vi "Q14070-Z060B.vi"() -> ()   [LabVIEW 2013]
uses:
  <vilib>/Utility/file.llb/Read From Spreadsheet File (string).vi
  <vilib>/express/express arith-compare/Formula/XNode/ExpressFormulaBlockNode.xnode
  PCI8622_32.dll
  <vilib>/printing/EasyPrintingControls.llb/contents.ctl
  <vilib>/Utility/NIReport.llb/NI_ReportGenerationCore.lvlib
  <vilib>/printing/EasyPrintingControls.llb/report_type.ctl
  <vilib>/Utility/NIReport.llb/NI_report.lvclass
  <vilib>/printing/EasyPrinting.llb/Easy Print VI Panel or Documentation (path).vi
panel:
  out "齿条跑和右极限":dbl format="%#.3f"
  out "齿条跑和左极限":dbl format="%#.3f"
  out "左轴向力数组大小":i32
  in  "电动缸快速":dbl=15.0
  in  "电动缸慢速":dbl=1.0
  out "最大轴向力标准(N)":dbl=200.0 caption="L+Lmax(mm)" format="%#.3f"
  out "循环退出":bool
  in  "?":bool
  in  "密码":string
  in  "?":bool
  in  "?":bool
  in  "截取百分比":dbl=0.05
  in  "半行程":dbl=70.0
  in  "是否取消放行按钮":bool
  out "PLC":bool
  out "齿条传动比":dbl=200.0 caption="L+Lmax(mm)" format="%#.3f"
  out "右平均轴向力(N)":dbl caption="L+Lmax(mm)" format="%#.3f"
  out "左平均轴向力(N)":dbl caption="最大位移偏离Lmax(mm)" format="%#.3f"
  in  "确定按钮":bool
  out "员工ID":string
  in  "出支线工步号":dbl
  out "报警提示":string
  in  "报警工步号":dbl
  out "急停":bool
  out "DeviceHandle":u32
  in  "轴向力设定次数":dbl=5.0
  in  "最小间隙(mm)":dbl=0.0005 format="%#.3f"
  out "本备料状态H":bool
  out "本测试状态H":bool
  out "本自动状态H":bool
  out "夹头松开":bool
  out "测头右位":bool
  out "测头左位":bool
  in  "测头气缸右移":bool
  in  "测头气缸左移":bool
  in  "轴向力已做次数":dbl
  out "轴向力及全行程间隙合格":bool
  out "轴向力启动":bool
  out "间隙启动":bool
  out "夹头夹紧位":bool
  in  "夹头松开":bool
  in  "夹头夹紧":bool
  out "找帽扭矩":dbl=5.0 caption="压力传感器" format="%#.2f"
  out "error out":errorcluster
  out "型号数量":i32
  out "error out 4":errorcluster
  in  "间隙设定调整次数":dbl=5.0
  out "读取产品ID":string
  in  "本备料状态":bool
  in  "本测试状态":bool
  in  "本自动状态":bool
  out "FGCS":string
  out "KSJJ":string
  out "Z060BRFID":string
  out "轴向力Y":dbl[](array[numeric])
  out "轴向力X":dbl[](array[numeric])
  out "间隙X数组":dbl[](array[numeric])
  out "间隙Y数组":dbl[](array[numeric])
  out "error out 3":errorcluster caption="错误输出"
  out "rfid工步号":u32
  out "芯片ID":string="201209190001"
  out "rfid完成":bool
  out "rfid触发":bool
  out "本序已做":bool
  in  "回零完成":bool
  in  "电动缸回零":bool
  in  "单点间隙已调试次数":dbl
  in  "需调整角度(度)":dbl
  in  "转向器中心":dbl
  out "扭矩到达":bool
  out "黄灯":bool
  out "红灯":bool
  out "基准位移":dbl caption="压力传感器" format="%#.4f"
  out "上序不合格":bool
  out "单点间隙合格":bool
  out "上序合格":bool
  out "测头机构电机":u32
  out "复位":bool
  in  "型号选择":u16(ring)=2 items=["J709", "J728", "J706"]
  in  "联线按钮":bool
  in  "工步号":u32
  in  "产品ID":string="201209190001"
  out "间隙位移(mm)":dbl=-4.6787895475327215 caption="压力传感器" format="%#.3f"
  out "齿条推拉力(N)":dbl format="%#.2f"
  out "齿条扭矩(Nm)":dbl format="%#.2f"
  out "通讯状态":bool
  out "员工姓名":string
  out "工步提示":string
  out "ADODB._Connection Out 2":refnum<k7>
  out "旋转齿条电机":u32
  out "电动缸电机":u32
  in  "停止":bool
  in  "参数加载":bool
  in  "选项卡控件":T1(tab)
  out "180°外全行程间隙标准(mm)":dbl=0.1 format="%#.3f"
  out "扭动曲线":cluster{"Y":dbl[], "Y":dbl[]}[](graph) caption="压球涨堵头1"
  out "中间位置间隙":dbl caption="间隙值L(mm)" format="%#.3f"
  out "中间位置最大间隙标准(mm)":dbl=0.07 format="%#.3f"
  out "右180°外全行程间隙":dbl caption="正向最大间隙L1(mm)" format="%#.3f"
  out "左180°外全行程间隙":dbl caption="正向最大间隙L1(mm)" format="%#.3f"
  out "右180°内全行程间隙":dbl caption="正向最大间隙L1(mm)" format="%#.3f"
  out "左180°内全行程间隙":dbl caption="正向最大间隙L1(mm)" format="%#.3f"
  out "180°内全行程间隙标准(mm)":dbl=0.07 format="%#.3f"
  in  "找帽OK":bool
  out "左全行程间隙":dbl caption="正向最大间隙L1(mm)" format="%#.3f"
  out "右全行程间隙":dbl caption="正向最大间隙L1(mm)" format="%#.3f"
  out "总圈数最大值":dbl
  out "总圈数标准":dbl
  out "总行程最大值":dbl
  out "总行程标准(mm)":dbl
  out "力波动标准(N)":dbl=60.0 caption="L+Lmax(mm)" format="%#.3f"
  out "轴向力标准(N)":dbl=100.0 caption="L+Lmax(mm)" format="%#.3f"
  out "右轴向力波动(N)":dbl caption="L+Lmax(mm)" format="%_4g"
  out "右最大轴向力(N)":dbl caption="L+Lmax(mm)" format="%_4g"
  out "左轴向力波动(N)":dbl caption="最大位移偏离Lmax(mm)" format="%_4g"
  out "左最大轴向力(N)":dbl caption="最大位移偏离Lmax(mm)" format="%_4g"
  out "行程跳动曲线":cluster{"Y":dbl[], "Y":dbl[]}[](graph) caption="压球涨堵头1"
  out "平均轴向力标准(N) max":dbl=200.0 caption="L+Lmax(mm)" format="%#.3f"
  out "总行程":dbl format="%_4g"
  out "总圈数":dbl format="%_4g"
  in  "不合格品":bool
  in  "扭矩停止值":dbl=16.0
  in  "齿条右极限":dbl=-70.0 caption="压力传感器" format="%#.2f"
  in  "齿条左极限":dbl=-262.0 caption="压力传感器" format="%#.2f"
  in  "齿条移动速度":dbl=5.0 caption="压力传感器" format="%#.2f"
  in  "旋转齿条轴找帽转速":dbl=5.0 caption="压力传感器" format="%#.2f"
  in  "测量点扭矩":dbl=4.0 caption="压力传感器" format="%#.2f"
  in  "旋转齿条轴测量转速":dbl caption="压力传感器" format="%#.2f"
  in  "测头机构轴后退位":dbl=30.0 caption="压力传感器" format="%#.2f"
  in  "测头机构轴待检位":dbl caption="压力传感器" format="%#.2f"
  in  "测头机构轴检测位":dbl caption="压力传感器" format="%#.2f"
  in  "测头机构轴移动速度":dbl caption="压力传感器" format="%#.2f"
  in  "机械间隙值":dbl=3.5
  in  "阻挡":bool
  in  "放行":bool
  in  "夹头松开":bool
  in  "夹头夹紧":bool
  in  "测头气缸右移":bool
  in  "测头气缸左移":bool
  in  "支线下降":bool
  in  "支线顶升":bool
  in  "出支线":bool
  in  "进支线":bool
  in  "主线下降":bool
  in  "主线顶升":bool
  in  "下阻挡器放行":bool
  in  "上阻挡器放行":bool
  in  "测头机构轴使能":bool
  in  "测头机构轴后退":bool
  in  "测头机构轴前进":bool
  in  "电动缸速度(mm/s)":dbl=10.0 format="%#.3f"
  out "电动缸位置(mm)":dbl format="%#.3f"
  in  "旋转齿条轴速度(°/s)":dbl=10.0 format="%#.3f"
  out "旋转齿条轴位置(°)":dbl format="%#.3f"
  in  "测头机构轴速度(mm/s)":dbl=10.0 format="%#.3f"
  out "测头机构轴位置(mm)":dbl format="%#.3f"
  in  "旋转齿条轴右转":bool
  in  "旋转齿条轴左转":bool
  in  "旋转齿条轴使能":bool
  in  "电动缸后退":bool
  in  "电动缸使能":bool
  in  "电动缸前进":bool
  in  "齿条扭矩比例偏移":dbl=1.0 format="%#.2f"
  in  "齿条扭矩零点偏移":dbl format="%#.2f"
  in  "齿条推拉力比例偏移":dbl=1.0 format="%#.2f"
  in  "齿条推拉力零点偏移":dbl format="%#.2f"
  in  "间隙位移比例偏移":dbl=1.0 format="%#.2f"
  in  "间隙位移零点偏移":dbl format="%#.2f"
  in  "传感器参数保存":bool
  in  "参数修改":bool
  in  "参数查询":bool
  in  "参数浏览表":string[][](table)
  # "芜湖机械转向器装配线"
  # "间隙及轴向力检测"
  # "湖北唯思凌科装备制造有限公司 设计开发 (C)2015"
  # "Q14070机械转向器装配线"
  # "≤"
  # "间隙测量结果"
  # "间隙测量判定值"
  # "≤"
  # "≤"
  # "≤"
  # "轴向力测量结果"
  # "轴向力测量标准"
  # "≥"
  # "≤"
  # "≥"
  # "≤"
  # "≤"
  # "≥"
  # "不得大于20NM"
  # "传感器校验区"
  # "关于传感器校验：\n1、传感器校验需要由具备资质的单位或部门进行校验。\n2、具备权限的用户才能够修改传感器校验参数和试验参数。\n3、修改校验参数方法：先将比例偏移置为1，修改零点偏移，使零点值与校验的传感器一致；然后根据增幅调整比例偏移。"
  # "注意：\n具备权限的用户才能够修改传感器校验参数和试验参数！"
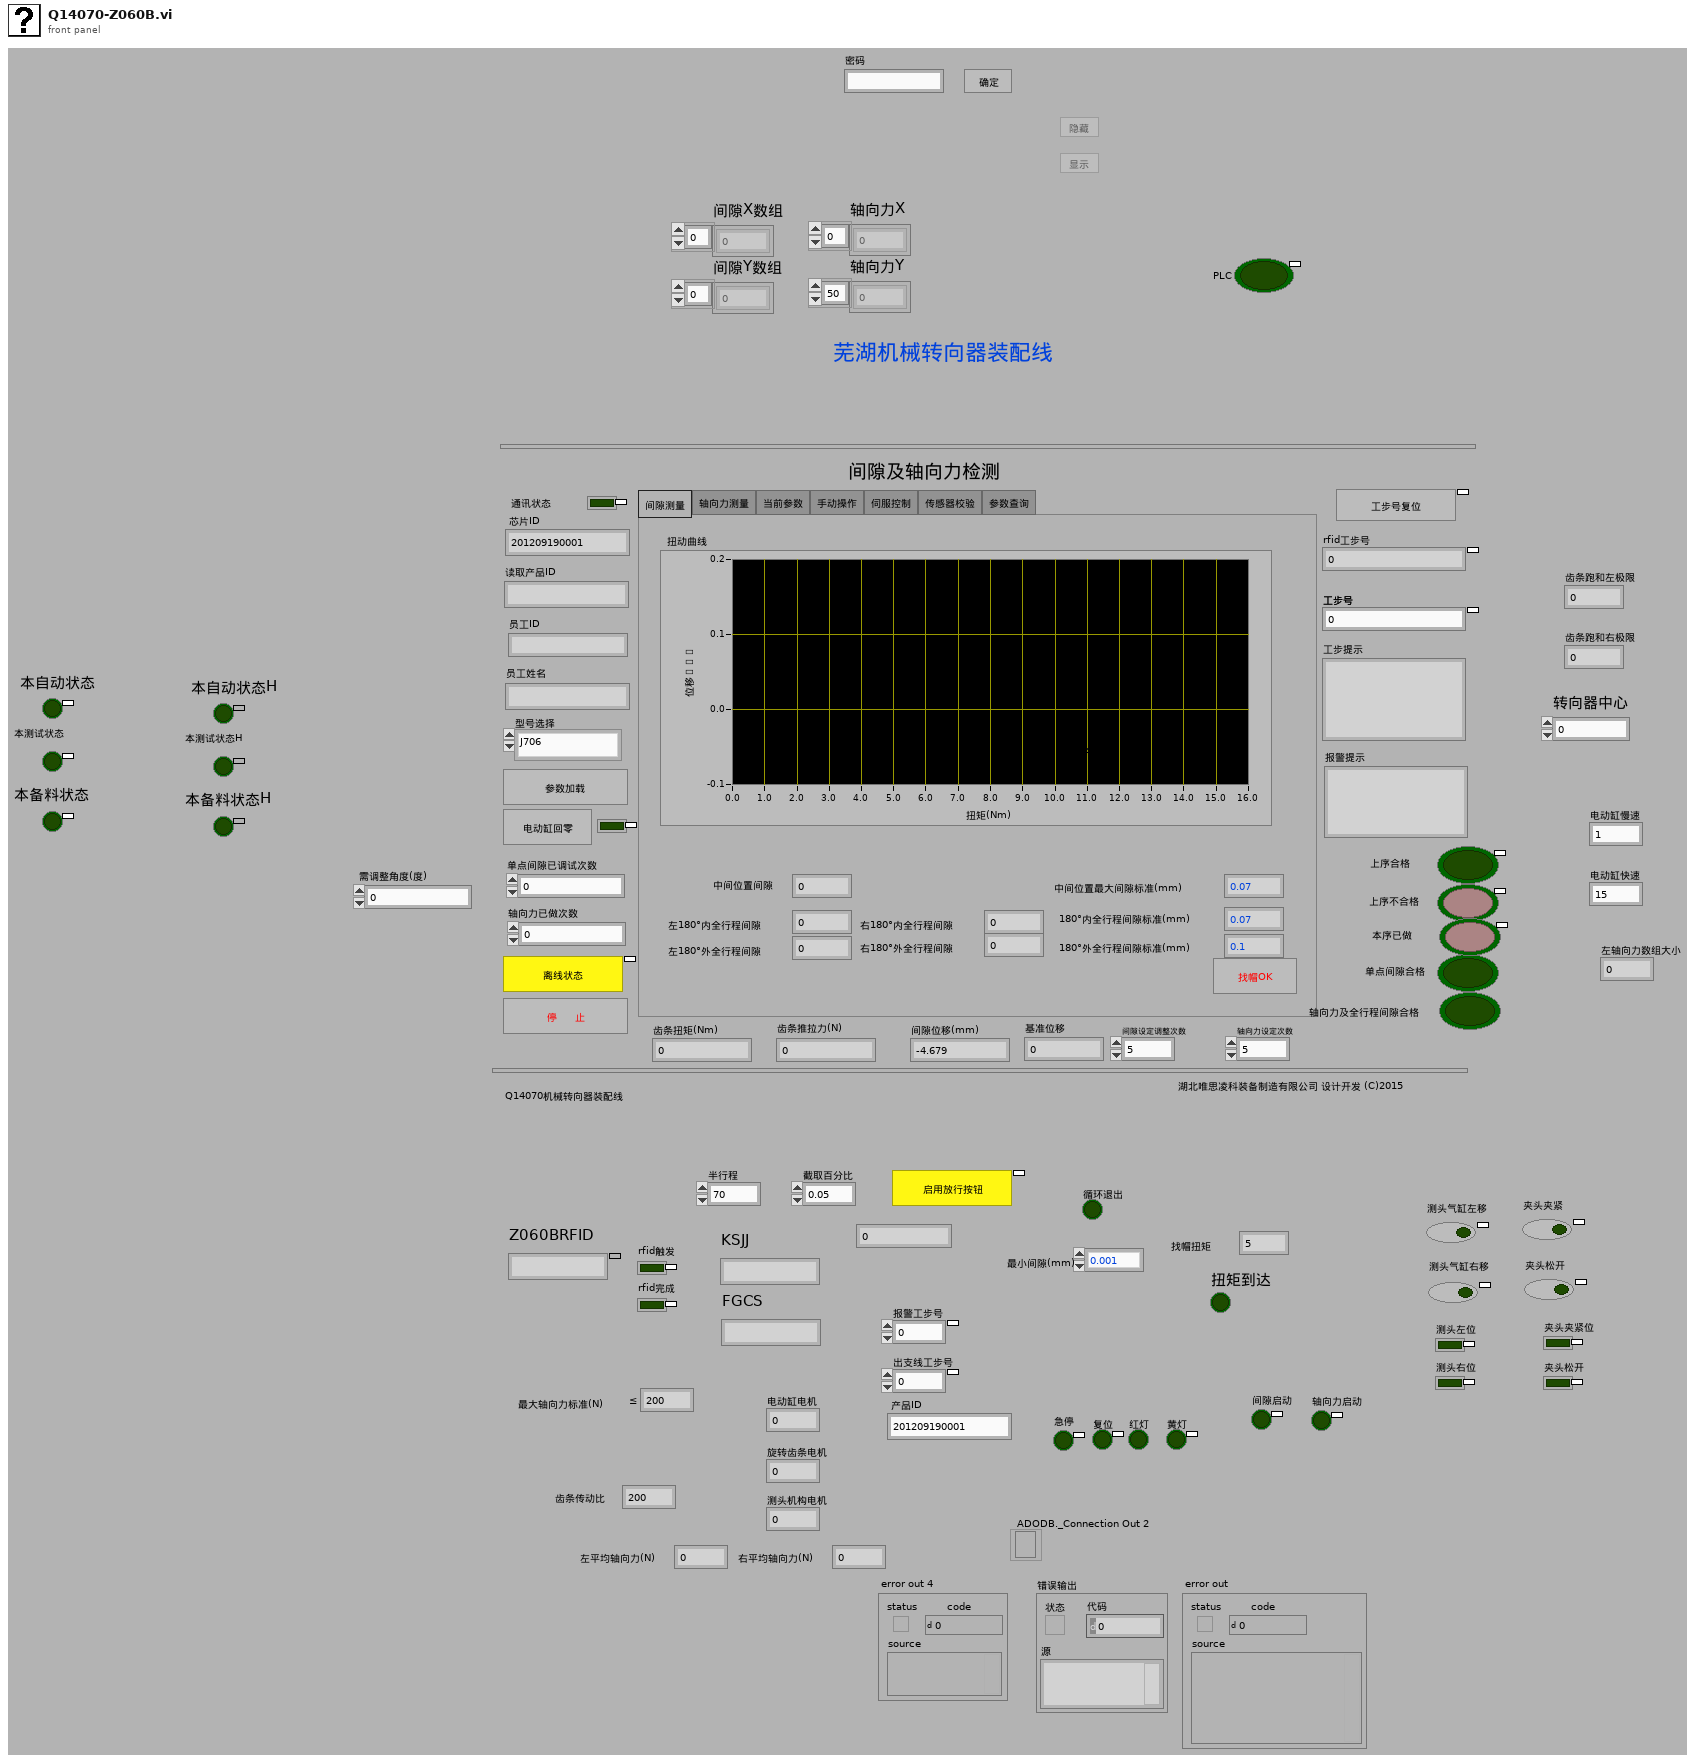
[diagram p1: front panel]
types:
  T1 = enum32{"间隙测量", "轴向力测量", "当前参数", "手动操作", "伺服控制", "传感器校验", "参数查询"}
  T2 = typedef "NI_ReportGenerationCore.lvlib/report_type.ctl" = u16
  T3 = typedef "NI_ReportGenerationCore.lvlib/contents.ctl" = u16
  T4 = typedef "imagedata.ctl" = cluster{"image type":i32, "image depth":i32, "image":u8[], "mask":u8[], "colors":u32[], "Rectangle":cluster{"left":i16, "top":i16, "right":i16, "bottom":i16}}
  T5 = enum8{"Enabled", "Disabled", "Disabled and Grayed Out"}
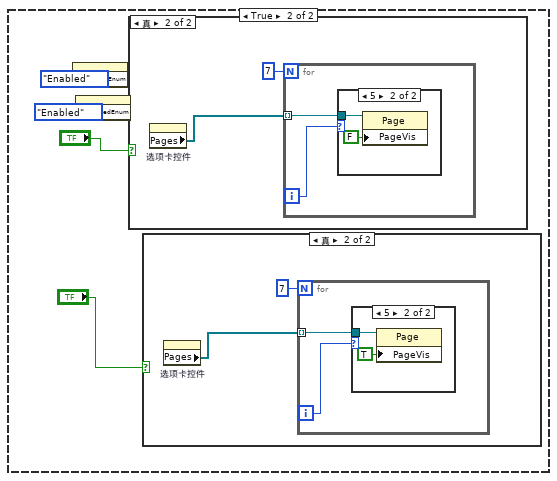
[diagram p2: hidden frame]
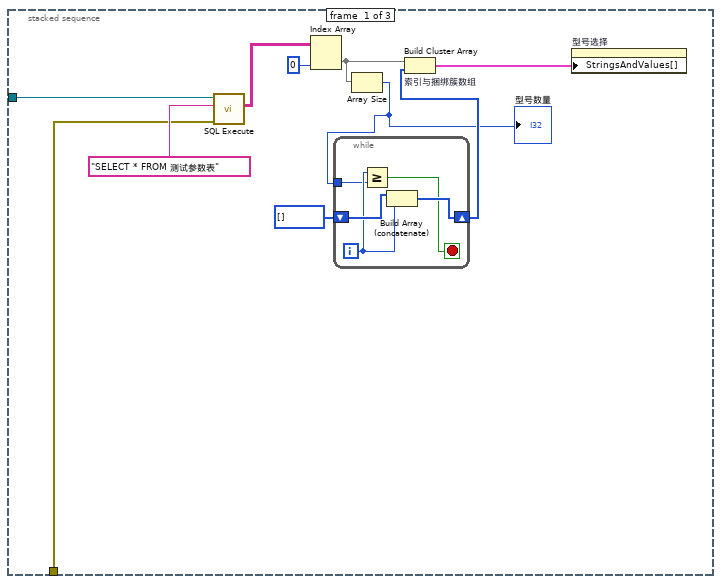
[diagram p9: hidden frame]
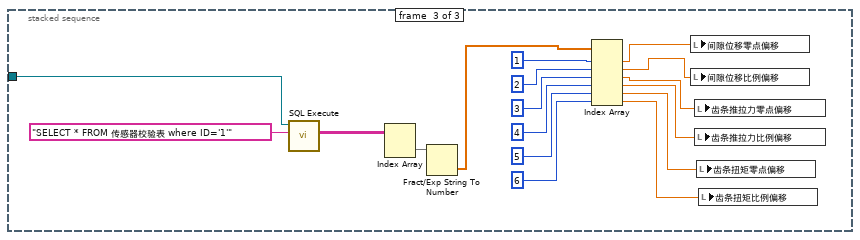
[diagram p10: hidden frame]
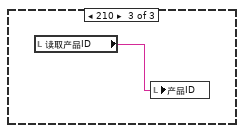
[diagram p12: hidden frame]
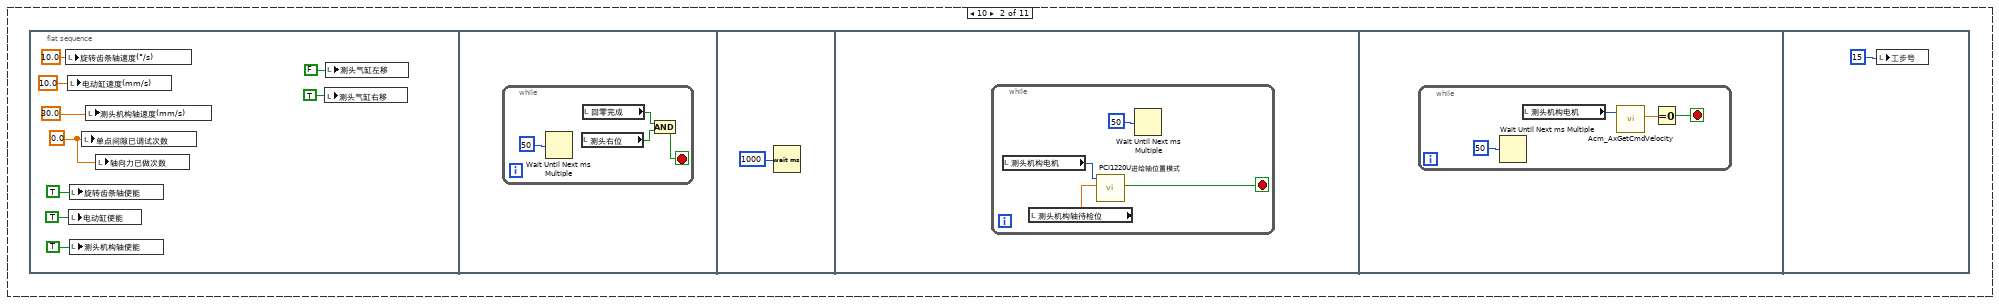
[diagram p14: hidden frame]
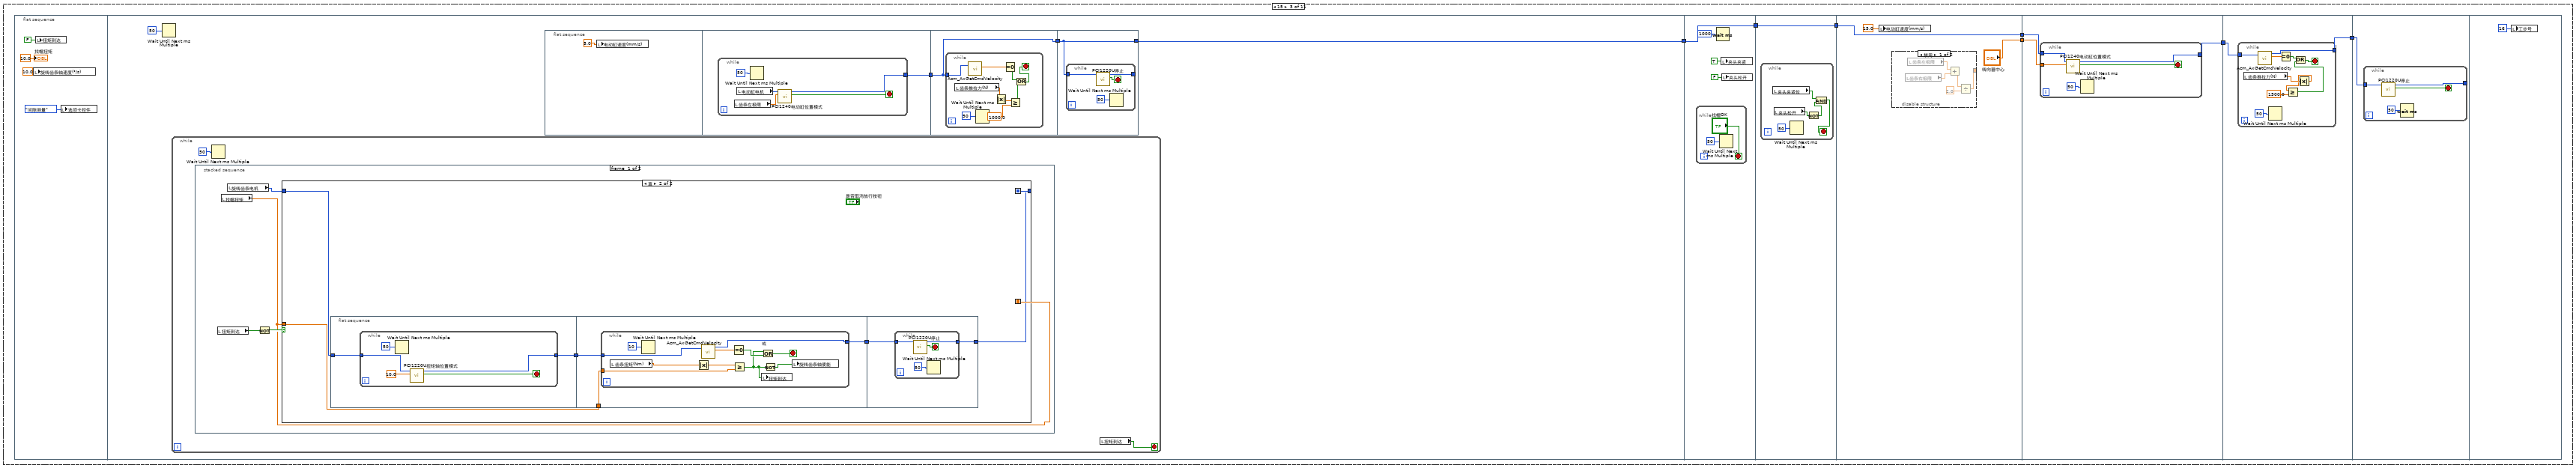
[diagram p15: hidden frame]
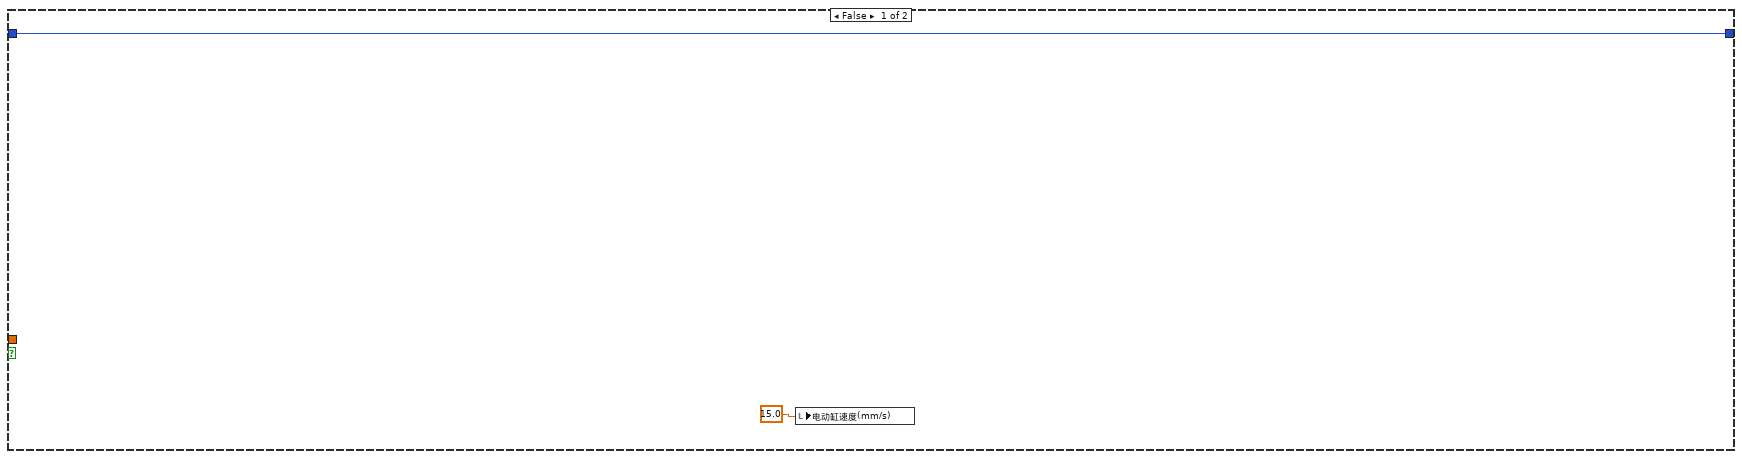
[diagram p16: hidden frame]
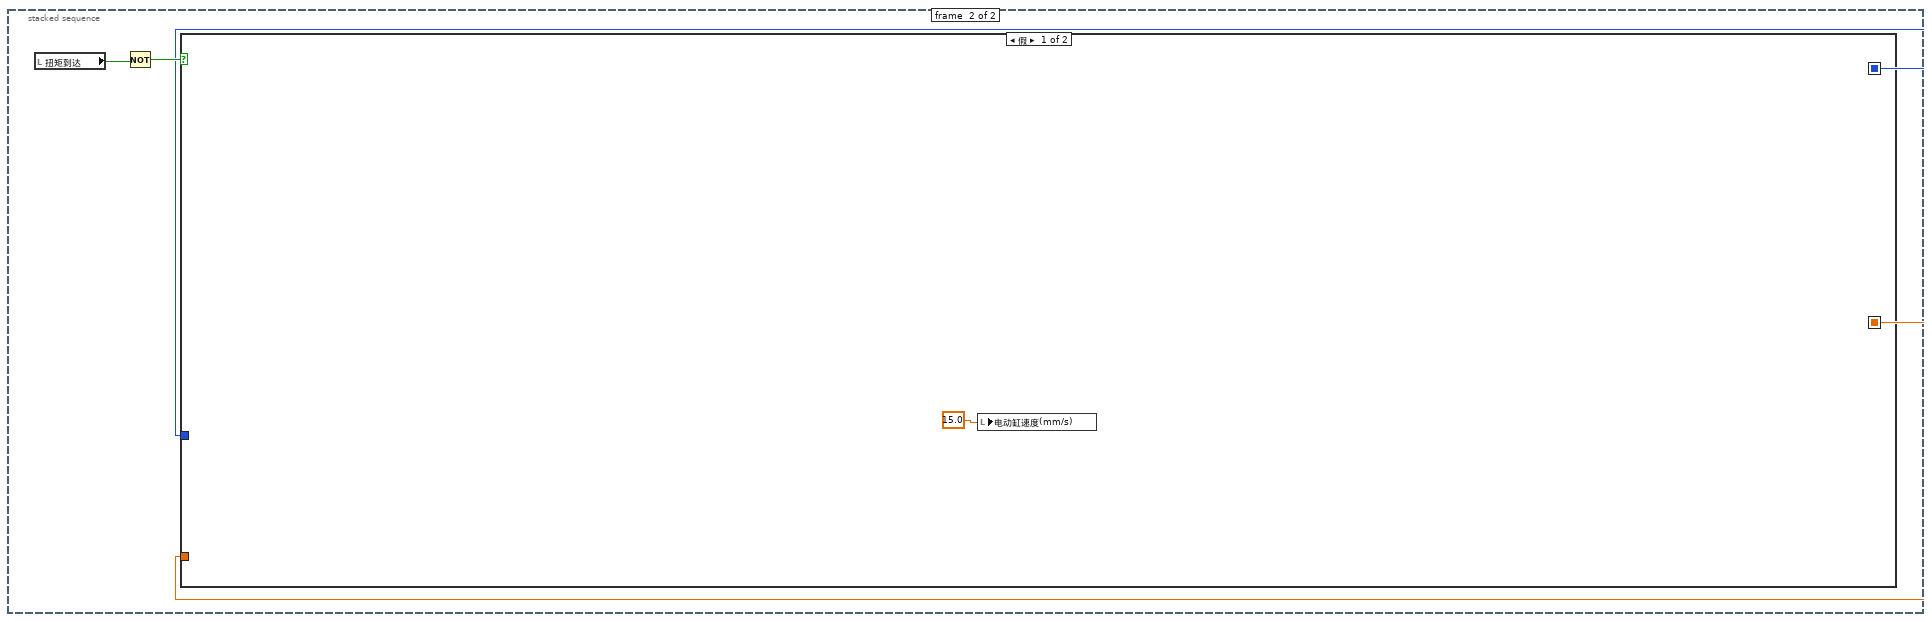
[diagram p17: hidden frame]
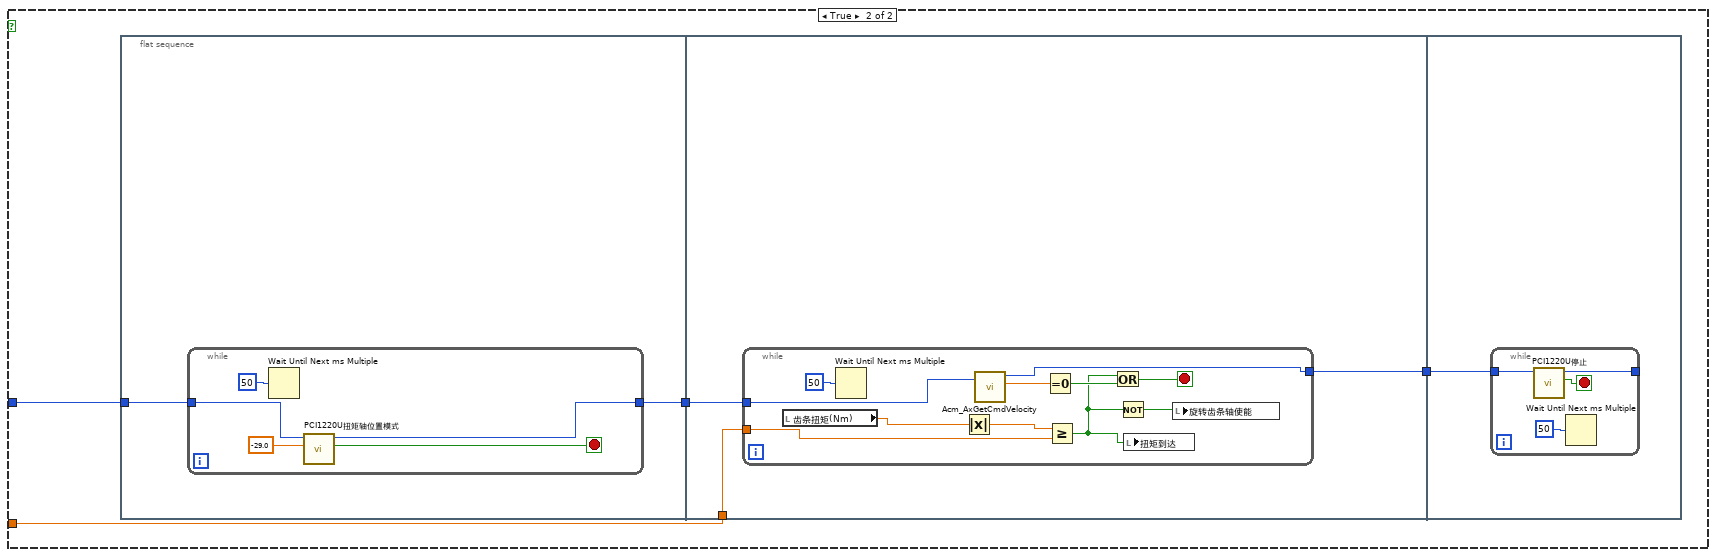
[diagram p18: hidden frame]
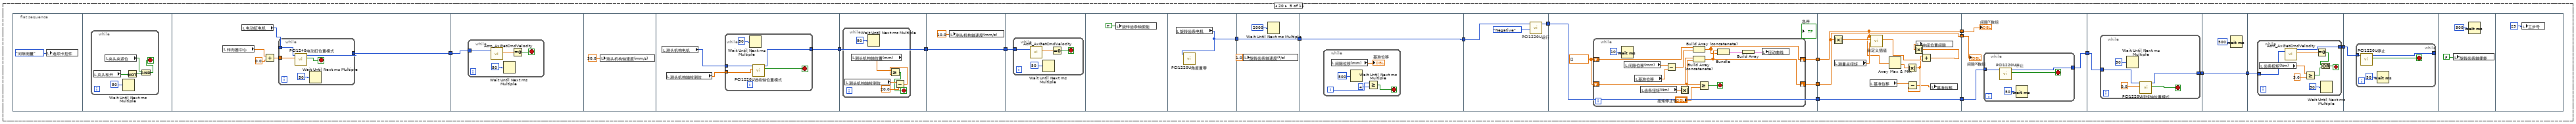
[diagram p20: hidden frame]
diagram:
  n1 = while {
    stop <- w7 stop-if-true
    n2 = local read "工步号"() -> (w5:u32)
    n3 = case shown="16" w5 {
      frame 0, Default {
      }
      frame 10 {
        n4 = flat-sequence {
          frame #0 {
            w8 = 0.0 ("已调试次数")
            n5 = local write "旋转齿条轴速度(°/s)"(10.0 ("旋转齿条轴速度(°/s)")) -> ()
            n6 = local write "电动缸速度(mm/s)"(10.0 ("电动缸速度(mm/s)")) -> ()
            n7 = local write "电动缸使能"(TRUE ("电动缸使能")) -> ()
            n8 = local write "旋转齿条轴使能"(TRUE ("旋转齿条轴使能")) -> ()
            n9 = local write "测头机构轴使能"(TRUE ("调整机构轴使能")) -> ()
            n10 = local write "单点间隙已调试次数"(w8) -> ()
            n11 = local write "测头机构轴速度(mm/s)"(30.0 ("调整机构轴速度(mm/s)")) -> ()
            n12 = local write "轴向力已做次数"(w8) -> ()
            n13 = local write "测头气缸右移"(TRUE ("测头气缸右移")) -> ()
            n14 = local write "测头气缸左移"(FALSE ("测头气缸左移")) -> ()
          }
          frame #1 {
            n15 = while {
              stop <- w17 stop-if-true
              n16 = Wait Until Next ms Multiple(millisecond multiple=u32 50 ("毫秒倍数")) -> ()  [unwired: 1 out]
              n17 = local read "测头右位"() -> (w18:bool)
              n18 = local read "回零完成"() -> (w19:bool)
              n19 = And(x=w19, y=w18) -> (x .and. y?=w17:bool)
            }
          }
          frame #2 {
            n20 = Wait (ms)(milliseconds to wait=u32 1000 ("等待时间（毫秒）")) -> ()  [unwired: 1 out]
          }
          frame #3 {
            n21 = while {
              stop <- w25 stop-if-true
              n22 = local read "测头机构电机"() -> (w23:u32)
              n23 = local read "测头机构轴待检位"() -> (w22:dbl)
              n24 = call "PCI1220U进给轴位置模式.vi"("Distance"=w22, "AxisHandle IN"=w23) -> ("AbsSuccess"=w25:bool)  [unwired: 8 in, 1 out]
              n25 = Wait Until Next ms Multiple(millisecond multiple=u32 50 ("毫秒倍数")) -> ()  [unwired: 1 out]
            }
          }
          frame #4 {
            n26 = while {
              stop <- w28 stop-if-true
              n27 = Wait Until Next ms Multiple(millisecond multiple=u32 50 ("毫秒倍数")) -> ()  [unwired: 1 out]
              n28 = local read "测头机构电机"() -> (w26:u32)
              n29 = call <userlib>:"Acm_AxGetCmdVelocity.vi"("AxisHandle"=w26) -> ("Velocity"=w29:dbl)  [unwired: 1 in, 3 out]
              n30 = Equal To 0?(x=w29) -> (x = 0?=w28:bool)
            }
          }
          frame #5 {
            n31 = local write "工步号"(u32 15 ("工步号")) -> ()
          }
        }
      }
      frame 15 {
        n32 = flat-sequence {
          tunnel: [w43] -> w34
          tunnel: w34 -> [w146]
          tunnel: [w146] -> w32
          tunnel: w32 -> [w150]
          tunnel: [w150] -> w31
          tunnel: [w157] -> w37
          tunnel: ["转向器中心"] -> w36
          tunnel: w31 -> [w157]
          tunnel: w37 -> [w166]
          tunnel: w36 -> [w165]
          tunnel: [w164] -> w35
          tunnel: w35 -> [w173]
          tunnel: [w172] -> w33
          tunnel: w33 -> [w184]
          frame #0 {
            n33 = local write "旋转齿条轴速度(°/s)"(10.0 ("旋转齿条轴速度(°/s)")) -> ()
            n34 = local write "扭矩到达"(FALSE ("扭矩到达")) -> ()
            n35 = local write "选项卡控件"(T1."间隙测量" ("选项卡控件")) -> ()
            "找帽扭矩" <- 10.0 ("找帽扭矩")
          }
          frame #1 {
            n36 = Wait Until Next ms Multiple(millisecond multiple=u32 50 ("毫秒倍数")) -> ()  [unwired: 1 out]
            n37 = while {
              stop <- w46 stop-if-true
              n38 = stacked-sequence {
                seq-local: [w48 _] -> [_ w89]
                seq-local: [w52 _] -> [_ w88]
                frame #0 {
                  n39 = local read "扭矩到达"() -> (w50:bool)
                  n40 = local read "找帽扭矩"() -> (w48:dbl)
                  n41 = local read "旋转齿条电机"() -> (w49:u32)
                  n42 = Not(x=w50) -> (.not. x?=w51:bool)
                  n43 = case shown="真" w51 {
                    tunnel: [w54 w55] -> w52
                    tunnel: w49 -> [w54 w59]
                    tunnel: w48 -> [_ w57]
                    frame False {
                      n44 = local write "电动缸速度(mm/s)"(15.0 ("电动缸速度(mm/s)")) -> ()
                    }
                    frame True {
                      n45 = flat-sequence {
                        tunnel: w59 -> [w61]
                        tunnel: [w60] -> w58
                        tunnel: w58 -> [w69]
                        tunnel: w57 -> [w68]
                        tunnel: [w67] -> w56
                        tunnel: w56 -> [w82]
                        tunnel: [w81] -> w55
                        frame #0 {
                          n46 = while {
                            tunnel: [w65] -> w60
                            tunnel: w61 -> [w62]
                            stop <- w64 stop-if-true
                            n47 = Wait Until Next ms Multiple(millisecond multiple=u32 50 ("毫秒倍数")) -> ()  [unwired: 1 out]
                            n48 = call "PCI1220U扭矩轴位置模式.vi"("Distance"=10.0, "AxisHandle IN"=w62) -> ("AbsSuccess"=w64:bool, "AxisHandle OUT"=w65:u32)  [unwired: 8 in]
                          }
                        }
                        frame #1 {
                          n49 = while {
                            tunnel: w69 -> [w79]
                            tunnel: w68 -> [w74]
                            tunnel: [w73] -> w67
                            stop <- w75 stop-if-true
                            n50 = local read "齿条扭矩(Nm)"() -> (w72:dbl)
                            n51 = Wait Until Next ms Multiple(millisecond multiple=u32 10 ("毫秒倍数")) -> ()  [unwired: 1 out]
                            n52 = Absolute Value(x=w72) -> (abs(x)=w77:dbl)
                            n53 = call <userlib>:"Acm_AxGetCmdVelocity.vi"("AxisHandle"=w79) -> ("Velocity"=w78:dbl, "AxisHandle"=w73:u32)  [unwired: 1 in, 2 out]
                            n54 = Equal To 0?(x=w78) -> (x = 0?=w76:bool)
                            n55 = Greater Or Equal?(x=w77, y=w74) -> (x >= y?=w71:bool)
                            n56 = Or "或"(x=w71, y=w76) -> (x .or. y?=w75:bool)
                            n57 = local write "扭矩到达"(w71) -> ()
                            n58 = Not(x=w71) -> (.not. x?=w70:bool)
                            n59 = local write "旋转齿条轴使能"(w70) -> ()
                          }
                        }
                        frame #2 {
                          n60 = while {
                            tunnel: w82 -> [w86]
                            tunnel: [w83] -> w81
                            stop <- w85 stop-if-true
                            n61 = call "PCI1220U停止.vi"("AxisHandle IN"=w86) -> ("完成"=w85:bool, "AxisHandle OUT"=w83:u32)  [unwired: 9 in]
                            n62 = Wait Until Next ms Multiple(millisecond multiple=u32 50 ("毫秒倍数")) -> ()  [unwired: 1 out]
                          }
                        }
                      }
                    }
                  }
                }
                frame #1 {
                  n63 = local read "扭矩到达"() -> (w87:bool)
                  n64 = Not(x=w87) -> (.not. x?=w90:bool)
                  n65 = case shown="假" w90 {
                    tunnel: w88 -> [_ w95]
                    tunnel: w89 -> [_ w93]
                    frame False {
                      n66 = local write "电动缸速度(mm/s)"(15.0 ("电动缸速度(mm/s)")) -> ()
                    }
                    frame True {
                      n67 = flat-sequence {
                        tunnel: w95 -> [w96]
                        tunnel: [w97] -> w94
                        tunnel: w94 -> [w105]
                        tunnel: w93 -> [w104]
                        tunnel: [w103] -> w92
                        tunnel: w92 -> [w117]
                        frame #0 {
                          n68 = while {
                            tunnel: [w101] -> w97
                            tunnel: w96 -> [w98]
                            stop <- w100 stop-if-true
                            n69 = Wait Until Next ms Multiple(millisecond multiple=u32 50 ("毫秒倍数")) -> ()  [unwired: 1 out]
                            n70 = call "PCI1220U扭矩轴位置模式.vi"("Distance"=-29.0, "AxisHandle IN"=w98) -> ("AbsSuccess"=w100:bool, "AxisHandle OUT"=w101:u32)  [unwired: 8 in]
                          }
                        }
                        frame #1 {
                          n71 = while {
                            tunnel: w105 -> [w115]
                            tunnel: [w110] -> w103
                            tunnel: w104 -> [w109]
                            stop <- w111 stop-if-true
                            n72 = local read "齿条扭矩(Nm)"() -> (w108:dbl)
                            n73 = Wait Until Next ms Multiple(millisecond multiple=u32 50 ("毫秒倍数")) -> ()  [unwired: 1 out]
                            n74 = Absolute Value(x=w108) -> (abs(x)=w113:dbl)
                            n75 = call <userlib>:"Acm_AxGetCmdVelocity.vi"("AxisHandle"=w115) -> ("Velocity"=w114:dbl, "AxisHandle"=w110:u32)  [unwired: 1 in, 2 out]
                            n76 = Equal To 0?(x=w114) -> (x = 0?=w112:bool)
                            n77 = Greater Or Equal?(x=w113, y=w109) -> (x >= y?=w106:bool)
                            n78 = Or(x=w106, y=w112) -> (x .or. y?=w111:bool)
                            n79 = Not(x=w106) -> (.not. x?=w107:bool)
                            n80 = local write "扭矩到达"(w106) -> ()
                            n81 = local write "旋转齿条轴使能"(w107) -> ()
                          }
                        }
                        frame #2 {
                          n82 = while {
                            tunnel: w117 -> [w121]
                            tunnel: [w118] -> _
                            stop <- w120 stop-if-true
                            n83 = call "PCI1220U停止.vi"("AxisHandle IN"=w121) -> ("完成"=w120:bool, "AxisHandle OUT"=w118:u32)  [unwired: 9 in]
                            n84 = Wait Until Next ms Multiple(millisecond multiple=u32 50 ("毫秒倍数")) -> ()  [unwired: 1 out]
                          }
                        }
                      }
                    }
                  }
                }
              }
              n85 = Wait Until Next ms Multiple(millisecond multiple=u32 50 ("毫秒倍数")) -> ()  [unwired: 1 out]
              n86 = local read "扭矩到达"() -> (w46:bool)
            }
            n87 = flat-sequence {
              tunnel: [w123] -> w45
              tunnel: w45 -> [w129]
              tunnel: [w129] -> w42
              tunnel: [w139] -> w43
              tunnel: w42 -> [w139]
              frame #0 {
                n88 = local write "电动缸速度(mm/s)"(5.0 ("电动缸速度(mm/s)")) -> ()
              }
              frame #1 {
                n89 = while {
                  tunnel: [w127] -> w123
                  stop <- w126 stop-if-true
                  n90 = local read "齿条左极限"() -> (w124:dbl)
                  n91 = local read "电动缸电机"() -> (w128:u32)
                  n92 = Wait Until Next ms Multiple(millisecond multiple=u32 50 ("毫秒倍数")) -> ()  [unwired: 1 out]
                  n93 = call "PCI1240电动缸位置模式 .vi"("Distance"=w124, "AxisHandle IN"=w128) -> ("AbsSuccess"=w126:bool, "AxisHandle OUT"=w127:u32)  [unwired: 8 in]
                }
              }
              frame #2 {
                n94 = while {
                  tunnel: w129 -> [w137]
                  stop <- w134 stop-if-true
                  n95 = local read "齿条推拉力(N)"() -> (w133:dbl)
                  n96 = call <userlib>:"Acm_AxGetCmdVelocity.vi"("AxisHandle"=w137) -> ("Velocity"=w138:dbl)  [unwired: 1 in, 3 out]
                  n97 = Wait Until Next ms Multiple(millisecond multiple=u32 50 ("毫秒倍数")) -> ()  [unwired: 1 out]
                  n98 = Absolute Value(x=w133) -> (abs(x)=w130:dbl)
                  n99 = Equal To 0?(x=w138) -> (x = 0?=w135:bool)
                  n100 = Greater Or Equal?(x=w130, y=1000.0) -> (x >= y?=w131:bool)
                  n101 = Or(x=w135, y=w131) -> (x .or. y?=w134:bool)
                }
              }
              frame #3 {
                n102 = while {
                  tunnel: w139 -> [w143]
                  tunnel: [w140] -> _
                  stop <- w142 stop-if-true
                  n103 = call "PCI1220U停止.vi"("AxisHandle IN"=w143) -> ("完成"=w142:bool, "AxisHandle OUT"=w140:u32)  [unwired: 9 in]
                  n104 = Wait Until Next ms Multiple(millisecond multiple=u32 50 ("毫秒倍数")) -> ()  [unwired: 1 out]
                }
              }
            }
          }
          frame #2 {
            n105 = while {
              stop <- "找帽OK" stop-if-true
              n106 = Wait Until Next ms Multiple(millisecond multiple=u32 50 ("毫秒倍数")) -> ()  [unwired: 1 out]
            }
            n107 = Wait (ms)(milliseconds to wait=u32 1000 ("毫秒倍数")) -> ()  [unwired: 1 out]
            n108 = local write "夹头夹紧"(TRUE ("夹头夹紧")) -> ()
            n109 = local write "夹头松开"(FALSE ("夹头松开")) -> ()
          }
          frame #3 {
            n110 = while {
              stop <- w152 stop-if-true
              n111 = local read "夹头夹紧位"() -> (w153:bool)
              n112 = local read "夹头松开"() -> (w155:bool)
              n113 = Wait Until Next ms Multiple(millisecond multiple=u32 50 ("毫秒倍数")) -> ()  [unwired: 1 out]
              n114 = Not(x=w155) -> (.not. x?=w154:bool)
              n115 = And(x=w153, y=w154) -> (x .and. y?=w152:bool)
            }
          }
          frame #4 {
            n116 = local write "电动缸速度(mm/s)"(15.0 ("电动缸轴移动速度")) -> ()
            n117 = disable-structure shown="禁用" {
              disable-tunnel: [w159 _] -> _
              frame Disabled {
                n118 = local read "齿条右极限"() -> (w162:dbl)
                n119 = local read "齿条左极限"() -> (w163:dbl)
                n120 = Add(x=w163, y=w162) -> (x+y=w161:dbl)
                n121 = Divide(x=w161, y=2.0) -> (x/y=w159:dbl)
              }
              frame Enabled {
              }
            }
          }
          frame #5 {
            n122 = while {
              tunnel: w166 -> [w171]
              tunnel: w165 -> [w170]
              tunnel: [w167] -> w164
              stop <- w169 stop-if-true
              n123 = call "PCI1240电动缸位置模式 .vi"("Distance"=w170, "AxisHandle IN"=w171) -> ("AbsSuccess"=w169:bool, "AxisHandle OUT"=w167:u32)  [unwired: 8 in]
              n124 = Wait Until Next ms Multiple(millisecond multiple=u32 50 ("毫秒倍数")) -> ()  [unwired: 1 out]
            }
          }
          frame #6 {
            n125 = while {
              tunnel: w173 -> [w183]
              tunnel: [w174] -> w172
              stop <- w175 stop-if-true
              n126 = local read "齿条推拉力(N)"() -> (w180:dbl)
              n127 = call <userlib>:"Acm_AxGetCmdVelocity.vi"("AxisHandle"=w183) -> ("Velocity"=w182:dbl, "AxisHandle"=w174:u32)  [unwired: 1 in, 2 out]
              n128 = Wait Until Next ms Multiple(millisecond multiple=u32 50 ("毫秒倍数")) -> ()  [unwired: 1 out]
              n129 = Equal To 0?(x=w182) -> (x = 0?=w177:bool)
              n130 = Absolute Value(x=w180) -> (abs(x)=w179:dbl)
              n131 = Greater Or Equal?(x=w179, y=1500.0) -> (x >= y?=w176:bool)
              n132 = Or(x=w177, y=w176) -> (x .or. y?=w175:bool)
            }
          }
          frame #7 {
            n133 = while {
              tunnel: w184 -> [w188]
              tunnel: [w187] -> _
              stop <- w186 stop-if-true
              n134 = call "PCI1220U停止.vi"("AxisHandle IN"=w188) -> ("完成"=w186:bool, "AxisHandle OUT"=w187:u32)  [unwired: 9 in]
              n135 = Wait (ms)(milliseconds to wait=u32 50 ("毫秒倍数")) -> ()  [unwired: 1 out]
            }
          }
          frame #8 {
            n136 = local write "工步号"(u32 16 ("工步号")) -> ()
          }
        }
      }
      frame 16 {
        n137 = flat-sequence {
          tunnel: [w203] -> w200
          tunnel: w200 -> [w210]
          tunnel: [w209] -> w199
          tunnel: w199 -> [w221]
          tunnel: [w223] -> w198
          tunnel: w198 -> [w232]
          tunnel: [w231] -> w197
          tunnel: w197 -> [w244]
          tunnel: [w246] -> w196
          tunnel: w196 -> [w253]
          tunnel: [w252] -> w195
          tunnel: w195 -> [w263]
          tunnel: [w266] -> w194
          tunnel: w194 -> [w275]
          tunnel: [w274] -> w193
          tunnel: w193 -> [w287]
          tunnel: [w286] -> w192
          tunnel: w192 -> [w292]
          tunnel: [w296] -> w191
          tunnel: w191 -> [w298]
          tunnel: [w297] -> w190
          tunnel: w190 -> [w309]
          frame #0 {
            n138 = local write "电动缸速度(mm/s)"(30.0 ("齿条移动速度")) -> ()
          }
          frame #1 {
            n139 = Wait (ms)(milliseconds to wait=u32 100 ("等待时间（毫秒）")) -> ()  [unwired: 1 out]
          }
          frame #2 {
            n140 = while {
              tunnel: [w206] -> w203
              stop <- w208 stop-if-true
              n141 = local read "电动缸电机"() -> (w205:u32)
              n142 = local read "齿条左极限"() -> (w204:dbl)
              n143 = Wait Until Next ms Multiple(millisecond multiple=u32 50 ("毫秒倍数")) -> ()  [unwired: 1 out]
              n144 = call "PCI1240电动缸位置模式 .vi"("Distance"=w204, "AxisHandle IN"=w205) -> ("AbsSuccess"=w208:bool, "AxisHandle OUT"=w206:u32)  [unwired: 8 in]
            }
          }
          frame #3 {
            n145 = while {
              tunnel: w210 -> [w219]
              tunnel: [w212] -> w209
              stop <- w213 stop-if-true
              n146 = local read "齿条推拉力(N)"() -> (w211:dbl)
              n147 = Wait Until Next ms Multiple(millisecond multiple=u32 50 ("毫秒倍数")) -> ()  [unwired: 1 out]
              n148 = call <userlib>:"Acm_AxGetCmdVelocity.vi"("AxisHandle"=w219) -> ("Velocity"=w218:dbl, "AxisHandle"=w212:u32)  [unwired: 1 in, 2 out]
              n149 = Less Or Equal?(x=w211, y=-500.0) -> (x <= y?=w214:bool)
              n150 = Equal To 0?(x=w218) -> (x = 0?=w215:bool)
              n151 = Or(x=w215, y=w214) -> (x .or. y?=w213:bool)
            }
          }
          frame #4 {
            n152 = call "PCI1220U停止.vi"("AxisHandle IN"=w221) -> ()  [unwired: 9 in, 2 out]
            n153 = local write "电动缸速度(mm/s)"(1.0 ("齿条移动速度")) -> ()
          }
          frame #5 {
            n154 = Wait (ms)(milliseconds to wait=u32 100 ("等待时间（毫秒）")) -> ()  [unwired: 1 out]
          }
          frame #6 {
            n155 = while {
              tunnel: [w228] -> w223
              stop <- w230 stop-if-true
              n156 = local read "齿条左极限"() -> (w226:dbl)
              n157 = Wait Until Next ms Multiple(millisecond multiple=u32 50 ("毫秒倍数")) -> ()  [unwired: 1 out]
              n158 = local read "电动缸电机"() -> (w227:u32)
              n159 = Add(x=w226, y=30.0) -> (x+y=w224:dbl)
              n160 = call "PCI1240电动缸位置模式 .vi"("Distance"=w224, "AxisHandle IN"=w227) -> ("AbsSuccess"=w230:bool, "AxisHandle OUT"=w228:u32)  [unwired: 8 in]
            }
          }
          frame #7 {
            n161 = while {
              tunnel: w232 -> [w241]
              tunnel: [w234] -> w231
              stop <- w235 stop-if-true
              n162 = local read "齿条推拉力(N)"() -> (w233:dbl)
              n163 = Wait Until Next ms Multiple(millisecond multiple=u32 50 ("毫秒倍数")) -> ()  [unwired: 1 out]
              n164 = call <userlib>:"Acm_AxGetCmdVelocity.vi"("AxisHandle"=w241) -> ("Velocity"=w240:dbl, "AxisHandle"=w234:u32)  [unwired: 1 in, 2 out]
              n165 = Less Or Equal?(x=w233, y=-500.0) -> (x <= y?=w236:bool)
              n166 = Equal To 0?(x=w240) -> (x = 0?=w237:bool)
              n167 = Or(x=w237, y=w236) -> (x .or. y?=w235:bool)
            }
          }
          frame #8 {
            n168 = local read "电动缸位置(mm)"() -> (→"齿条跑和左极限":dbl)
            n169 = call "PCI1220U停止.vi"("AxisHandle IN"=w244) -> ()  [unwired: 9 in, 2 out]
            n170 = local write "电动缸速度(mm/s)"(30.0 ("齿条移动速度")) -> ()
          }
          frame #9 {
            n171 = Wait (ms)(milliseconds to wait=u32 100 ("等待时间（毫秒）")) -> ()  [unwired: 1 out]
          }
          frame #10 {
            n172 = while {
              tunnel: [w249] -> w246
              stop <- w251 stop-if-true
              n173 = local read "电动缸电机"() -> (w248:u32)
              n174 = local read "齿条右极限"() -> (w247:dbl)
              n175 = Wait Until Next ms Multiple(millisecond multiple=u32 50 ("毫秒倍数")) -> ()  [unwired: 1 out]
              n176 = call "PCI1240电动缸位置模式 .vi"("Distance"=w247, "AxisHandle IN"=w248) -> ("AbsSuccess"=w251:bool, "AxisHandle OUT"=w249:u32)  [unwired: 8 in]
            }
          }
          frame #11 {
            n177 = while {
              tunnel: w253 -> [w262]
              tunnel: [w255] -> w252
              stop <- w256 stop-if-true
              n178 = local read "齿条推拉力(N)"() -> (w254:dbl)
              n179 = Wait Until Next ms Multiple(millisecond multiple=u32 50 ("毫秒倍数")) -> ()  [unwired: 1 out]
              n180 = call <userlib>:"Acm_AxGetCmdVelocity.vi"("AxisHandle"=w262) -> ("Velocity"=w261:dbl, "AxisHandle"=w255:u32)  [unwired: 1 in, 2 out]
              n181 = Equal To 0?(x=w261) -> (x = 0?=w258:bool)
              n182 = Greater Or Equal?(x=w254, y=500.0) -> (x >= y?=w257:bool)
              n183 = Or(x=w258, y=w257) -> (x .or. y?=w256:bool)
            }
          }
          frame #12 {
            n184 = call "PCI1220U停止.vi"("AxisHandle IN"=w263) -> ()  [unwired: 9 in, 2 out]
            n185 = local write "电动缸速度(mm/s)"(1.0 ("齿条移动速度")) -> ()
          }
          frame #13 {
            n186 = Wait (ms)(milliseconds to wait=u32 100 ("等待时间（毫秒）")) -> ()  [unwired: 1 out]
          }
          frame #14 {
            n187 = while {
              tunnel: [w271] -> w266
              stop <- w273 stop-if-true
              n188 = local read "齿条右极限"() -> (w269:dbl)
              n189 = Wait Until Next ms Multiple(millisecond multiple=u32 50 ("毫秒倍数")) -> ()  [unwired: 1 out]
              n190 = local read "电动缸电机"() -> (w270:u32)
              n191 = Subtract(x=w269, y=30.0) -> (x-y=w267:dbl)
              n192 = call "PCI1240电动缸位置模式 .vi"("Distance"=w267, "AxisHandle IN"=w270) -> ("AbsSuccess"=w273:bool, "AxisHandle OUT"=w271:u32)  [unwired: 8 in]
            }
          }
          frame #15 {
            n193 = while {
              tunnel: w275 -> [w284]
              tunnel: [w277] -> w274
              stop <- w278 stop-if-true
              n194 = local read "齿条推拉力(N)"() -> (w276:dbl)
              n195 = Wait Until Next ms Multiple(millisecond multiple=u32 50 ("毫秒倍数")) -> ()  [unwired: 1 out]
              n196 = call <userlib>:"Acm_AxGetCmdVelocity.vi"("AxisHandle"=w284) -> ("Velocity"=w283:dbl, "AxisHandle"=w277:u32)  [unwired: 1 in, 2 out]
              n197 = Equal To 0?(x=w283) -> (x = 0?=w280:bool)
              n198 = Greater Or Equal?(x=w276, y=500.0) -> (x >= y?=w279:bool)
              n199 = Or(x=w280, y=w279) -> (x .or. y?=w278:bool)
            }
          }
          frame #16 {
            n200 = call "PCI1220U停止.vi"("AxisHandle IN"=w287) -> ()  [unwired: 9 in, 2 out]
            n201 = local read "电动缸位置(mm)"() -> (w286:dbl)
            "齿条跑和右极限" <- w286
            n202 = local write "电动缸速度(mm/s)"(30.0 ("齿条移动速度")) -> ()
          }
          frame #17 {
            n203 = local read "齿条跑和左极限"() -> (w288:dbl)
            n204 = Add(x=w288, y=w292) -> (x+y=w291:dbl)
            n205 = Divide(x=w291, y=2.0) -> (x/y=w289:dbl)
            n206 = local write "转向器中心"(w289) -> ()
          }
          frame #18 {
            n207 = Wait (ms)(milliseconds to wait=u32 150 ("等待时间（毫秒）")) -> ()  [unwired: 1 out]
          }
          frame #19 {
            n208 = local read "转向器中心"() -> (w294:dbl)
            n209 = Wait Until Next ms Multiple(millisecond multiple=u32 50 ("毫秒倍数")) -> ()  [unwired: 1 out]
            n210 = call "PCI1240电动缸位置模式 .vi"("Distance"=w294) -> ("AxisHandle OUT"=w296:u32)  [unwired: 9 in, 1 out]
          }
          frame #20 {
            n211 = while {
              tunnel: w298 -> [w308]
              tunnel: [w299] -> w297
              stop <- w300 stop-if-true
              n212 = local read "齿条推拉力(N)"() -> (w305:dbl)
              n213 = Wait Until Next ms Multiple(millisecond multiple=u32 50 ("毫秒倍数")) -> ()  [unwired: 1 out]
              n214 = Absolute Value(x=w305) -> (abs(x)=w304:dbl)
              n215 = call <userlib>:"Acm_AxGetCmdVelocity.vi"("AxisHandle"=w308) -> ("Velocity"=w307:dbl, "AxisHandle"=w299:u32)  [unwired: 1 in, 2 out]
              n216 = Greater Or Equal?(x=w304, y=500.0) -> (x >= y?=w301:bool)
              n217 = Equal To 0?(x=w307) -> (x = 0?=w302:bool)
              n218 = Or(x=w302, y=w301) -> (x .or. y?=w300:bool)
            }
          }
          frame #21 {
            n219 = call "PCI1220U停止.vi"("AxisHandle IN"=w309) -> ()  [unwired: 9 in, 2 out]
          }
          frame #22 {
            n220 = local write "工步号"(u32 20 ("工步号")) -> ()
          }
        }
      }
      frame 20 {
        n221 = flat-sequence {
          tunnel: [w339] -> w320
          tunnel: w320 -> [w345]
          tunnel: [w352] -> w316
          tunnel: w316 -> [w359]
          tunnel: [w359] -> w315
          tunnel: w315 -> [w367]
          tunnel: [w367] -> w314
          tunnel: w314 -> [w368]
          tunnel: [w374] -> w318
          tunnel: [w376] -> w319
          tunnel: w318 -> [w376]
          tunnel: [w378] -> w325
          tunnel: w319 -> [w378]
          tunnel: w325 -> [w385]
          tunnel: [w384] -> w324
          tunnel: [w389] -> w323
          tunnel: [w388] -> w322
          tunnel: w324 -> [w387]
          tunnel: [w387] -> w321
          tunnel: [w416] -> w328
          tunnel: [w413] -> w327
          tunnel: w323 -> [w413]
          tunnel: [w412] -> w326
          tunnel: w322 -> [w412]
          tunnel: w321 -> [w416]
          tunnel: w328 -> [w420]
          tunnel: [w419] -> w317
          tunnel: w327 -> [w417]
          tunnel: w326 -> [w418]
          tunnel: w317 -> [w426]
          tunnel: [w425] -> w312
          tunnel: w312 -> [w433]
          tunnel: [w433] -> w311
          tunnel: w311 -> [w435]
          tunnel: [w434] -> w313
          tunnel: w313 -> [w445]
          frame #0 {
            n222 = local write "选项卡控件"(T1."间隙测量" ("选项卡控件")) -> ()
          }
          frame #1 {
            n223 = while {
              stop <- w330 stop-if-true
              n224 = local read "夹头松开"() -> (w332:bool)
              n225 = local read "夹头夹紧位"() -> (w331:bool)
              n226 = Wait Until Next ms Multiple(millisecond multiple=u32 50 ("毫秒倍数")) -> ()  [unwired: 1 out]
              n227 = Not(x=w332) -> (.not. x?=w333:bool)
              n228 = And(x=w331, y=w333) -> (x .and. y?=w330:bool)
            }
          }
          frame #2 {
            n229 = local read "转向器中心"() -> (w335:dbl)
            n230 = local read "电动缸电机"() -> (w338:u32)
            n231 = Add(x=w335, y=0.0) -> (x+y=w337:dbl)
            n232 = while {
              tunnel: w338 -> [w344]
              tunnel: w337 -> [w343]
              tunnel: [w340] -> w339
              stop <- w342 stop-if-true
              n233 = call "PCI1240电动缸位置模式 .vi"("Distance"=w343, "AxisHandle IN"=w344) -> ("AbsSuccess"=w342:bool, "AxisHandle OUT"=w340:u32)  [unwired: 8 in]
              n234 = Wait Until Next ms Multiple(millisecond multiple=u32 50 ("毫秒倍数")) -> ()  [unwired: 1 out]
            }
          }
          frame #3 {
            n235 = while {
              tunnel: w345 -> [w349]
              stop <- w347 stop-if-true
              n236 = call <userlib>:"Acm_AxGetCmdVelocity.vi"("AxisHandle"=w349) -> ("Velocity"=w348:dbl)  [unwired: 1 in, 3 out]
              n237 = Wait Until Next ms Multiple(millisecond multiple=u32 50 ("毫秒倍数")) -> ()  [unwired: 1 out]
              n238 = Equal To 0?(x=w348) -> (x = 0?=w347:bool)
            }
          }
          frame #4 {
            n239 = local write "测头机构轴速度(mm/s)"(30.0 ("测头机构轴速度(mm/s)")) -> ()
          }
          frame #5 {
            n240 = local read "测头机构电机"() -> (w353:u32)
            n241 = local read "测头机构轴检测位"() -> (w351:dbl)
            n242 = while {
              tunnel: w353 -> [w356]
              tunnel: w351 -> [w355]
              tunnel: [w354] -> w352
              stop <- w358 stop-if-true
              n243 = Wait Until Next ms Multiple(millisecond multiple=u32 50 ("毫秒倍数")) -> ()  [unwired: 1 out]
              n244 = call "PCI1220U进给轴位置模式.vi"("Distance"=w355, "AxisHandle IN"=w356) -> ("AbsSuccess"=w358:bool, "AxisHandle OUT"=w354:u32)  [unwired: 8 in]
            }
          }
          frame #6 {
            n245 = while {
              stop <- w362 stop-if-true
              n246 = local read "测头机构轴检测位"() -> (w364:dbl)
              n247 = local read "测头机构轴位置(mm)"() -> (w361:dbl)
              n248 = Wait Until Next ms Multiple(millisecond multiple=u32 50 ("毫秒倍数")) -> ()  [unwired: 1 out]
              n249 = Subtract(x=w364, y=20.0) -> (x-y=w360:dbl)
              n250 = Greater Or Equal?(x=w361, y=w360) -> (x >= y?=w362:bool)
            }
          }
          frame #7 {
            n251 = local write "测头机构轴速度(mm/s)"(10.0 ("测头机构轴速度(mm/s)")) -> ()
          }
          frame #8 {
            n252 = while {
              tunnel: w368 -> [w372]
              stop <- w370 stop-if-true
              n253 = call <userlib>:"Acm_AxGetCmdVelocity.vi"("AxisHandle"=w372) -> ("Velocity"=w371:dbl)  [unwired: 1 in, 3 out]
              n254 = Wait Until Next ms Multiple(millisecond multiple=u32 50 ("毫秒倍数")) -> ()  [unwired: 1 out]
              n255 = Equal To 0?(x=w371) -> (x = 0?=w370:bool)
            }
          }
          frame #9 {
            n256 = local write "旋转齿条轴使能"(TRUE ("旋转齿条轴使能")) -> ()
          }
          frame #10 {
            n257 = local read "旋转齿条电机"() -> (w374:u32)
            n258 = call "PCI1220U角度置零.vi"("AxisHandle IN"=w374) -> ()  [unwired: 10 in, 1 out]
          }
          frame #11 {
            n259 = local write "旋转齿条轴速度(°/s)"(1.0 ("旋转齿条轴速度(°/s)")) -> ()
            n260 = Wait Until Next ms Multiple(millisecond multiple=u32 2000 ("毫秒倍数")) -> ()  [unwired: 1 out]
          }
          frame #12 {
            n261 = while {
              i -> [w381]
              stop <- w379 stop-if-true
              n262 = local read "间隙位移(mm)"() -> (→"基准位移":dbl)
              n263 = Wait Until Next ms Multiple(millisecond multiple=u32 500 ("毫秒倍数")) -> ()  [unwired: 1 out]
              n264 = Greater Or Equal?(x=w381, y=4) -> (x >= y?=w379:bool)
            }
          }
          frame #13 {
            n265 = call "PCI1220U运行.vi"("方向"=enum32{"Negative", "Positive"}."Negative" ("Direction"), "AxisHandle IN"=w385) -> ("AxisHandle OUT"=w384:u32)  [unwired: 9 in]
          }
          frame #14 {
            w390 = dbl[] []
            n266 = while {
              shift-right: [w401] -> w389
              shift-left: w390 -> [w403]
              shift-right: [w400] -> w388
              shift-left: w390 -> [w402]
              stop <- w393 stop-if-true
              n267 = Wait (ms)(milliseconds to wait=u32 10 ("毫秒倍数")) -> ()  [unwired: 1 out]
              n268 = local read "间隙位移(mm)"() -> (w396:dbl)
              n269 = local read "基准位移"() -> (w394:dbl)
              n270 = local read "齿条扭矩(Nm)"() -> (w397:dbl)
              n271 = Subtract(x=w396, y=w394) -> (x-y=w395:dbl)
              n272 = Absolute Value(x=w397) -> (abs(x)=w392:dbl)
              n273 = Build Array (concatenate) ("创建数组")(w402, w395) -> (w400:dbl[])
              n274 = Build Array (concatenate) ("创建数组")(w403, w392) -> (w401:dbl[])
              n275 = Greater Or Equal?(x=w392, y="扭矩停止值") -> (x >= y?=w393:bool)
              n276 = Bundle ("捆绑")(w401, w400) -> (w398:cluster{dbl[], dbl[]})  [unwired: 1 in]
              n277 = Build Array ("创建数组")(w398) -> (w399:cluster{dbl[], dbl[]}[])
              n278 = local write "扭动曲线"(w399) -> ()
            }
          }
          frame #15 {
            n279 = Absolute Value(x=w413) -> (abs(x)=w414:dbl[])
            n280 = local read "测量点扭矩"() -> (w415:dbl)
            n281 = local read "基准位移"() -> (w409:dbl)
            n282 = call "自定义插值.vi"("压力"=w415, "扭矩数组"=w414, "位移数组"=w412) -> ("扭矩值"=w410:dbl)  [unwired: 8 in]
            n283 = Array Max & Min(array=w412) -> (min value=w411:dbl)  [unwired: 3 out]
            n284 = Absolute Value(x=w411) -> (abs(x)=w408:dbl)
            n285 = Subtract(x=w409, y=w408) -> (x-y=w407:dbl)
            n286 = Add(x=w408, y=w410) -> (x+y=w405:dbl)
            n287 = Absolute Value(x=w405) -> (abs(x)=w406:dbl)
            n288 = local write "中间位置间隙"(w406) -> ()
            n289 = local write "基准位移"(w407) -> ()
          }
          frame #16 {
            n290 = while {
              tunnel: w420 -> [w424]
              tunnel: [w423] -> w419
              stop <- w422 stop-if-true
              n291 = call "PCI1220U停止.vi"("AxisHandle IN"=w424) -> ("完成"=w422:bool, "AxisHandle OUT"=w423:u32)  [unwired: 9 in]
              n292 = Wait (ms)(milliseconds to wait=u32 50 ("毫秒倍数")) -> ()  [unwired: 1 out]
            }
            "间隙Y数组" <- w418
            "间隙X数组" <- w417
          }
          frame #17 {
            n293 = while {
              tunnel: [w431] -> w425
              tunnel: w426 -> [w429]
              stop <- w430 stop-if-true
              n294 = Wait Until Next ms Multiple(millisecond multiple=u32 50 ("毫秒倍数")) -> ()  [unwired: 1 out]
              n295 = call "PCI1220U扭矩轴位置模式.vi"("Distance"=0.0, "AxisHandle IN"=w429) -> ("AbsSuccess"=w430:bool, "AxisHandle OUT"=w431:u32)  [unwired: 8 in]
            }
          }
          frame #18 {
            n296 = Wait (ms)(milliseconds to wait=u32 500 ("等待时间（毫秒）")) -> ()  [unwired: 1 out]
          }
          frame #19 {
            n297 = while {
              tunnel: w435 -> [w443]
              tunnel: [w439] -> w434
              stop <- w440 stop-if-true
              n298 = local read "齿条扭矩(Nm)"() -> (w438:dbl)
              n299 = call <userlib>:"Acm_AxGetCmdVelocity.vi"("AxisHandle"=w443) -> ("Velocity"=w444:dbl, "AxisHandle"=w439:u32)  [unwired: 1 in, 2 out]
              n300 = Greater Or Equal?(x=w438, y=3.0) -> (x >= y?=w436:bool)
              n301 = Equal To 0?(x=w444) -> (x = 0?=w441:bool)
              n302 = Or(x=w441, y=w436) -> (x .or. y?=w440:bool)
              n303 = Wait Until Next ms Multiple(millisecond multiple=u32 50 ("毫秒倍数")) -> ()  [unwired: 1 out]
            }
          }
          frame #20 {
            n304 = while {
              tunnel: w445 -> [w449]
              tunnel: [w448] -> _
              stop <- w447 stop-if-true
              n305 = call "PCI1220U停止.vi"("AxisHandle IN"=w449) -> ("完成"=w447:bool, "AxisHandle OUT"=w448:u32)  [unwired: 9 in]
              n306 = Wait (ms)(milliseconds to wait=u32 50 ("毫秒倍数")) -> ()  [unwired: 1 out]
            }
          }
          frame #21 {
            n307 = local write "旋转齿条轴使能"(FALSE ("旋转齿条轴使能")) -> ()
            n308 = Wait (ms)(milliseconds to wait=u32 500 ("毫秒倍数")) -> ()  [unwired: 1 out]
          }
          frame #22 {
            n309 = local write "工步号"(u32 25 ("工步号")) -> ()
          }
        }
      }
      frame 25 {
        n310 = flat-sequence {
          frame #0 {
            n311 = local read "中间位置最大间隙标准(mm)"() -> (w454:dbl)
            n312 = local read "中间位置间隙"() -> (w455:dbl)
            n313 = local read "最小间隙(mm)"() -> (w453:dbl)
            n314 = In Range and Coerce(upper limit=w454, x=w455, lower limit=w453) -> (In Range?=w458:bool)  [unwired: 1 out]
            n315 = case shown="假" w458 {
              tunnel: [FALSE ("本序合格") TRUE ("本序合格")] -> w457
              tunnel: [w463 0.0 ("需调整角度(度)")] -> w456
              tunnel: w455 -> [w461 _]
              tunnel: w454 -> [w460 _]
              tunnel: w453 -> [w459 _]
              frame False {
                n316 = xnode "公式"("X"=w461, "Xmax"=w460, "Xmin"=w459) -> ("结果"=w463:dbl)  [unwired: 1 in, 1 out]
              }
              frame True {
              }
            }
            n317 = local write "单点间隙合格"(w457) -> ()
            n318 = local write "需调整角度(度)"(w456) -> ()
          }
          frame #1 {
            n319 = local read "单点间隙合格"() -> (w478:bool)
            n320 = case shown="假" w478 {
              frame False {
                n321 = local read "单点间隙已调试次数"() -> (w481:dbl)
                n322 = Less?(x=w481, y="间隙设定调整次数") -> (x < y?=w480:bool)
                n323 = case shown="假" w480 {
                  frame False {
                    n324 = local write "工步号"(u32 45 ("变更工步号")) -> ()
                  }
                  frame True {
                    n325 = local write "工步号"(u32 30 ("变更工步号")) -> ()
                  }
                }
              }
              frame True {
                n326 = local write "工步号"(u32 40 ("变更工步号")) -> ()
              }
            }
          }
        }
      }
      frame 30 {
        # "人工调整"
        n327 = flat-sequence {
          tunnel: [w487] -> w485
          tunnel: w485 -> [w494]
          frame #0 {
            n328 = local write "测头机构轴速度(mm/s)"(30.0 ("测头机构轴速度(mm/s)")) -> ()
          }
          frame #1 {
            n329 = local read "测头机构电机"() -> (w488:u32)
            n330 = while {
              tunnel: w488 -> [w491]
              tunnel: [w490] -> w487
              stop <- w493 stop-if-true
              n331 = local read "测头机构轴待检位"() -> (w489:dbl)
              n332 = call "PCI1220U进给轴位置模式.vi"("Distance"=w489, "AxisHandle IN"=w491) -> ("AbsSuccess"=w493:bool, "AxisHandle OUT"=w490:u32)  [unwired: 8 in]
              n333 = Wait Until Next ms Multiple(millisecond multiple=u32 50 ("毫秒倍数")) -> ()  [unwired: 1 out]
            }
          }
          frame #2 {
            n334 = while {
              tunnel: w494 -> [w498]
              stop <- w496 stop-if-true
              n335 = call <userlib>:"Acm_AxGetCmdVelocity.vi"("AxisHandle"=w498) -> ("Velocity"=w497:dbl)  [unwired: 1 in, 3 out]
              n336 = Wait Until Next ms Multiple(millisecond multiple=u32 50 ("毫秒倍数")) -> ()  [unwired: 1 out]
              n337 = Equal To 0?(x=w497) -> (x = 0?=w496:bool)
            }
          }
          frame #3 {
            n338 = while {
              stop <- w500 stop-if-true
              n339 = local read "测头机构轴位置(mm)"() -> (w502:dbl)
              n340 = Wait Until Next ms Multiple(millisecond multiple=u32 50 ("毫秒倍数")) -> ()  [unwired: 1 out]
              n341 = Less Or Equal?(x=w502, y=35.0) -> (x <= y?=w500:bool)
            }
          }
          frame #4 {
            n342 = local write "测头气缸左移"(TRUE ("测头气缸左移")) -> ()
            n343 = local write "测头气缸右移"(FALSE ("测头气缸右移")) -> ()
          }
          frame #5 {
            n344 = while {
              stop <- w505 stop-if-true
              # "等待启动"
              n345 = local read "间隙启动"() -> (w505:bool)
              n346 = Wait Until Next ms Multiple(millisecond multiple=u32 50 ("毫秒倍数")) -> ()  [unwired: 1 out]
            }
          }
          frame #6 {
            n347 = local read "不合格品"() -> (w507:bool)
            n348 = case shown="假" w507 {
              frame False {
                n349 = flat-sequence {
                  frame #0 {
                    n350 = local read "单点间隙已调试次数"() -> (w510:dbl)
                    n351 = local write "测头气缸左移"(FALSE ("测头气缸左移")) -> ()
                    n352 = local write "测头气缸右移"(TRUE ("测头气缸左移")) -> ()
                    n353 = Add(x=w510, y=1.0 ("已调试次数")) -> (x+y=w512:dbl)
                    n354 = local write "单点间隙已调试次数"(w512) -> ()
                  }
                  frame #1 {
                    n355 = while {
                      stop <- w513 stop-if-true
                      n356 = Wait Until Next ms Multiple(millisecond multiple=u32 50 ("毫秒倍数")) -> ()  [unwired: 1 out]
                      n357 = local read "测头右位"() -> (w513:bool)
                    }
                  }
                  frame #2 {
                    n358 = local write "工步号"(u32 20 ("工步号")) -> ()
                  }
                }
              }
              frame True {
                n359 = local write "工步号"(u32 45 ("工步号")) -> ()
              }
            }
          }
        }
      }
      frame 40 {
        n360 = flat-sequence {
          tunnel: [w633] -> w629
          tunnel: w629 -> [w635]
          tunnel: [w634] -> w628
          tunnel: w628 -> [w643]
          tunnel: [w643] -> w627
          tunnel: w627 -> [w655]
          tunnel: [w655] -> w626
          tunnel: w626 -> [w657]
          tunnel: [w656] -> w625
          tunnel: w625 -> [w665]
          tunnel: [w665] -> w624
          tunnel: w624 -> [w675]
          tunnel: [w675] -> w623
          tunnel: w623 -> [w683]
          tunnel: [w683] -> w622
          tunnel: w622 -> [w685]
          tunnel: [w686] -> w621
          tunnel: [w684] -> w620
          tunnel: w621 -> [w699]
          tunnel: w620 -> [w694]
          tunnel: [w697] -> w619
          tunnel: [w696] -> w618
          tunnel: [w695] -> w617
          tunnel: [w694] -> w616
          tunnel: [w730] -> w615
          tunnel: [w733] -> w614
          tunnel: w619 -> [w733]
          tunnel: [w732] -> w613
          tunnel: w618 -> [w732]
          tunnel: [w731] -> w612
          tunnel: w617 -> [w731]
          tunnel: w616 -> [w730]
          tunnel: w615 -> [w739]
          tunnel: [w735] -> w611
          tunnel: [w738] -> w610
          tunnel: w614 -> [w738]
          tunnel: [w737] -> w609
          tunnel: w613 -> [w737]
          tunnel: [w736] -> w608
          tunnel: w612 -> [w736]
          tunnel: [w734] -> w607
          tunnel: [w754] -> w603
          tunnel: [w753] -> w604
          tunnel: [w752] -> w605
          tunnel: w611 -> [w747]
          tunnel: w610 -> [w751]
          tunnel: w609 -> [w750]
          tunnel: w608 -> [w749]
          tunnel: w607 -> [w748]
          tunnel: [w747] -> w606
          tunnel: [w801] -> w602
          tunnel: [w786] -> w601
          tunnel: [w800] -> w600
          tunnel: [w799] -> w599
          tunnel: [w798] -> w598
          tunnel: [w797] -> w597
          tunnel: [w796] -> w596
          tunnel: w606 -> [w800]
          tunnel: w605 -> [w799]
          tunnel: w604 -> [w786]
          tunnel: w603 -> [w801]
          tunnel: [w787] -> w595
          tunnel: w602 -> [w823]
          tunnel: [w823] -> w594
          tunnel: w601 -> [w822]
          tunnel: [w822] -> w593
          tunnel: w600 -> [w821]
          tunnel: [w810] -> w592
          tunnel: [w809] -> w591
          tunnel: [w820] -> w590
          tunnel: w599 -> [w820]
          tunnel: w598 -> [w817]
          tunnel: w597 -> [w819]
          tunnel: w596 -> [w818]
          tunnel: [w812] -> w589
          tunnel: [w811] -> w588
          tunnel: w595 -> [w808]
          tunnel: w594 -> [w836]
          tunnel: w593 -> [w835]
          tunnel: w592 -> [w831]
          tunnel: w591 -> [w838]
          tunnel: [w838] -> w586
          tunnel: w590 -> [w837]
          tunnel: [w833] -> w585
          tunnel: w589 -> [w840]
          tunnel: [w840] -> w584
          tunnel: w588 -> [w839]
          tunnel: [w839] -> w583
          tunnel: [w834] -> w587
          tunnel: [w832] -> w582
          tunnel: [w831] -> w581
          tunnel: w587 -> [w879]
          tunnel: [w879] -> w580
          tunnel: [w873] -> w579
          tunnel: w586 -> [w878]
          tunnel: [w878] -> w578
          tunnel: w585 -> [w877]
          tunnel: [w877] -> w577
          tunnel: w584 -> [w876]
          tunnel: [w876] -> w576
          tunnel: w583 -> [w875]
          tunnel: [w875] -> w575
          tunnel: [w874] -> w574
          tunnel: w582 -> [w874]
          tunnel: w581 -> [w873]
          tunnel: w580 -> [w886]
          tunnel: [w886] -> w573
          tunnel: w579 -> [w880]
          tunnel: w578 -> [w885]
          tunnel: [w885] -> w572
          tunnel: w577 -> [w884]
          tunnel: [w884] -> w571
          tunnel: w576 -> [w883]
          tunnel: [w883] -> w570
          tunnel: w575 -> [w882]
          tunnel: [w882] -> w569
          tunnel: [w880] -> w568
          tunnel: [w881] -> w567
          tunnel: w574 -> [w881]
          tunnel: [w902] -> w566
          tunnel: [w901] -> w565
          tunnel: w573 -> [w894]
          tunnel: [w893] -> w564
          tunnel: w572 -> [w896]
          tunnel: [w896] -> w563
          tunnel: w571 -> [w897]
          tunnel: [w900] -> w562
          tunnel: w570 -> [w898]
          tunnel: w569 -> [w899]
          tunnel: [w899] -> w561
          tunnel: [w898] -> w560
          tunnel: w568 -> [w893]
          tunnel: w567 -> [w895]
          tunnel: w566 -> [w939]
          tunnel: w565 -> [w945]
          tunnel: [w945] -> w559
          tunnel: w564 -> [w942]
          tunnel: [w942] -> w558
          tunnel: w563 -> [w944]
          tunnel: [w944] -> w557
          tunnel: w562 -> [w943]
          tunnel: [w943] -> w556
          tunnel: [w939] -> w555
          tunnel: [w938] -> w554
          tunnel: [w937] -> w553
          tunnel: w561 -> [w935]
          tunnel: w560 -> [w936]
          tunnel: [w936] -> w552
          tunnel: [w935] -> w551
          tunnel: [w934] -> w550
          tunnel: w559 -> [w958]
          tunnel: [w992] -> w549
          tunnel: w558 -> [w992]
          tunnel: [w991] -> w548
          tunnel: w557 -> [w991]
          tunnel: w556 -> [w990]
          tunnel: [w988] -> w547
          tunnel: w555 -> [w987]
          tunnel: w554 -> [w985]
          tunnel: w553 -> [w984]
          tunnel: [w982] -> w546
          tunnel: [w981] -> w545
          tunnel: [w980] -> w544
          tunnel: [w955] -> w543
          tunnel: [w954] -> w542
          tunnel: w552 -> [w977]
          tunnel: w551 -> [w976]
          tunnel: [w977] -> w541
          tunnel: [w976] -> w540
          tunnel: [w975] -> w539
          tunnel: [w974] -> w538
          tunnel: [w971] -> w537
          tunnel: [w966] -> w536
          tunnel: [w961] -> w535
          tunnel: [w953] -> w534
          tunnel: w550 -> [w952]
          tunnel: w549 -> [w1019]
          tunnel: [w1019] -> w533
          tunnel: w548 -> [_]
          tunnel: [w1016] -> w532
          tunnel: w547 -> [w1018]
          tunnel: w546 -> [w1014]
          tunnel: w545 -> [w1013]
          tunnel: w544 -> [w1012]
          tunnel: [w1011] -> w531
          tunnel: [w1010] -> w530
          tunnel: w543 -> [w1009]
          tunnel: w542 -> [w1008]
          tunnel: w541 -> [w1004]
          tunnel: w540 -> [w1003]
          tunnel: [w1004] -> w529
          tunnel: [w1003] -> w528
          tunnel: [w1002] -> w527
          tunnel: [w1001] -> w526
          tunnel: w539 -> [w1001]
          tunnel: [w1000] -> w525
          tunnel: w538 -> [w1000]
          tunnel: [w999] -> w524
          tunnel: [w998] -> w523
          tunnel: w537 -> [w997]
          tunnel: [w996] -> w522
          tunnel: w536 -> [w996]
          tunnel: [w995] -> w521
          tunnel: w535 -> [w995]
          tunnel: w534 -> [w994]
          tunnel: w533 -> [w1035]
          tunnel: [w1035] -> w520
          tunnel: w532 -> [w1034]
          tunnel: [w1034] -> w519
          tunnel: w531 -> [w1029]
          tunnel: w530 -> [w1028]
          tunnel: w529 -> [w1031]
          tunnel: w528 -> [w1030]
          tunnel: w527 -> [w1027]
          tunnel: w526 -> [w1026]
          tunnel: w525 -> [w1025]
          tunnel: w524 -> [w1024]
          tunnel: w523 -> [w1023]
          tunnel: w522 -> [w1021]
          tunnel: w521 -> [w1020]
          tunnel: w520 -> [w1038]
          tunnel: [w1037] -> w518
          tunnel: w519 -> [w1036]
          tunnel: w518 -> [w1045]
          tunnel: [w1044] -> w517
          tunnel: w517 -> [w1051]
          frame #0 {
            n361 = local read "电动缸快速"() -> (w630:dbl)
            n362 = local write "电动缸速度(mm/s)"(w630) -> ()
            n363 = local write "单点间隙已调试次数"(0.0 ("单点间隙已调试次数")) -> ()
            n364 = local read "电动缸电机"() -> (w633:u32)
            n365 = local write "选项卡控件"(T1."轴向力测量" ("选项卡控件")) -> ()
          }
          frame #1 {
            n366 = while {
              tunnel: w635 -> [w642]
              tunnel: [w641] -> w634
              stop <- w636 stop-if-true
              n367 = local read "齿条左极限"() -> (w639:dbl)
              n368 = Wait (ms)(milliseconds to wait=u32 50 ("毫秒倍数")) -> ()  [unwired: 1 out]
              n369 = local read "循环退出"() -> (w638:bool)
              n370 = call "PCI1240电动缸位置模式 .vi"("Distance"=w639, "AxisHandle IN"=w642) -> ("AbsSuccess"=w637:bool, "AxisHandle OUT"=w641:u32)  [unwired: 8 in]
              n371 = Compound Arithmetic op=OR(w637, w638) -> (w636:bool)
            }
          }
          frame #2 {
            n372 = while {
              tunnel: w643 -> [w644]
              stop <- w646 stop-if-true
              n373 = local read "齿条推拉力(N)"() -> (w650:dbl)
              n374 = Wait (ms)(milliseconds to wait=u32 50 ("毫秒倍数")) -> ()  [unwired: 1 out]
              n375 = call <userlib>:"Acm_AxGetCmdVelocity.vi"("AxisHandle"=w644) -> ("Velocity"=w652:dbl)  [unwired: 1 in, 3 out]
              n376 = local read "循环退出"() -> (w645:bool)
              n377 = Less Or Equal?(x=w650, y=-500.0) -> (x <= y?=w647:bool)
              n378 = Equal To 0?(x=w652) -> (x = 0?=w648:bool)
              n379 = Compound Arithmetic op=OR(w648, w647, w645) -> (w646:bool)
            }
          }
          frame #3 {
            n380 = local read "电动缸慢速"() -> (w653:dbl)
            n381 = local write "电动缸速度(mm/s)"(w653) -> ()
            n382 = Wait (ms)(milliseconds to wait=u32 100 ("等待时间（毫秒）")) -> ()  [unwired: 1 out]
          }
          frame #4 {
            n383 = while {
              tunnel: w657 -> [w664]
              tunnel: [w662] -> w656
              stop <- w658 stop-if-true
              n384 = Wait (ms)(milliseconds to wait=u32 50 ("毫秒倍数")) -> ()  [unwired: 1 out]
              n385 = local read "循环退出"() -> (w660:bool)
              n386 = call "PCI1240电动缸位置模式 .vi"("Distance"=10000.0, "AxisHandle IN"=w664) -> ("AbsSuccess"=w659:bool, "AxisHandle OUT"=w662:u32)  [unwired: 8 in]
              n387 = Compound Arithmetic op=OR(w659, w660) -> (w658:bool)
            }
          }
          frame #5 {
            n388 = while {
              tunnel: w665 -> [w666]
              stop <- w668 stop-if-true
              n389 = local read "齿条推拉力(N)"() -> (w672:dbl)
              n390 = Wait (ms)(milliseconds to wait=u32 50 ("毫秒倍数")) -> ()  [unwired: 1 out]
              n391 = call <userlib>:"Acm_AxGetCmdVelocity.vi"("AxisHandle"=w666) -> ("Velocity"=w674:dbl)  [unwired: 1 in, 3 out]
              n392 = local read "循环退出"() -> (w667:bool)
              n393 = Less Or Equal?(x=w672, y=-500.0) -> (x <= y?=w669:bool)
              n394 = Equal To 0?(x=w674) -> (x = 0?=w670:bool)
              n395 = Compound Arithmetic op=OR(w670, w669, w667) -> (w668:bool)
            }
          }
          frame #6 {
            n396 = while {
              tunnel: w675 -> [w680]
              stop <- w676 stop-if-true
              n397 = call "PCI1220U停止.vi"("AxisHandle IN"=w680) -> ("完成"=w677:bool)  [unwired: 9 in, 1 out]
              n398 = local read "循环退出"() -> (w678:bool)
              n399 = Wait (ms)(milliseconds to wait=u32 50 ("毫秒倍数")) -> ()  [unwired: 1 out]
              n400 = Compound Arithmetic op=OR(w677, w678) -> (w676:bool)
            }
          }
          frame #7 {
            n401 = local read "电动缸快速"() -> (w681:dbl)
            n402 = local write "电动缸速度(mm/s)"(w681) -> ()
            n403 = Wait (ms)(milliseconds to wait=u32 100 ("毫秒倍数")) -> ()  [unwired: 1 out]
          }
          frame #8 {
            n404 = while {
              tunnel: w685 -> [w693]
              tunnel: [w691] -> w684
              stop <- w687 stop-if-true
              n405 = local read "齿条右极限"() -> (w690:dbl)
              n406 = Wait (ms)(milliseconds to wait=u32 50 ("毫秒倍数")) -> ()  [unwired: 1 out]
              n407 = local read "循环退出"() -> (w689:bool)
              n408 = call "PCI1240电动缸位置模式 .vi"("Distance"=w690, "AxisHandle IN"=w693) -> ("AbsSuccess"=w688:bool, "AxisHandle OUT"=w691:u32)  [unwired: 8 in]
              n409 = Compound Arithmetic op=OR(w688, w689) -> (w687:bool)
            }
            n410 = local read "转向器中心"() -> (w686:dbl)
          }
          frame #9 {
            w698 = dbl[] []
            n411 = while {
              shift-right: [w717] -> w696
              shift-left: w698 -> [w727]
              shift-right: [w725] -> w697
              shift-left: w698 -> [w726]
              tunnel: w694 -> [w721]
              tunnel: w699 -> [w720]
              shift-right: [w716] -> w695
              shift-left: w698 -> [w718]
              stop <- w710 stop-if-true
              n412 = local read "中间位置间隙"() -> (w707:dbl)
              n413 = local read "基准位移"() -> (w722:dbl)
              n414 = local read "间隙位移(mm)"() -> (w706:dbl)
              n415 = local read "电动缸位置(mm)"() -> (w702:dbl)
              n416 = call <userlib>:"Acm_AxGetCmdVelocity.vi"("AxisHandle"=w721) -> ("Velocity"=w715:dbl)  [unwired: 1 in, 3 out]
              n417 = Wait (ms)(milliseconds to wait=u32 50 ("毫秒倍数")) -> ()  [unwired: 1 out]
              n418 = local read "齿条推拉力(N)"() -> (w713:dbl)
              n419 = Subtract(x=w706, y=w722) -> (x-y=w709:dbl)
              n420 = Subtract(x=w709, y=w707) -> (x-y=w708:dbl)
              n421 = Subtract(x=w702, y=w720) -> (x-y=w705:dbl)
              n422 = Negate(x=w708) -> (-x=w700:dbl)
              n423 = local read "循环退出"() -> (w701:bool)
              n424 = Multiply(x=w705, y=1.0) -> (x*y=w703:dbl)
              n425 = Build Array (concatenate) ("创建数组")(w726, w700) -> (w725:dbl[])
              n426 = Build Array (concatenate) ("创建数组")(w727, w703) -> (w717:dbl[])
              n427 = Build Array (concatenate) ("创建数组")(w718, w713) -> (w716:dbl[])
              n428 = Greater Or Equal?(x=w713, y=500.0) -> (x >= y?=w711:bool)
              n429 = Equal To 0?(x=w715) -> (x = 0?=w712:bool)
              n430 = Bundle ("捆绑")(w717, w725) -> (w723:cluster{dbl[], dbl[]})  [unwired: 1 in]
              n431 = Compound Arithmetic op=OR(w712, w711, w701) -> (w710:bool)
              n432 = Bundle ("捆绑")(w717, w716) -> (w719:cluster{dbl[], dbl[]})  [unwired: 1 in]
              n433 = Build Array ("创建数组")(w723, w719) -> (w724:cluster{dbl[], dbl[]}[])
              n434 = local write "行程跳动曲线"(w724) -> ()
            }
          }
          frame #10 {
            n435 = local read "电动缸慢速"() -> (w729:dbl)
            n436 = local write "电动缸速度(mm/s)"(w729) -> ()
          }
          frame #11 {
            n437 = while {
              tunnel: w739 -> [w746]
              tunnel: [w744] -> w735
              stop <- w740 stop-if-true
              n438 = Wait (ms)(milliseconds to wait=u32 50 ("毫秒倍数")) -> ()  [unwired: 1 out]
              n439 = local read "循环退出"() -> (w742:bool)
              n440 = call "PCI1240电动缸位置模式 .vi"("Distance"=-10.0, "AxisHandle IN"=w746) -> ("AbsSuccess"=w741:bool, "AxisHandle OUT"=w744:u32)  [unwired: 8 in]
              n441 = Compound Arithmetic op=OR(w741, w742) -> (w740:bool)
            }
            n442 = local read "转向器中心"() -> (w734:dbl)
          }
          frame #12 {
            n443 = while {
              shift-right: [w772] -> w753
              shift-left: w750 -> [w782]
              shift-right: [w780] -> w754
              shift-left: w751 -> [w781]
              tunnel: w747 -> [w776]
              tunnel: w748 -> [w775]
              shift-right: [w771] -> w752
              shift-left: w749 -> [w773]
              stop <- w765 stop-if-true
              n444 = local read "中间位置间隙"() -> (w762:dbl)
              n445 = local read "基准位移"() -> (w777:dbl)
              n446 = local read "间隙位移(mm)"() -> (w761:dbl)
              n447 = local read "电动缸位置(mm)"() -> (w757:dbl)
              n448 = call <userlib>:"Acm_AxGetCmdVelocity.vi"("AxisHandle"=w776) -> ("Velocity"=w770:dbl)  [unwired: 1 in, 3 out]
              n449 = Wait (ms)(milliseconds to wait=u32 50 ("毫秒倍数")) -> ()  [unwired: 1 out]
              n450 = local read "齿条推拉力(N)"() -> (w768:dbl)
              n451 = Subtract(x=w761, y=w777) -> (x-y=w764:dbl)
              n452 = Subtract(x=w757, y=w775) -> (x-y=w760:dbl)
              n453 = Subtract(x=w764, y=w762) -> (x-y=w763:dbl)
              n454 = Negate(x=w763) -> (-x=w755:dbl)
              n455 = Multiply(x=w760, y=1.0) -> (x*y=w758:dbl)
              n456 = local read "循环退出"() -> (w756:bool)
              n457 = Build Array (concatenate) ("创建数组")(w781, w755) -> (w780:dbl[])
              n458 = Build Array (concatenate) ("创建数组")(w782, w758) -> (w772:dbl[])
              n459 = Build Array (concatenate) ("创建数组")(w773, w768) -> (w771:dbl[])
              n460 = Greater Or Equal?(x=w768, y=500.0) -> (x >= y?=w766:bool)
              n461 = Equal To 0?(x=w770) -> (x = 0?=w767:bool)
              n462 = Bundle ("捆绑")(w772, w780) -> (w778:cluster{dbl[], dbl[]})  [unwired: 1 in]
              n463 = Bundle ("捆绑")(w772, w771) -> (w774:cluster{dbl[], dbl[]})  [unwired: 1 in]
              n464 = Compound Arithmetic op=OR(w767, w766, w756) -> (w765:bool)
              n465 = Build Array ("创建数组")(w778, w774) -> (w779:cluster{dbl[], dbl[]}[])
              n466 = local write "行程跳动曲线"(w779) -> ()
            }
          }
          frame #13 {
            n467 = while {
              tunnel: w800 -> [w807]
              tunnel: [w806] -> _
              stop <- w802 stop-if-true
              n468 = call "PCI1220U停止.vi"("AxisHandle IN"=w807) -> ("完成"=w803:bool, "AxisHandle OUT"=w806:u32)  [unwired: 9 in]
              n469 = Wait (ms)(milliseconds to wait=u32 50 ("毫秒倍数")) -> ()  [unwired: 1 out]
              n470 = local read "循环退出"() -> (w804:bool)
              n471 = Compound Arithmetic op=OR(w803, w804) -> (w802:bool)
            }
            n472 = call "功能计算_何 截取位移左.vi"("位移数组"=w786, "拉压力数组"=w799, "半行程"="半行程", "截取百分比"="截取百分比") -> ("峰值扭矩"=w798:dbl, "平均扭矩"=w797:dbl, "扭差"=w796:dbl)  [unwired: 12 in, 1 out]
            "左轴向力波动(N)" <- w796
            "左最大轴向力(N)" <- w798
            n473 = call "间隙计算.vi"("扭矩数组"=w801) -> ("峰值间隙1"=w795:dbl, "峰值间隙2"=w794:dbl)  [unwired: 6 in, 3 out]
            n474 = local read "180°内全行程间隙标准(mm)"() -> (w793:dbl)
            n475 = Array Size(array=w786) -> (size(s)=w785:i32)
            n476 = local read "180°外全行程间隙标准(mm)"() -> (w790:dbl)
            n477 = local write "左平均轴向力(N)"(w797) -> ()
            n478 = local write "左180°外全行程间隙"(w794) -> ()
            n479 = local write "左180°内全行程间隙"(w795) -> ()
            n480 = local write "左轴向力数组大小"(w785) -> ()
            n481 = local read "电动缸快速"() -> (w784:dbl)
            n482 = Greater?(x=w795, y=w793) -> (0:w792:bool)
            n483 = Greater?(x=w794, y=w790) -> (0:w791:bool)
            n484 = local write "电动缸速度(mm/s)"(w784) -> ()
            n485 = property on="左180°内全行程间隙" class="DigNum (严格)"("Blinking"=w792) -> ()  [unwired: 2 in, 2 out]
            n486 = property on="左180°外全行程间隙" class="DigNum (严格)"("Blinking"=w791) -> ()  [unwired: 2 in, 2 out]
            n487 = local read "最大轴向力标准(N)"() -> (w787:dbl)
          }
          frame #14 {
            n488 = while {
              tunnel: w821 -> [w830]
              tunnel: [w827] -> w810
              stop <- w824 stop-if-true
              n489 = Wait (ms)(milliseconds to wait=u32 50 ("毫秒倍数")) -> ()  [unwired: 1 out]
              n490 = local read "齿条左极限"() -> (w828:dbl)
              n491 = local read "循环退出"() -> (w826:bool)
              n492 = call "PCI1240电动缸位置模式 .vi"("Distance"=w828, "AxisHandle IN"=w830) -> ("AbsSuccess"=w825:bool, "AxisHandle OUT"=w827:u32)  [unwired: 8 in]
              n493 = Compound Arithmetic op=OR(w825, w826) -> (w824:bool)
            }
            n494 = local read "轴向力标准(N)"() -> (w815:dbl)
            n495 = local read "平均轴向力标准(N) max"() -> (w814:dbl)
            n496 = local read "力波动标准(N)"() -> (w813:dbl)
            n497 = call "判断.vi"("y 3"=w813, "y 2-2"=w814, "y 2-1"=w815, "y"=w808, "x 3"=w818, "x 2"=w819, "x"=w817) -> ("非x? 3"=w811:bool, "非x? 2"=w816:bool, "非x?"=w812:bool)  [unwired: 2 in]
            n498 = property on="左最大轴向力(N)" class="DigNum (严格)"("Blinking"=w812) -> ()  [unwired: 2 in, 2 out]
            n499 = property on="左平均轴向力(N)" class="DigNum (严格)"("Blinking"=w816) -> ()  [unwired: 2 in, 2 out]
            n500 = property on="左轴向力波动(N)" class="DigNum (严格)"("Blinking"=w811) -> ()  [unwired: 2 in, 2 out]
            n501 = local read "转向器中心"() -> (w809:dbl)
          }
          frame #15 {
            n502 = while {
              shift-right: [w861] -> w832
              shift-left: w835 -> [w870]
              shift-right: [w868] -> w834
              shift-left: w836 -> [w869]
              tunnel: w831 -> [w863]
              tunnel: w838 -> [w862]
              shift-right: [w858] -> w833
              shift-left: w837 -> [w859]
              stop <- w853 stop-if-true
              n503 = local read "电动缸位置(mm)"() -> (w843:dbl)
              n504 = call <userlib>:"Acm_AxGetCmdVelocity.vi"("AxisHandle"=w863) -> ("Velocity"=w851:dbl)  [unwired: 1 in, 3 out]
              n505 = local read "间隙位移(mm)"() -> (w849:dbl)
              n506 = local read "基准位移"() -> (w864:dbl)
              n507 = Wait (ms)(milliseconds to wait=u32 50 ("毫秒倍数")) -> ()  [unwired: 1 out]
              n508 = local read "中间位置间隙"() -> (w850:dbl)
              n509 = local read "齿条推拉力(N)"() -> (w857:dbl)
              n510 = Add(x=1.47, y=w843) -> (x+y=w845:dbl)
              n511 = Subtract(x=w849, y=w864) -> (x-y=w865:dbl)
              n512 = Subtract(x=w845, y=w862) -> (x-y=w848:dbl)
              n513 = local read "循环退出"() -> (w842:bool)
              n514 = Subtract(x=w865, y=w850) -> (x-y=w852:dbl)
              n515 = Negate(x=w852) -> (-x=w841:dbl)
              n516 = Multiply(x=w848, y=1.0) -> (x*y=w846:dbl)
              n517 = Build Array (concatenate) ("创建数组")(w870, w846) -> (w861:dbl[])
              n518 = Less Or Equal?(x=w857, y=-500.0) -> (x <= y?=w854:bool)
              n519 = Build Array (concatenate) ("创建数组")(w859, w857) -> (w858:dbl[])
              n520 = Equal To 0?(x=w851) -> (x = 0?=w855:bool)
              n521 = Build Array (concatenate) ("创建数组")(w869, w841) -> (w868:dbl[])
              n522 = Bundle ("捆绑")(w861, w858) -> (w860:cluster{dbl[], dbl[]})  [unwired: 1 in]
              n523 = Compound Arithmetic op=OR(w855, w854, w842) -> (w853:bool)
              n524 = Bundle ("捆绑")(w861, w868) -> (w866:cluster{dbl[], dbl[]})  [unwired: 1 in]
              n525 = Build Array ("创建数组")(w866, w860) -> (w867:cluster{dbl[], dbl[]}[])
              n526 = local write "行程跳动曲线"(w867) -> ()
            }
          }
          frame #16 {
            n527 = local read "电动缸慢速"() -> (w872:dbl)
            n528 = local write "电动缸速度(mm/s)"(w872) -> ()
          }
          frame #17 {
            n529 = while {
              tunnel: w880 -> [w892]
              stop <- w887 stop-if-true
              n530 = Wait (ms)(milliseconds to wait=u32 50 ("毫秒倍数")) -> ()  [unwired: 1 out]
              n531 = local read "循环退出"() -> (w889:bool)
              n532 = call "PCI1240电动缸位置模式 .vi"("Distance"=160.0, "AxisHandle IN"=w892) -> ("AbsSuccess"=w888:bool)  [unwired: 8 in, 1 out]
              n533 = Compound Arithmetic op=OR(w888, w889) -> (w887:bool)
            }
          }
          frame #18 {
            n534 = while {
              shift-right: [w923] -> w901
              shift-left: w895 -> [w932]
              shift-right: [w930] -> w902
              shift-left: w894 -> [w931]
              tunnel: w893 -> [w925]
              tunnel: w896 -> [w924]
              shift-right: [w920] -> w900
              shift-left: w897 -> [w921]
              stop <- w915 stop-if-true
              n535 = local read "电动缸位置(mm)"() -> (w905:dbl)
              n536 = call <userlib>:"Acm_AxGetCmdVelocity.vi"("AxisHandle"=w925) -> ("Velocity"=w913:dbl)  [unwired: 1 in, 3 out]
              n537 = local read "间隙位移(mm)"() -> (w911:dbl)
              n538 = local read "基准位移"() -> (w926:dbl)
              n539 = Wait (ms)(milliseconds to wait=u32 50 ("毫秒倍数")) -> ()  [unwired: 1 out]
              n540 = local read "中间位置间隙"() -> (w912:dbl)
              n541 = local read "齿条推拉力(N)"() -> (w919:dbl)
              n542 = Subtract(x=w911, y=w926) -> (x-y=w927:dbl)
              n543 = Add(x=1.45, y=w905) -> (x+y=w907:dbl)
              n544 = Subtract(x=w907, y=w924) -> (x-y=w910:dbl)
              n545 = Subtract(x=w927, y=w912) -> (x-y=w914:dbl)
              n546 = local read "循环退出"() -> (w904:bool)
              n547 = Negate(x=w914) -> (-x=w903:dbl)
              n548 = Multiply(x=w910, y=1.0) -> (x*y=w908:dbl)
              n549 = Build Array (concatenate) ("创建数组")(w932, w908) -> (w923:dbl[])
              n550 = Less Or Equal?(x=w919, y=-500.0) -> (x <= y?=w916:bool)
              n551 = Build Array (concatenate) ("创建数组")(w921, w919) -> (w920:dbl[])
              n552 = Equal To 0?(x=w913) -> (x = 0?=w917:bool)
              n553 = Build Array (concatenate) ("创建数组")(w931, w903) -> (w930:dbl[])
              n554 = Bundle ("捆绑")(w923, w920) -> (w922:cluster{dbl[], dbl[]})  [unwired: 1 in]
              n555 = Compound Arithmetic op=OR(w917, w916, w904) -> (w915:bool)
              n556 = Bundle ("捆绑")(w923, w930) -> (w928:cluster{dbl[], dbl[]})  [unwired: 1 in]
              n557 = Build Array ("创建数组")(w928, w922) -> (w929:cluster{dbl[], dbl[]}[])
              n558 = local write "行程跳动曲线"(w929) -> ()
            }
          }
          frame #19 {
            n559 = while {
              tunnel: w942 -> [w951]
              tunnel: [w950] -> _
              stop <- w946 stop-if-true
              n560 = local read "循环退出"() -> (w948:bool)
              n561 = call "PCI1220U停止.vi"("AxisHandle IN"=w951) -> ("完成"=w947:bool, "AxisHandle OUT"=w950:u32)  [unwired: 9 in]
              n562 = Wait (ms)(milliseconds to wait=u32 50 ("毫秒倍数")) -> ()  [unwired: 1 out]
              n563 = Compound Arithmetic op=OR(w947, w948) -> (w946:bool)
            }
            n564 = Array Max & Min(array=w939) -> (max value=w941:dbl, min value=w940:dbl)  [unwired: 2 out]
            n565 = local read "左轴向力数组大小"() -> (w934:i32)
            n566 = Absolute Value(x=w941) -> (abs(x)=w938:dbl)
            n567 = Absolute Value(x=w940) -> (abs(x)=w937:dbl)
            n568 = local write "左全行程间隙"(w938) -> ()
            n569 = local write "右全行程间隙"(w937) -> ()
          }
          frame #20 {
            n570 = local read "180°内全行程间隙标准(mm)"() -> (w983:dbl)
            n571 = local read "截取百分比"() -> (w956:dbl)
            n572 = local read "齿条传动比"() -> (w960:dbl)
            n573 = local read "半行程"() -> (w957:dbl)
            n574 = Split 1D Array(array=w990, index=w952) -> (second subarray=w989:dbl[])  [unwired: 1 out]
            n575 = Split 1D Array(array=w958, index=w952) -> (second subarray=w959:dbl[])  [unwired: 1 out]
            n576 = Array Max & Min(array=w958) -> (max value=w979:dbl, min value=w978:dbl)  [unwired: 2 out]
            n577 = local read "机械间隙值"() -> (w972:dbl)
            n578 = local read "总圈数标准"() -> (w964:dbl)
            n579 = local read "总圈数最大值"() -> (w965:dbl)
            n580 = Subtract(x=w979, y=w978) -> (x-y=w973:dbl)
            n581 = call "功能计算_何 截取位移右.vi"("位移数组"=w959, "拉压力数组"=w989, "半行程"=w957, "截取百分比"=w956) -> ("峰值扭矩"=w955:dbl, "平均扭矩"=w988:dbl, "扭差"=w954:dbl)  [unwired: 12 in, 1 out]
            "右最大轴向力(N)" <- w955
            "右轴向力波动(N)" <- w954
            n582 = Subtract(x=w973, y=w972) -> (x-y=w970:dbl)
            n583 = Split 1D Array(array=w987, index=w952) -> (second subarray=w986:dbl[])  [unwired: 1 out]
            n584 = Greater?(x=w985, y=w983) -> (0:w975:bool)
            n585 = Greater?(x=w984, y=w983) -> (0:w974:bool)
            n586 = call "间隙计算.vi"("扭矩数组"=w986) -> ("峰值间隙1"=w981:dbl, "峰值间隙2"=w980:dbl)  [unwired: 6 in, 3 out]
            n587 = Divide(x=w970, y=w960) -> (x/y=w963:dbl)
            n588 = In Range and Coerce(upper limit=w965, x=w963, lower limit=w964) -> (In Range?=w962:bool)  [unwired: 1 out]
            n589 = Not(x=w962) -> (.not. x?=w961:bool)
            n590 = property on="总圈数" class="DigNum (严格)"("Blinking"=w961) -> ()  [unwired: 2 in, 2 out]
            n591 = property on="左全行程间隙" class="DigNum (严格)"("Blinking"=w975) -> ()  [unwired: 2 in, 2 out]
            n592 = property on="右全行程间隙" class="DigNum (严格)"("Blinking"=w974) -> ()  [unwired: 2 in, 2 out]
            n593 = local write "右平均轴向力(N)"(w988) -> ()
            n594 = local write "总圈数"(w963) -> ()
            n595 = local read "180°内全行程间隙标准(mm)"() -> (w982:dbl)
            n596 = local read "总行程标准(mm)"() -> (w968:dbl)
            n597 = local read "总行程最大值"() -> (w969:dbl)
            n598 = In Range and Coerce(upper limit=w969, x=w970, lower limit=w968) -> (In Range?=w967:bool)  [unwired: 1 out]
            n599 = local write "右180°外全行程间隙"(w980) -> ()
            n600 = local write "右180°内全行程间隙"(w981) -> ()
            n601 = local read "180°外全行程间隙标准(mm)"() -> (w971:dbl)
            n602 = local read "最大轴向力标准(N)"() -> (w953:dbl)
            n603 = Not(x=w967) -> (.not. x?=w966:bool)
            n604 = local write "总行程"(w970) -> ()
            n605 = property on="总行程" class="DigNum (严格)"("Blinking"=w966) -> ()  [unwired: 2 in, 2 out]
            "轴向力X" <- w958
            "轴向力Y" <- w990
          }
          frame #21 {
            n606 = local read "电动缸快速"() -> (w993:dbl)
            n607 = local read "轴向力标准(N)"() -> (w1007:dbl)
            n608 = local read "平均轴向力标准(N) max"() -> (w1006:dbl)
            n609 = Greater?(x=w1013, y=w1014) -> (0:w999:bool)
            n610 = Greater?(x=w1012, y=w997) -> (0:w998:bool)
            n611 = local write "电动缸速度(mm/s)"(w993) -> ()
            n612 = local read "转向器中心"() -> (w1015:dbl)
            n613 = local read "力波动标准(N)"() -> (w1005:dbl)
            n614 = call "判断.vi"("y 3"=w1005, "y 2-2"=w1006, "y 2-1"=w1007, "y"=w994, "x 3"=w1008, "x 2"=w1018, "x"=w1009) -> ("非x? 3"=w1002:bool, "非x? 2"=w1010:bool, "非x?"=w1011:bool)  [unwired: 2 in]
            n615 = property on="右180°内全行程间隙" class="DigNum (严格)"("Blinking"=w999) -> ()  [unwired: 2 in, 2 out]
            n616 = property on="右180°外全行程间隙" class="DigNum (严格)"("Blinking"=w998) -> ()  [unwired: 2 in, 2 out]
            n617 = Add(x=w1015, y=0.0) -> (x+y=w1016:dbl)
          }
          frame #22 {
            n618 = Compound Arithmetic op=OR(w1026, w1025, w1024, w1023) -> (w1022:bool)
            n619 = property on="右最大轴向力(N)" class="DigNum (严格)"("Blinking"=w1029) -> ()  [unwired: 2 in, 2 out]
            n620 = property on="右平均轴向力(N)" class="DigNum (严格)"("Blinking"=w1028) -> ()  [unwired: 2 in, 2 out]
            n621 = property on="右轴向力波动(N)" class="DigNum (严格)"("Blinking"=w1027) -> ()  [unwired: 2 in, 2 out]
            n622 = Compound Arithmetic op=OR(w1020, w1022, w1029, w1027, w1031, w1030, w1021) -> (w1033:bool)
            n623 = Not(x=w1033) -> (.not. x?=w1032:bool)
            n624 = local write "轴向力及全行程间隙合格"(w1032) -> ()
          }
          frame #23 {
            n625 = while {
              tunnel: w1038 -> [w1042]
              tunnel: [w1040] -> w1037
              tunnel: w1036 -> [w1039]
              stop <- w1041 stop-if-true
              n626 = call "PCI1240电动缸位置模式 .vi"("Distance"=w1039, "AxisHandle IN"=w1042) -> ("AbsSuccess"=w1041:bool, "AxisHandle OUT"=w1040:u32)  [unwired: 8 in]
              n627 = Wait (ms)(milliseconds to wait=u32 50 ("毫秒倍数")) -> ()  [unwired: 1 out]
            }
          }
          frame #24 {
            n628 = while {
              tunnel: w1045 -> [w1050]
              tunnel: [w1046] -> w1044
              stop <- w1048 stop-if-true
              n629 = call <userlib>:"Acm_AxGetCmdVelocity.vi"("AxisHandle"=w1050) -> ("Velocity"=w1049:dbl, "AxisHandle"=w1046:u32)  [unwired: 1 in, 2 out]
              n630 = Wait Until Next ms Multiple(millisecond multiple=u32 50 ("毫秒倍数")) -> ()  [unwired: 1 out]
              n631 = Equal To 0?(x=w1049) -> (x = 0?=w1048:bool)
            }
          }
          frame #25 {
            n632 = call "PCI1220U停止.vi"("AxisHandle IN"=w1051) -> ()  [unwired: 9 in, 2 out]
          }
          frame #26 {
            n633 = local read "轴向力已做次数"() -> (w1054:dbl)
            n634 = Add(x=w1054, y=1.0) -> (x+y=w1052:dbl)
            n635 = local write "轴向力已做次数"(w1052) -> ()
          }
          frame #27 {
            n636 = local read "轴向力及全行程间隙合格"() -> (w1055:bool)
            n637 = case shown="假" w1055 {
              frame False {
                n638 = Less?(x="轴向力已做次数", y="轴向力设定次数") -> (x < y?=w1057:bool)
                n639 = case shown="假" w1057 {
                  frame False {
                    n640 = local write "工步号"(u32 45 ("工步号")) -> ()
                  }
                  frame True {
                    n641 = local write "工步号"(u32 30 ("工步号")) -> ()
                  }
                }
              }
              frame True {
                n642 = local write "工步号"(u32 45 ("工步号")) -> ()
              }
            }
          }
        }
      }
      frame 45 {
        # "测头退回"
        n643 = flat-sequence {
          tunnel: [w1065] -> w1062
          tunnel: w1062 -> [w1072]
          frame #0 {
            n644 = local write "测头机构轴速度(mm/s)"(30.0 ("测头机构轴速度(mm/s)")) -> ()
          }
          frame #1 {
            n645 = local read "测头机构轴后退位"() -> (w1064:dbl)
            n646 = local read "测头机构电机"() -> (w1066:u32)
            n647 = while {
              tunnel: w1066 -> [w1070]
              tunnel: w1064 -> [w1069]
              tunnel: [w1068] -> w1065
              stop <- w1071 stop-if-true
              n648 = Wait Until Next ms Multiple(millisecond multiple=u32 50 ("毫秒倍数")) -> ()  [unwired: 1 out]
              n649 = call "PCI1220U进给轴位置模式.vi"("Distance"=w1069, "AxisHandle IN"=w1070) -> ("AbsSuccess"=w1071:bool, "AxisHandle OUT"=w1068:u32)  [unwired: 8 in]
            }
          }
          frame #2 {
            n650 = while {
              tunnel: w1072 -> [w1076]
              stop <- w1074 stop-if-true
              n651 = call <userlib>:"Acm_AxGetCmdVelocity.vi"("AxisHandle"=w1076) -> ("Velocity"=w1075:dbl)  [unwired: 1 in, 3 out]
              n652 = Wait Until Next ms Multiple(millisecond multiple=u32 50 ("毫秒倍数")) -> ()  [unwired: 1 out]
              n653 = Equal To 0?(x=w1075) -> (x = 0?=w1074:bool)
            }
          }
          frame #3 {
            n654 = while {
              stop <- w1078 stop-if-true
              n655 = local read "测头机构轴位置(mm)"() -> (w1080:dbl)
              n656 = Wait Until Next ms Multiple(millisecond multiple=u32 50 ("毫秒倍数")) -> ()  [unwired: 1 out]
              n657 = Less Or Equal?(x=w1080, y=35.0) -> (x <= y?=w1078:bool)
            }
          }
          frame #4 {
            n658 = local write "测头气缸右移"(FALSE ("测头气缸右移")) -> ()
            n659 = local write "测头气缸左移"(TRUE ("测头气缸左移")) -> ()
          }
          frame #5 {
            n660 = Wait Until Next ms Multiple(millisecond multiple=u32 500 ("毫秒倍数")) -> ()  [unwired: 1 out]
          }
          frame #6 {
            n661 = local write "工步号"(u32 50 ("工步号")) -> ()
          }
        }
      }
      frame 50 {
        n662 = flat-sequence {
          tunnel: [w1107] -> w1096
          tunnel: w1096 -> [w1114]
          tunnel: [w1113] -> w1093
          tunnel: w1093 -> [w1125]
          tunnel: [w1131] -> w1090
          tunnel: w1090 -> [w1134]
          tunnel: [w1133] -> w1089
          tunnel: w1089 -> [w1138]
          tunnel: [w1138] -> w1088
          tunnel: w1088 -> [w1140]
          tunnel: [w1139] -> w1086
          tunnel: [w1146] -> w1087
          tunnel: w1086 -> [w1147]
          tunnel: w1087 -> [w1149]
          tunnel: [w1148] -> w1085
          tunnel: [w1155] -> w1095
          tunnel: w1085 -> [w1155]
          tunnel: w1095 -> [w1158]
          tunnel: [w1157] -> w1094
          tunnel: w1094 -> [w1164]
          tunnel: [w1165] -> w1092
          tunnel: w1092 -> [w1172]
          tunnel: [w1171] -> w1091
          tunnel: w1091 -> [w1182]
          frame #0 {
            n663 = local write "旋转齿条轴速度(°/s)"(15.0 ("调整螺塞轴速度(°/s)")) -> ()
            n664 = local write "测头机构轴速度(mm/s)"(15.0 ("调整机构轴速度(mm/s)")) -> ()
            n665 = local write "电动缸速度(mm/s)"(15.0 ("电动缸速度(mm/s)")) -> ()
            n666 = local write "夹头夹紧"(FALSE ("夹头夹紧")) -> ()
            n667 = local write "夹头松开"(TRUE ("夹头松开")) -> ()
          }
          frame #1 {
            n668 = while {
              stop <- w1102 stop-if-true
              n669 = local read "夹头松开"() -> (w1103:bool)
              n670 = local read "夹头夹紧"() -> (w1105:bool)
              n671 = Wait Until Next ms Multiple(millisecond multiple=u32 50 ("毫秒倍数")) -> ()  [unwired: 1 out]
              n672 = Not(x=w1105) -> (.not. x?=w1104:bool)
              n673 = And(x=w1104, y=w1103) -> (x .and. y?=w1102:bool)
            }
          }
          frame #2 {
            n674 = while {
              tunnel: [w1110] -> w1107
              stop <- w1109 stop-if-true
              n675 = local read "电动缸电机"() -> (w1111:u32)
              n676 = Wait Until Next ms Multiple(millisecond multiple=u32 50 ("毫秒倍数")) -> ()  [unwired: 1 out]
              n677 = local read "齿条右极限"() -> (w1108:dbl)
              n678 = call "PCI1240电动缸位置模式 .vi"("Distance"=w1108, "AxisHandle IN"=w1111) -> ("AbsSuccess"=w1109:bool, "AxisHandle OUT"=w1110:u32)  [unwired: 8 in]
            }
          }
          frame #3 {
            n679 = while {
              tunnel: w1114 -> [w1123]
              tunnel: [w1115] -> w1113
              stop <- w1116 stop-if-true
              n680 = local read "齿条推拉力(N)"() -> (w1121:dbl)
              n681 = Wait Until Next ms Multiple(millisecond multiple=u32 50 ("毫秒倍数")) -> ()  [unwired: 1 out]
              n682 = call <userlib>:"Acm_AxGetCmdVelocity.vi"("AxisHandle"=w1123) -> ("Velocity"=w1124:dbl, "AxisHandle"=w1115:u32)  [unwired: 1 in, 2 out]
              n683 = Equal To 0?(x=w1124) -> (x = 0?=w1118:bool)
              n684 = Absolute Value(x=w1121) -> (abs(x)=w1120:dbl)
              n685 = Greater Or Equal?(x=w1120, y=1000.0) -> (x >= y?=w1117:bool)
              n686 = Or(x=w1118, y=w1117) -> (x .or. y?=w1116:bool)
            }
          }
          frame #4 {
            n687 = while {
              tunnel: w1125 -> [w1129]
              tunnel: [w1128] -> _
              stop <- w1127 stop-if-true
              n688 = call "PCI1220U停止.vi"("AxisHandle IN"=w1129) -> ("完成"=w1127:bool, "AxisHandle OUT"=w1128:u32)  [unwired: 9 in]
              n689 = Wait (ms)(milliseconds to wait=u32 50 ("毫秒倍数")) -> ()  [unwired: 1 out]
            }
          }
          frame #5 {
            n690 = local write "旋转齿条轴使能"(TRUE ("旋转齿条轴使能")) -> ()
          }
          frame #6 {
            n691 = local read "旋转齿条电机"() -> (w1131:u32)
            n692 = Wait Until Next ms Multiple(millisecond multiple=u32 500 ("毫秒倍数")) -> ()  [unwired: 1 out]
          }
          frame #7 {
            n693 = call <userlib>:"Acm_AxHome.vi"("DirMode"=u32 0, "HomeMode"=u32 11, "AxisHandle"=w1134) -> ("AxisHandle"=w1133:u32)  [unwired: 1 in, 2 out]
          }
          frame #8 {
            n694 = Wait Until Next ms Multiple(millisecond multiple=u32 100 ("毫秒倍数")) -> ()  [unwired: 1 out]
          }
          frame #9 {
            n695 = while {
              tunnel: w1140 -> [w1143]
              tunnel: [w1142] -> w1139
              stop <- w1141 stop-if-true
              n696 = call <userlib>:"Acm_AxGetCmdVelocity.vi"("AxisHandle"=w1143) -> ("Velocity"=w1145:dbl, "AxisHandle"=w1142:u32)  [unwired: 1 in, 2 out]
              n697 = Wait Until Next ms Multiple(millisecond multiple=u32 50 ("毫秒倍数")) -> ()  [unwired: 1 out]
              n698 = Equal To 0?(x=w1145) -> (x = 0?=w1141:bool)
            }
          }
          frame #10 {
            n699 = call "PCI1220U角度置零.vi"("AxisHandle IN"=w1147) -> ("AxisHandle OUT"=w1146:u32)  [unwired: 10 in]
          }
          frame #11 {
            n700 = while {
              tunnel: w1149 -> [w1151]
              tunnel: [w1150] -> w1148
              stop <- w1154 stop-if-true
              n701 = Wait Until Next ms Multiple(millisecond multiple=u32 50 ("毫秒倍数")) -> ()  [unwired: 1 out]
              n702 = call "PCI1220U扭矩轴位置模式.vi"("Distance"=10.0, "AxisHandle IN"=w1151) -> ("AbsSuccess"=w1154:bool, "AxisHandle OUT"=w1150:u32)  [unwired: 8 in]
            }
          }
          frame #12 {
            n703 = Wait Until Next ms Multiple(millisecond multiple=u32 500 ("毫秒倍数")) -> ()  [unwired: 1 out]
          }
          frame #13 {
            n704 = while {
              tunnel: w1158 -> [w1161]
              tunnel: [w1160] -> w1157
              stop <- w1159 stop-if-true
              n705 = call <userlib>:"Acm_AxGetCmdVelocity.vi"("AxisHandle"=w1161) -> ("Velocity"=w1163:dbl, "AxisHandle"=w1160:u32)  [unwired: 1 in, 2 out]
              n706 = Wait Until Next ms Multiple(millisecond multiple=u32 50 ("毫秒倍数")) -> ()  [unwired: 1 out]
              n707 = Equal To 0?(x=w1163) -> (x = 0?=w1159:bool)
            }
          }
          frame #14 {
            n708 = call "PCI1220U角度置零.vi"("AxisHandle IN"=w1164) -> ()  [unwired: 10 in, 1 out]
          }
          frame #15 {
            n709 = while {
              tunnel: [w1168] -> w1165
              stop <- w1167 stop-if-true
              n710 = local read "电动缸电机"() -> (w1169:u32)
              n711 = Wait Until Next ms Multiple(millisecond multiple=u32 50 ("毫秒倍数")) -> ()  [unwired: 1 out]
              n712 = local read "齿条右极限"() -> (w1166:dbl)
              n713 = call "PCI1240电动缸位置模式 .vi"("Distance"=w1166, "AxisHandle IN"=w1169) -> ("AbsSuccess"=w1167:bool, "AxisHandle OUT"=w1168:u32)  [unwired: 8 in]
            }
          }
          frame #16 {
            n714 = while {
              tunnel: w1172 -> [w1180]
              tunnel: [w1178] -> w1171
              stop <- w1173 stop-if-true
              n715 = local read "齿条推拉力(N)"() -> (w1177:dbl)
              n716 = Wait Until Next ms Multiple(millisecond multiple=u32 50 ("毫秒倍数")) -> ()  [unwired: 1 out]
              n717 = call <userlib>:"Acm_AxGetCmdVelocity.vi"("AxisHandle"=w1180) -> ("Velocity"=w1181:dbl, "AxisHandle"=w1178:u32)  [unwired: 1 in, 2 out]
              n718 = Equal To 0?(x=w1181) -> (x = 0?=w1175:bool)
              n719 = Greater Or Equal?(x=w1177, y=300.0) -> (x >= y?=w1174:bool)
              n720 = Or(x=w1175, y=w1174) -> (x .or. y?=w1173:bool)
            }
          }
          frame #17 {
            n721 = while {
              tunnel: w1182 -> [w1186]
              tunnel: [w1185] -> _
              stop <- w1184 stop-if-true
              n722 = call "PCI1220U停止.vi"("AxisHandle IN"=w1186) -> ("完成"=w1184:bool, "AxisHandle OUT"=w1185:u32)  [unwired: 9 in]
              n723 = Wait (ms)(milliseconds to wait=u32 50 ("毫秒倍数")) -> ()  [unwired: 1 out]
            }
          }
          frame #18 {
            n724 = local write "工步号"(u32 100 ("工步号")) -> ()
          }
        }
      }
      frame 100 {
        n725 = flat-sequence {
          tunnel: [w1221] -> w1211
          tunnel: [w1219] -> w1210
          tunnel: [w1213] -> w1198
          tunnel: [w1212] -> w1195
          tunnel: w1211 -> [w1228]
          tunnel: w1210 -> [w1225]
          tunnel: ["F:\\报表存储\\" ("字符串")] -> w1209
          tunnel: w1198 -> [w1227]
          tunnel: [w1228] -> w1197
          tunnel: [w1227] -> w1196
          tunnel: w1195 -> [w1226]
          tunnel: [w1226] -> w1194
          tunnel: [w1225] -> w1193
          tunnel: w1209 -> [w1240]
          tunnel: [w1247] -> w1208
          tunnel: [w1245] -> w1207
          tunnel: [w1244] -> w1206
          tunnel: [w1243] -> w1205
          tunnel: w1197 -> [w1239]
          tunnel: w1196 -> [w1238]
          tunnel: w1194 -> [w1237]
          tunnel: w1193 -> [w1230]
          tunnel: [w1232] -> w1188
          tunnel: w1208 -> [w1254]
          tunnel: [w1255] -> w1204
          tunnel: w1207 -> [w1255]
          tunnel: w1206 -> [w1253]
          tunnel: w1205 -> [w1252]
          tunnel: [w1251] -> w1203
          tunnel: [w1250] -> w1202
          tunnel: [w1249] -> w1189
          tunnel: w1188 -> [w1249]
          tunnel: [w1262] -> w1201
          tunnel: w1204 -> [w1262]
          tunnel: w1203 -> [w1261]
          tunnel: [w1261] -> w1200
          tunnel: [w1260] -> w1199
          tunnel: w1202 -> [w1260]
          tunnel: [w1258] -> w1190
          tunnel: w1189 -> [w1258]
          tunnel: w1201 -> [w1265]
          tunnel: w1200 -> [w1273]
          tunnel: w1199 -> [w1272]
          tunnel: [w1264] -> w1191
          tunnel: w1190 -> [w1264]
          tunnel: [w1281] -> w1192
          tunnel: w1191 -> [w1281]
          tunnel: w1192 -> [w1283]
          frame #0 {
            n726 = local read "产品ID"() -> (w1220:string)
            n727 = Format Date/Time String(time format string (%c)="%Y%m%d" ("时间格式字符串(%c)")) -> (date/time string=w1214:string)  [unwired: 2 in]
            n728 = String Subset(string=w1214, offset (0)=6 ("偏移量(0)"), length (rest)=2 ("长度（剩余）")) -> (substring=w1212:string)
            n729 = String Subset(string=w1214, offset (0)=4 ("偏移量(0)"), length (rest)=2 ("长度（剩余）")) -> (substring=w1213:string)
            n730 = String Subset(string=w1214, offset (0)=0 ("偏移量(0)"), length (rest)=4 ("长度（剩余）")) -> (substring=w1221:string)
            n731 = call <vilib>:"Trim Whitespace.vi"("string"=w1220) -> ("trimmed string"=w1219:string)  [unwired: 1 in]
          }
          frame #1 {
          }
          frame #2 {
            w1231 = "\\" ("字符串")
            n732 = Concatenate Strings(w1240, w1239, w1231, w1238, w1231, w1237, w1231, w1230, w1231) -> (w1234:string)
            n733 = Concatenate Strings(w1240, w1239, w1231, w1238, w1231, w1237, w1231, w1230, w1231) -> (w1248:string)
            n734 = Concatenate Strings(w1234, w1230, "间隙曲线.JPG" ("字符串")) -> (w1246:string)
            n735 = Concatenate Strings(w1234, "轴向力曲线数组.txt" ("字符串")) -> (w1243:string)
            n736 = Concatenate Strings(w1234, "扭动曲线数组.txt" ("字符串")) -> (w1244:string)
            n737 = Concatenate Strings(w1234, w1230, "轴向力曲线.JPG" ("字符串")) -> (w1236:string)
            n738 = String To Path(string=w1246) -> (path=w1245:path)
            n739 = String To Path(string=w1248) -> (path=w1247:path)
            n740 = String To Path(string=w1236) -> (path=w1232:path)
          }
          frame #3 {
            n741 = call <vilib>:"Check if File or Folder Exists.vi"("path"=w1254) -> ("file or folder exists?"=w1256:bool)  [unwired: 8 in, 2 out]
            n742 = case shown="假" w1256 {
              tunnel: w1254 -> [w1257 _]
              frame False {
                n743 = Create Folder(path (use dialog)=w1257) -> ()  [unwired: 2 in, 3 out]
              }
              frame True {
              }
            }
            n744 = String To Path(string=w1252) -> (path=w1250:path)
            n745 = String To Path(string=w1253) -> (path=w1251:path)
          }
          frame #4 {
            n746 = local write "选项卡控件"(T1."间隙测量" ("选项卡控件")) -> ()
            n747 = Wait Until Next ms Multiple(millisecond multiple=u32 1000 ("毫秒倍数")) -> ()  [unwired: 1 out]
          }
          frame #5 {
            n748 = disable-structure shown="禁用" {
              disable-tunnel: w1265 -> [w1274 _]
              frame Disabled {
                w1278 = T2 2 items=["快速打印", "标准报表", "HTML", "双字节", "Excel"] ("report type (Quick Print)")
                w1277 = T3 1 items=["完整前面板", "前面板可见部分", "图标、说明、前面板和程序框图", "说明信息: 使用前面板", "说明信息: 作为子VI使用", "说明信息: 完整", "说明信息: 自定义"] ("contents (complete front panel)")
                n749 = Current VI's Path() -> (path=w1276:path)
                n750 = call-poly <vilib>:"Easy Print VI Panel or Documentation.vi"("report type (Quick Print)"=w1278, "contents (complete front panel)"=w1277, "VI path"=w1276) -> ("error out"=w1280:errorcluster, "report out"=w1279:refnum<class "NI_report.lvclass">)  [unwired: 1 in, 6 out]
                n751 = call-dynamic "Save Report to File.vi"("report in"=w1279, "report file path"=w1274, "error in (no error)"=w1280) -> ("error out"=→"error out 3":errorcluster)  [unwired: 2 in, 10 out]
              }
              frame Enabled {
              }
            }
            n752 = local read "间隙Y数组"() -> (w1270:dbl[])
            n753 = local read "间隙X数组"() -> (w1271:dbl[])
            n754 = local read "轴向力Y"() -> (w1268:dbl[])
            n755 = local read "轴向力X"() -> (w1269:dbl[])
            n756 = call "导出曲线数组.vi"("file path (dialog if empty)"=w1273, "数组 2"=w1270, "数组"=w1271) -> ()  [unwired: 9 in]
            n757 = call "导出曲线数组.vi"("file path (dialog if empty)"=w1272, "数组 2"=w1268, "数组"=w1269) -> ()  [unwired: 9 in]
            n758 = control-ref of="本VI"() -> (w1267:refnum<vi>)
            n759 = invoke class="VI" method="FP.Get Image"(reference=w1267) -> ("image data"=w1266:T4)  [unwired: 5 in, 5 out]
            n760 = call <vilib>:"Write JPEG File.vi"("image data"=w1266, "path to JPEG file"=w1265) -> ()  [unwired: 8 in, 2 out]
          }
          frame #6 {
            n761 = local write "选项卡控件"(T1."轴向力测量" ("选项卡控件")) -> ()
          }
          frame #7 {
            n762 = control-ref of="本VI"() -> (w1284:refnum<vi>)
            n763 = invoke class="VI" method="FP.Get Image"(reference=w1284) -> ("image data"=w1285:T4)  [unwired: 5 in, 5 out]
            n764 = call <vilib>:"Write JPEG File.vi"("image data"=w1285, "path to JPEG file"=w1283) -> ()  [unwired: 8 in, 2 out]
          }
          frame #8 {
            n765 = local read "联线按钮"() -> (w1286:bool)
            n766 = case shown="真" w1286 {
              frame False {
              }
              frame True {
                n767 = flat-sequence {
                  tunnel: [w1289] -> w1287
                  tunnel: [w1317] -> w1288
                  tunnel: w1287 -> [w1313]
                  tunnel: w1288 -> [w1329]
                  frame #0 {
                    n768 = local read "轴向力及全行程间隙合格"() -> (w1290:bool)
                    n769 = local read "单点间隙合格"() -> (w1291:bool)
                    n770 = And(x=w1291, y=w1290) -> (x .and. y?=w1289:bool)
                  }
                  frame #1 {
                    w1311 = i16 3 ("精度(6)")
                    n771 = local read "右180°内全行程间隙"() -> (w1310:dbl)
                    n772 = local read "右180°外全行程间隙"() -> (w1303:dbl)
                    n773 = local read "左180°外全行程间隙"() -> (w1302:dbl)
                    n774 = local read "左180°内全行程间隙"() -> (w1320:dbl)
                    n775 = local read "右最大轴向力(N)"() -> (w1305:dbl)
                    n776 = local read "左轴向力波动(N)"() -> (w1306:dbl)
                    n777 = local read "左最大轴向力(N)"() -> (w1304:dbl)
                    n778 = local read "员工ID"() -> (w1292:string)
                    n779 = local read "右轴向力波动(N)"() -> (w1307:dbl)
                    n780 = Boolean To (0,1)(Boolean=w1313) -> (0, 1=w1315:i16)
                    n781 = local read "中间位置间隙"() -> (w1322:dbl)
                    n782 = local read "总圈数"() -> (w1309:dbl)
                    n783 = local read "总行程"() -> (w1308:dbl)
                    n784 = local read "FGCS"() -> (w1324:string)
                    n785 = local read "KSJJ"() -> (w1326:string)
                    n786 = local read "产品ID"() -> (w1327:string)
                    n787 = Number To Decimal String(number=w1315, width (-)=i16 1 ("宽度(-)")) -> (decimal integer string=w1312:string)
                    n788 = Format Date/Time String(time format string (%c)="%Y%m%d%H%M" ("时间格式字符串(%c)")) -> (date/time string=w1325:string)  [unwired: 2 in]
                    n789 = Number To Fractional String(number=w1308, precision (6)=w1311) -> (F-format string=w1294:string)  [unwired: 2 in]
                    n790 = Number To Fractional String(number=w1303, precision (6)=w1311) -> (F-format string=w1299:string)  [unwired: 2 in]
                    n791 = Number To Fractional String(number=w1306, precision (6)=w1311) -> (F-format string=w1296:string)  [unwired: 2 in]
                    n792 = Number To Fractional String(number=w1310, precision (6)=w1311) -> (F-format string=w1301:string)  [unwired: 2 in]
                    n793 = Number To Fractional String(number=w1305, precision (6)=w1311) -> (F-format string=w1297:string)  [unwired: 2 in]
                    n794 = Number To Fractional String(number=w1307, precision (6)=w1311) -> (F-format string=w1295:string)  [unwired: 2 in]
                    n795 = Number To Fractional String(number=w1320, precision (6)=w1311) -> (F-format string=w1318:string)  [unwired: 2 in]
                    n796 = Number To Fractional String(number=w1304, precision (6)=w1311) -> (F-format string=w1298:string)  [unwired: 2 in]
                    n797 = Number To Fractional String(number=w1309, precision (6)=w1311) -> (F-format string=w1293:string)  [unwired: 2 in]
                    n798 = Number To Fractional String(number=w1302, precision (6)=w1311) -> (F-format string=w1300:string)  [unwired: 2 in]
                    n799 = Number To Fractional String(number=w1322, precision (6)=i16 3 ("精度(6)")) -> (F-format string=w1319:string)  [unwired: 2 in]
                    n800 = Build Array(w1327, w1292, "1", w1312, w1326, w1325, w1324, "Q14073-11A", w1319, w1318, w1301, w1300, w1299, w1298, w1297, w1296, w1295, w1294, w1293) -> (w1317:string[])
                  }
                  frame #2 {
                    n801 = Wait (ms)(milliseconds to wait=u32 500 ("等待时间（毫秒）")) -> ()  [unwired: 1 out]
                    n802 = call "数据库更新.vi"("设备号"="06", "数据"=w1329) -> ()  [unwired: 13 in, 1 out]
                  }
                  frame #3 {
                  }
                }
              }
            }
          }
          frame #9 {
            n803 = local write "产品ID"("") -> ()
            n804 = local write "工步号"(u32 0 ("工步号")) -> ()
          }
        }
      }
    }
    n805 = Wait (ms)(milliseconds to wait=u32 50 ("毫秒倍数")) -> ()  [unwired: 1 out]
    n806 = local read "停止"() -> (w7:bool)
  }
  n807 = while {
    stop <- w1334 stop-if-true
    n808 = event shown="[2] \"参数修改\": 值改变" {
      selector: _ -> [_ _ _ _ _ _]
      dyn-events: _ -> [_ _ _ _ _ _]
      timeout: 500 -> [_ _ _ _ _ _]
      event Timeout {
        n809 = event-data() -> ()  [unwired: 3 out]
      }
      event "停止": Value Change {
        n810 = event-data() -> ()  [unwired: 6 out]
        n811 = flat-sequence {
          frame #0 {
            n812 = Wait (ms)(milliseconds to wait=u32 1000 ("毫秒倍数")) -> ()  [unwired: 1 out]
          }
          frame #1 {
            n813 = Quit LabVIEW(quit? (T)=TRUE ("停止？(T)")) -> ()
          }
        }
      }
      event "参数修改": Value Change {
        n814 = event-data() -> ()  [unwired: 6 out]
        n815 = while {
          i -> [w1341]
          stop <- w1340 stop-if-true
          n816 = local read "参数浏览表"() -> (w1343:string[][])
          n817 = local read "型号数量"() -> (w1342:i32)
          n818 = Wait Until Next ms Multiple(millisecond multiple=u32 50 ("毫秒倍数")) -> ()  [unwired: 1 out]
          n819 = Greater Or Equal?(x=w1341, y=w1342) -> (x >= y?=w1340:bool)
          n820 = Index Array(array=w1343, index (col)=w1341) -> (element=w1339:string[])  [unwired: 1 in]
          n821 = stacked-sequence {
            tunnel: w1339 -> [w1385]
            frame #0 {
              n822 = Index Array(array=w1385, index #1=0 ("索引"), index #2=2 ("索引"), index #3=3 ("索引"), index #4=4 ("索引"), index #5=5 ("索引"), index #6=6 ("索引"), index #7=7 ("索引"), index #8=8 ("索引"), index #9=9 ("索引"), index #10=10 ("索引"), index #11=11 ("索引"), index #12=12 ("索引"), index #13=13 ("索引"), index #14=14 ("索引"), index #15=15 ("索引"), index #16=16 ("索引"), index #17=17 ("索引"), index #18=18 ("索引"), index #19=19 ("索引"), index #20=20 ("索引"), index #21=21 ("索引"), index #22=22 ("索引"), index #23=23 ("索引")) -> (element #1=w1345:string, element #2=w1381:string, element #3=w1380:string, element #4=w1379:string, element #5=w1378:string, element #6=w1377:string, element #7=w1376:string, element #8=w1375:string, element #9=w1374:string, element #10=w1373:string, element #11=w1372:string, element #12=w1363:string, element #13=w1362:string, element #14=w1361:string, element #15=w1360:string, element #16=w1359:string, element #17=w1358:string, element #18=w1355:string, element #19=w1354:string, element #20=w1352:string, element #21=w1351:string, element #22=w1350:string, element #23=w1349:string)
              n823 = call "创建文本"("测头机构轴移动速度"=w1381, "测头机构轴检测位"=w1380, "测头机构轴待检位"=w1379, "测头机构轴后退位"=w1378, "齿条移动速度"=w1377, "齿条左极限"=w1376, "齿条右极限"=w1375, "旋转齿条轴找帽转速"=w1374, "旋转齿条轴测量转速"=w1373, "测量点扭矩"=w1372, "总行程最小值"=w1363, "总行程最大值"=w1362, "最大轴向力"=w1361, "轴向力波动"=w1360, "平均轴向力最小值"=w1359, "平均轴向力最大值"=w1358, "总圈数最小值"=w1355, "总圈数最大值"=w1354, "中间位置"=w1352, "中间间隙标准"=w1351, "180内间隙标准"=w1350, "180外间隙标准"=w1349, "产品型号"=w1345) -> ("Result"=w1371:string)  [unwired: 3 in, 1 out]
              n824 = local read "ADODB._Connection Out 2"() -> (w1370:refnum<k7>)
              n825 = call "SQL Execute.vi"("Command Text"=w1371, "ADODB._Connection In"=w1370) -> ("error out"=w1383:errorcluster, "ADODB._Connection Out"=w1384:refnum<k7>)  [unwired: 6 in, 2 out]
              n826 = call "ADO Connection Close.vi"("error in (no error)"=w1383, "ADODB._Connection In"=w1384) -> ("error out"=→"error out":errorcluster)  [unwired: 8 in, 1 out]
            }
          }
        }
      }
      event "参数查询": Value Change {
        n827 = event-data() -> ()  [unwired: 6 out]
        n828 = flat-sequence {
          tunnel: [w1408] -> w1401
          tunnel: [w1407] -> w1400
          tunnel: [w1406] -> w1397
          tunnel: w1401 -> [w1412]
          tunnel: w1400 -> [w1414]
          tunnel: [w1414] -> w1399
          tunnel: [w1413] -> w1398
          tunnel: w1397 -> [w1413]
          tunnel: w1399 -> [_]
          tunnel: w1398 -> [_]
          frame #0 {
            n829 = call-poly <vilib>:"Read From Spreadsheet File.vi"("file path (dialog if empty)"=path "D:/Q14070-Z060人机界面/参数/参数项.txt") -> ("first row"=w1402:string[])  [unwired: 6 in, 4 out]
            n830 = property on="参数浏览表" class="Tbl (严格)"("Row Headers[]"=w1402) -> ()  [unwired: 2 in, 2 out]
          }
          frame #1 {
            n831 = local read "ADODB._Connection Out 2"() -> (w1405:refnum<k7>)
            n832 = call "SQL Execute.vi"("Command Text"="SELECT * FROM 测试参数表;", "ADODB._Connection In"=w1405) -> ("error out"=w1406:errorcluster, "Data"=w1410:string[][], "ADODB._Connection Out"=w1407:refnum<k7>)  [unwired: 6 in, 1 out]
            n833 = Transpose 2D Array "二维数组转置"(2D array=w1410) -> (transposed array=w1408:string[][])
            n834 = Index Array(array=w1408, index (row)=0 ("索引 (行)")) -> (element=w1409:string[])  [unwired: 1 in]
            n835 = property on="参数浏览表" class="Tbl (严格)"("Column Headers[]"=w1409) -> ()  [unwired: 2 in, 2 out]
          }
          frame #2 {
            n836 = local write "参数浏览表"(w1412) -> ()
          }
          frame #3 {
          }
        }
      }
      event "传感器参数保存": Value Change {
        n837 = event-data() -> ()  [unwired: 6 out]
        n838 = flat-sequence {
          frame #0 {
            n839 = local read "齿条推拉力零点偏移"() -> (w1419:dbl)
            n840 = local read "齿条推拉力比例偏移"() -> (w1415:dbl)
            n841 = local read "间隙位移零点偏移"() -> (w1426:dbl)
            n842 = local read "齿条扭矩零点偏移"() -> (w1418:dbl)
            n843 = local read "间隙位移比例偏移"() -> (w1416:dbl)
            n844 = local read "齿条扭矩比例偏移"() -> (w1417:dbl)
            n845 = local read "ADODB._Connection Out 2"() -> (w1434:refnum<k7>)
            n846 = Number To Fractional String(number=w1426, precision (6)=i16 2 ("精度(6)")) -> (F-format string=w1433:string)  [unwired: 2 in]
            n847 = Number To Fractional String(number=w1419, precision (6)=i16 2 ("精度(6)")) -> (F-format string=w1432:string)  [unwired: 2 in]
            n848 = Number To Fractional String(number=w1418, precision (6)=i16 2 ("精度(6)")) -> (F-format string=w1431:string)  [unwired: 2 in]
            n849 = Number To Fractional String(number=w1416, precision (6)=i16 2 ("精度(6)")) -> (F-format string=w1430:string)  [unwired: 2 in]
            n850 = Number To Fractional String(number=w1415, precision (6)=i16 2 ("精度(6)")) -> (F-format string=w1429:string)  [unwired: 2 in]
            n851 = Number To Fractional String(number=w1417, precision (6)=i16 2 ("精度(6)")) -> (F-format string=w1428:string)  [unwired: 2 in]
            n852 = call "创建文本3"("4"=w1430, "6"=w1428, "1"=w1433, "2"=w1432, "3"=w1431, "5"=w1429) -> ("Result"=w1435:string)  [unwired: 8 in, 1 out]
            n853 = call "SQL Execute.vi"("Command Text"=w1435, "ADODB._Connection In"=w1434) -> ("error out"=→"error out 4":errorcluster)  [unwired: 6 in, 3 out]
          }
        }
      }
      event "产品ID": Value Change {
        n854 = event-data() -> ()  [unwired: 7 out]
        n855 = Format Date/Time String(time format string (%c)="%Y%m%d%H%M" ("时间格式字符串(%c)")) -> (date/time string=w1436:string)  [unwired: 2 in]
        n856 = local write "KSJJ"(w1436) -> ()
      }
    }
    n857 = Wait (ms)(milliseconds to wait=u32 50 ("毫秒倍数")) -> ()  [unwired: 1 out]
    n858 = local read "停止"() -> (w1334:bool)
  }
  n859 = while {
    stop <- w1439 stop-if-true
    n860 = stacked-sequence {
      frame #0 {
        n861 = flat-sequence {
          frame #0 {
          }
          frame #1 {
            "PLC" <- "阻挡"
          }
          frame #2 {
            n862 = First Call?() -> (First Call?: T/F=w1441:bool)
            n863 = case shown="真" w1441 {
              frame False {
              }
              frame True {
                n864 = call "员工管理测试程序.vi"() -> ("员工姓名"=w1443:string, "员工ID"=w1442:string)  [unwired: 10 in]
                n865 = local write "员工ID"(w1442) -> ()
                n866 = local write "员工姓名"(w1443) -> ()
              }
            }
          }
          frame #3 {
          }
          frame #4 {
          }
          frame #5 {
          }
          frame #6 {
          }
        }
      }
      frame #1 {
        n867 = flat-sequence {
          frame #0 {
            n868 = property on="型号选择" class="Ring (严格)"() -> ("RingText.Text"=w1447:string)  [unwired: 2 in, 2 out]
            n869 = case shown="\"J728\"" w1447 {
              frame "J709", Default {
                w1448 = FALSE ("可见")
                w1449 = TRUE ("可见")
                n870 = property on="右180°内全行程间隙" class="DigNum (严格)"("Visible"=w1448) -> ()  [unwired: 2 in, 2 out]
                n871 = property on="右180°外全行程间隙" class="DigNum (严格)"("Visible"=w1448) -> ()  [unwired: 2 in, 2 out]
                n872 = property on="左180°外全行程间隙" class="DigNum (严格)"("Visible"=w1448) -> ()  [unwired: 2 in, 2 out]
                n873 = property on="左180°内全行程间隙" class="DigNum (严格)"("Visible"=w1448) -> ()  [unwired: 2 in, 2 out]
                n874 = property on="右全行程间隙" class="DigNum (严格)"("Visible"=w1449) -> ()  [unwired: 2 in, 2 out]
                n875 = property on="左全行程间隙" class="DigNum (严格)"("Visible"=w1449) -> ()  [unwired: 2 in, 2 out]
              }
              frame "J706" {
                w1450 = TRUE ("可见")
                w1451 = FALSE ("可见")
                n876 = property on="右180°内全行程间隙" class="DigNum (严格)"("Visible"=w1450) -> ()  [unwired: 2 in, 2 out]
                n877 = property on="右180°外全行程间隙" class="DigNum (严格)"("Visible"=w1450) -> ()  [unwired: 2 in, 2 out]
                n878 = property on="左180°外全行程间隙" class="DigNum (严格)"("Visible"=w1450) -> ()  [unwired: 2 in, 2 out]
                n879 = property on="左180°内全行程间隙" class="DigNum (严格)"("Visible"=w1450) -> ()  [unwired: 2 in, 2 out]
                n880 = property on="右全行程间隙" class="DigNum (严格)"("Visible"=w1451) -> ()  [unwired: 2 in, 2 out]
                n881 = property on="左全行程间隙" class="DigNum (严格)"("Visible"=w1451) -> ()  [unwired: 2 in, 2 out]
              }
              frame "J728" {
                w1452 = TRUE ("可见")
                w1453 = FALSE ("可见")
                n882 = property on="右180°内全行程间隙" class="DigNum (严格)"("Visible"=w1452) -> ()  [unwired: 2 in, 2 out]
                n883 = property on="右180°外全行程间隙" class="DigNum (严格)"("Visible"=w1452) -> ()  [unwired: 2 in, 2 out]
                n884 = property on="左180°外全行程间隙" class="DigNum (严格)"("Visible"=w1452) -> ()  [unwired: 2 in, 2 out]
                n885 = property on="左180°内全行程间隙" class="DigNum (严格)"("Visible"=w1452) -> ()  [unwired: 2 in, 2 out]
                n886 = property on="右全行程间隙" class="DigNum (严格)"("Visible"=w1453) -> ()  [unwired: 2 in, 2 out]
                n887 = property on="左全行程间隙" class="DigNum (严格)"("Visible"=w1453) -> ()  [unwired: 2 in, 2 out]
              }
            }
          }
          frame #1 {
            (unwired) string[] ["I急停按钮", "I自动旋钮", "I启动按钮", "I备用按钮", "I复位按钮", "I上阻挡器放行", "I下阻挡器放行", "I进支线按钮"] ("I0说明")
            (unwired) string[] ["I出支线按钮", "I主线顶升按钮", "I主线下降按钮", "I支线顶升按钮", "I支线下降按钮", "I气压报警", "未使用", "未使用"] ("I0说明")
            n888 = local read "间隙位移(mm)"() -> (w1456:dbl)
            n889 = Greater Or Equal?(x=w1456, y=4.0) -> (x >= y?=w1454:bool)
            n890 = case shown="真" w1454 {
              frame False {
              }
              frame True {
                n891 = local write "测头机构轴使能"(FALSE ("测头机构轴使能")) -> ()
              }
            }
          }
          frame #2 {
            (unwired) string[] ["I电动缸SRDY", "I电动缸ZSPD", "I电动缸ALRM", "I间隙进给SRDY", "I间隙进给ZSPD", "I间隙进给ALRM", "I间隙旋转SRPD", "I间隙旋转ZSPD"] ("I0说明")
            n892 = local read "测头机构轴位置(mm)"() -> (w1460:dbl)
            n893 = Greater Or Equal?(x=w1460, y=90.0) -> (x >= y?=w1458:bool)
            n894 = case shown="假" w1458 {
              frame False {
                w1461 = T5."Enabled" ("禁用")
                n895 = property on="测头气缸右移" class="Bool"("DisabledEnum"=w1461) -> ()  [unwired: 2 in, 2 out]
                n896 = property on="测头气缸左移" class="Bool"("DisabledEnum"=w1461) -> ()  [unwired: 2 in, 2 out]
                n897 = property on="测头气缸右移" class="Bool (严格)"("DisabledEnum"=w1461) -> ()  [unwired: 2 in, 2 out]
                n898 = property on="测头气缸左移" class="Bool (严格)"("DisabledEnum"=w1461) -> ()  [unwired: 2 in, 2 out]
              }
              frame True {
                w1462 = T5."Disabled" ("禁用")
                w1463 = FALSE ("测头气缸右移")
                n899 = local write "测头气缸右移"(w1463) -> ()
                n900 = local write "测头气缸左移"(w1463) -> ()
                n901 = property on="测头气缸右移" class="Bool"("DisabledEnum"=w1462) -> ()  [unwired: 2 in, 2 out]
                n902 = property on="测头气缸左移" class="Bool"("DisabledEnum"=w1462) -> ()  [unwired: 2 in, 2 out]
                n903 = property on="测头气缸右移" class="Bool (严格)"("DisabledEnum"=w1462) -> ()  [unwired: 2 in, 2 out]
                n904 = property on="测头气缸左移" class="Bool (严格)"("DisabledEnum"=w1462) -> ()  [unwired: 2 in, 2 out]
              }
            }
          }
          frame #3 {
            (unwired) string[] ["I间隙旋转ALRM", "I扭矩旋转SRPD", "I扭矩旋转ZSPD", "I扭矩旋转ALRM", "I拧紧机合格", "I拧紧机不合格", "I拧紧机报警", "未使用"] ("I0说明")
          }
        }
        n905 = local read "急停"() -> (w1446:bool)
        n906 = local read "复位"() -> (w1445:bool)
        n907 = Compound Arithmetic op=OR(invert w1446, w1445) -> (→"循环退出":bool)
      }
      frame #2 {
        n908 = flat-sequence {
          frame #0 {
            (unwired) string[] ["I自制气缸进位", "I自制气缸原位", "I上工位检测", "I本工位检测", "I下工位检测", "I主线顶升上位", "I主线顶升下位", "I支线顶升上位"] ("I0说明")
          }
          frame #1 {
            (unwired) string[] ["I支线顶升下位", "I支线进到位", "I支线退到位", "I位移气缸原位", "I位移气缸进位", "I拧紧机在位", "I电动缸原位", "I电动缸进位"] ("I0说明")
          }
          frame #2 {
            (unwired) string[] ["未使用", "未使用", "未使用", "未使用", "未使用", "未使用", "未使用", "未使用"] ("I0说明")
          }
          frame #3 {
            (unwired) string[] ["未使用", "未使用", "未使用", "未使用", "未使用", "未使用", "未使用", "未使用"] ("I0说明")
          }
        }
        n909 = local read "本测试状态"() -> (w1465:bool)
        n910 = local read "本自动状态"() -> (w1466:bool)
        n911 = local read "本备料状态"() -> (w1464:bool)
        n912 = local write "本测试状态H"(w1465) -> ()
        n913 = local write "本自动状态H"(w1466) -> ()
        n914 = local write "本备料状态H"(w1464) -> ()
      }
      frame #3 {
        n915 = local read "报警工步号"() -> (w1468:dbl)
        n916 = local read "工步号"() -> (w1470:u32)
        n917 = case shown="0, 默认" w1470 {
          tunnel: [w1480 "请取胶瓶" ("工步描述") "请对锁紧螺母加力" ("工步描述") "灵敏度测试中" ("工步描述") "有油刚度测试中" ("工步描述") "安装好锁紧螺母后，按顶升按钮，夹具夹紧" ("工步描述") "请点击启动按钮进行试验" ("工步描述") "探头气缸右移" ("工步描述") "电动缸前进找中" ("工步描述") "探头前进测试开始" ("工步描述") "探头退回" ("工步描述") "轴向力测试中" ("工步描述") "测头后退夹抓松开" ("工步描述") "伺服回零" ("工步描述") "力特性试验完成" ("工步描述") "套好输出轴把手，按启动按钮，做回正力试验" ("工步描述") "回正力试验中" ("工步描述") "试验完成，将把手拉回，取下油管，按顶升按钮" ("工步描述") "拆下锁紧螺母和输入轴万向节，按顶升按钮" ("工步描述")] -> w1469
          frame 0, Default {
            n918 = local read "联线按钮"() -> (w1479:bool)
            n919 = case shown="真" w1479 {
              tunnel: ["等待工件" ("工步描述") "等待扫描条码" ("工步描述")] -> w1480
              frame False {
              }
              frame True {
              }
            }
          }
          frame 1 {
          }
          frame 2 {
          }
          frame 3 {
          }
          frame 4 {
          }
          frame 5 {
          }
          frame 6 {
          }
          frame 10 {
          }
          frame 15 {
          }
          frame 20 {
          }
          frame 30 {
          }
          frame 40 {
          }
          frame 45 {
          }
          frame 50 {
          }
          frame 55 {
          }
          frame 60 {
          }
          frame 70 {
          }
          frame 80 {
          }
          frame 56 {
          }
        }
        "工步提示" <- w1469
        n920 = case shown="3" w1468 {
          tunnel: [_ "操作步骤错请取胶瓶" "操作步骤错误请点标" "测头气缸不在原位" "急停被按下" "气压报警" "电动缸伺服报警" "旋转伺服服报警" "测头伺服服报警"] -> w1467
          frame 0, Default {
          }
          frame 1 {
          }
          frame 3 {
          }
          frame 2 {
          }
          frame 4 {
          }
          frame 5 {
          }
          frame 6 {
          }
          frame 7 {
          }
          frame 8 {
          }
        }
        "报警提示" <- w1467
      }
      frame #4 {
        n921 = local read "急停"() -> (w1502:bool)
        n922 = local read "红灯"() -> (w1501:bool)
        n923 = local read "复位"() -> (w1504:bool)
        n924 = local read "红灯"() -> (w1503:bool)
        n925 = case shown="假" w1502 {
          frame False {
            n926 = local write "红灯"(TRUE ("红灯")) -> ()
          }
          frame True {
            n927 = local write "红灯"(FALSE ("复位")) -> ()
          }
        }
        n928 = case shown="真" w1501 {
          frame False {
          }
          frame True {
            n929 = local write "回零完成"(FALSE ("夹头夹紧控制")) -> ()
          }
        }
        n930 = local read "停止"() -> (w1506:bool)
        n931 = Compound Arithmetic op=OR(w1504, w1506, w1503) -> (w1505:bool)
        n932 = case shown="真" w1505 {
          frame False {
          }
          frame True {
            n933 = local read "测头机构电机"() -> (w1510:u32)
            n934 = local read "旋转齿条电机"() -> (w1511:u32)
            n935 = local read "电动缸电机"() -> (w1512:u32)
            n936 = call "PCI1220U停止.vi"("AxisHandle IN"=w1511) -> ()  [unwired: 9 in, 2 out]
            n937 = call "PCI1220U停止.vi"("AxisHandle IN"=w1512) -> ()  [unwired: 9 in, 2 out]
            n938 = call "PCI1220U停止.vi"("AxisHandle IN"=w1510) -> ()  [unwired: 9 in, 2 out]
          }
        }
      }
      frame #5 {
        n939 = local read "齿条扭矩(Nm)"() -> (w1515:dbl)
        n940 = local read "黄灯"() -> (w1513:bool)
        n941 = local read "旋转齿条轴左转"() -> (w1521:bool)
        n942 = Absolute Value(x=w1515) -> (abs(x)=w1520:dbl)
        n943 = local read "旋转齿条轴右转"() -> (w1516:bool)
        n944 = Not(x=w1521) -> (.not. x?=w1517:bool)
        n945 = Less?(x=w1520, y=20.0) -> (x < y?=w1518:bool)
        n946 = Compound Arithmetic op=AND(w1516, w1517, w1518, w1513) -> (w1514:bool)
        n947 = case shown="真" w1514 {
          frame False {
          }
          frame True {
            n948 = flat-sequence {
              tunnel: [w1525] -> w1523
              tunnel: w1523 -> [w1527]
              tunnel: [w1527] -> w1522
              tunnel: w1522 -> [w1538]
              frame #0 {
                n949 = local read "旋转齿条电机"() -> (w1524:u32)
                n950 = call "PCI1220U运行.vi"("方向"=enum32{"Negative", "Positive"}."Negative" ("Direction"), "AxisHandle IN"=w1524) -> ("AxisHandle OUT"=w1525:u32)  [unwired: 9 in]
              }
              frame #1 {
                n951 = while {
                  stop <- w1531 stop-if-true
                  n952 = Wait (ms)(milliseconds to wait=u32 50 ("毫秒倍数")) -> ()  [unwired: 1 out]
                  n953 = local read "齿条扭矩(Nm)"() -> (w1536:dbl)
                  n954 = local read "旋转齿条轴右转"() -> (w1533:bool)
                  n955 = local read "红灯"() -> (w1528:bool)
                  n956 = local read "复位"() -> (w1529:bool)
                  n957 = Absolute Value(x=w1536) -> (abs(x)=w1535:dbl)
                  n958 = Not(x=w1533) -> (.not. x?=w1530:bool)
                  n959 = Greater?(x=w1535, y=10.0) -> (0:w1532:bool)
                  n960 = Compound Arithmetic op=OR(w1532, w1530, w1529, w1528) -> (w1531:bool)
                }
              }
              frame #2 {
                n961 = call "PCI1220U停止.vi"("AxisHandle IN"=w1538) -> ()  [unwired: 9 in, 2 out]
              }
            }
          }
        }
      }
      frame #6 {
        n962 = local read "齿条扭矩(Nm)"() -> (w1543:dbl)
        n963 = local read "旋转齿条轴右转"() -> (w1547:bool)
        n964 = Absolute Value(x=w1543) -> (abs(x)=w1542:dbl)
        n965 = local read "旋转齿条轴左转"() -> (w1545:bool)
        n966 = local read "黄灯"() -> (w1539:bool)
        n967 = Not(x=w1547) -> (.not. x?=w1544:bool)
        n968 = Less?(x=w1542, y=20.0) -> (x < y?=w1540:bool)
        n969 = Compound Arithmetic op=AND(w1545, w1544, w1540, w1539) -> (w1546:bool)
        n970 = case shown="真" w1546 {
          frame False {
          }
          frame True {
            n971 = flat-sequence {
              tunnel: [w1551] -> w1549
              tunnel: w1549 -> [w1553]
              tunnel: [w1553] -> w1548
              tunnel: w1548 -> [w1564]
              frame #0 {
                n972 = local read "旋转齿条电机"() -> (w1550:u32)
                n973 = call "PCI1220U运行.vi"("方向"=enum32{"Negative", "Positive"}."Positive" ("Direction"), "AxisHandle IN"=w1550) -> ("AxisHandle OUT"=w1551:u32)  [unwired: 9 in]
              }
              frame #1 {
                n974 = while {
                  stop <- w1556 stop-if-true
                  n975 = Wait (ms)(milliseconds to wait=u32 50 ("毫秒倍数")) -> ()  [unwired: 1 out]
                  n976 = local read "齿条扭矩(Nm)"() -> (w1562:dbl)
                  n977 = local read "旋转齿条轴左转"() -> (w1559:bool)
                  n978 = local read "红灯"() -> (w1554:bool)
                  n979 = local read "复位"() -> (w1555:bool)
                  n980 = Absolute Value(x=w1562) -> (abs(x)=w1561:dbl)
                  n981 = Not(x=w1559) -> (.not. x?=w1557:bool)
                  n982 = Greater?(x=w1561, y=10.0) -> (0:w1558:bool)
                  n983 = Compound Arithmetic op=OR(w1555, w1554, w1558, w1557) -> (w1556:bool)
                }
              }
              frame #2 {
                n984 = call "PCI1220U停止.vi"("AxisHandle IN"=w1564) -> ()  [unwired: 9 in, 2 out]
              }
            }
          }
        }
      }
      frame #7 {
        n985 = local read "齿条推拉力(N)"() -> (w1569:dbl)
        n986 = local read "电动缸前进"() -> (w1566:bool)
        n987 = local read "电动缸后退"() -> (w1565:bool)
        n988 = Absolute Value(x=w1569) -> (abs(x)=w1573:dbl)
        n989 = local read "黄灯"() -> (w1567:bool)
        n990 = Not(x=w1565) -> (.not. x?=w1570:bool)
        n991 = Less?(x=w1573, y=1000.0) -> (x < y?=w1571:bool)
        n992 = Compound Arithmetic op=AND(w1566, w1570, w1567, w1571) -> (w1568:bool)
        n993 = case shown="真" w1568 {
          frame False {
          }
          frame True {
            n994 = flat-sequence {
              tunnel: [w1577] -> w1575
              tunnel: w1575 -> [w1579]
              tunnel: [w1579] -> w1574
              tunnel: w1574 -> [w1590]
              frame #0 {
                n995 = local read "电动缸电机"() -> (w1576:u32)
                n996 = call "PCI1220U运行.vi"("方向"=enum32{"Negative", "Positive"}."Positive" ("Direction"), "AxisHandle IN"=w1576) -> ("AxisHandle OUT"=w1577:u32)  [unwired: 9 in]
              }
              frame #1 {
                n997 = while {
                  stop <- w1587 stop-if-true
                  n998 = local read "电动缸前进"() -> (w1584:bool)
                  n999 = local read "齿条推拉力(N)"() -> (w1581:dbl)
                  n1000 = Wait (ms)(milliseconds to wait=u32 50 ("毫秒倍数")) -> ()  [unwired: 1 out]
                  n1001 = Absolute Value(x=w1581) -> (abs(x)=w1583:dbl)
                  n1002 = local read "红灯"() -> (w1585:bool)
                  n1003 = local read "复位"() -> (w1586:bool)
                  n1004 = Greater?(x=w1583, y=1000.0) -> (0:w1580:bool)
                  n1005 = Not(x=w1584) -> (.not. x?=w1588:bool)
                  n1006 = Compound Arithmetic op=OR(w1586, w1585, w1588, w1580) -> (w1587:bool)
                }
              }
              frame #2 {
                n1007 = call "PCI1220U停止.vi"("AxisHandle IN"=w1590) -> ()  [unwired: 9 in, 2 out]
              }
            }
          }
        }
      }
      frame #8 {
        n1008 = local read "电动缸前进"() -> (w1591:bool)
        n1009 = local read "齿条推拉力(N)"() -> (w1595:dbl)
        n1010 = local read "电动缸后退"() -> (w1592:bool)
        n1011 = Absolute Value(x=w1595) -> (abs(x)=w1599:dbl)
        n1012 = local read "黄灯"() -> (w1593:bool)
        n1013 = Not(x=w1591) -> (.not. x?=w1596:bool)
        n1014 = Less?(x=w1599, y=1000.0) -> (x < y?=w1597:bool)
        n1015 = Compound Arithmetic op=AND(w1592, w1596, w1593, w1597) -> (w1594:bool)
        n1016 = case shown="真" w1594 {
          frame False {
          }
          frame True {
            n1017 = flat-sequence {
              tunnel: [w1603] -> w1601
              tunnel: w1601 -> [w1605]
              tunnel: [w1605] -> w1600
              tunnel: w1600 -> [w1616]
              frame #0 {
                n1018 = local read "电动缸电机"() -> (w1602:u32)
                n1019 = call "PCI1220U运行.vi"("方向"=enum32{"Negative", "Positive"}."Negative" ("Direction"), "AxisHandle IN"=w1602) -> ("AxisHandle OUT"=w1603:u32)  [unwired: 9 in]
              }
              frame #1 {
                n1020 = while {
                  stop <- w1613 stop-if-true
                  n1021 = local read "电动缸后退"() -> (w1610:bool)
                  n1022 = local read "齿条推拉力(N)"() -> (w1609:dbl)
                  n1023 = Wait (ms)(milliseconds to wait=u32 50 ("毫秒倍数")) -> ()  [unwired: 1 out]
                  n1024 = Absolute Value(x=w1609) -> (abs(x)=w1607:dbl)
                  n1025 = local read "红灯"() -> (w1612:bool)
                  n1026 = local read "复位"() -> (w1611:bool)
                  n1027 = Greater?(x=w1607, y=1000.0) -> (0:w1606:bool)
                  n1028 = Not(x=w1610) -> (.not. x?=w1614:bool)
                  n1029 = Compound Arithmetic op=OR(w1611, w1612, w1614, w1606) -> (w1613:bool)
                }
              }
              frame #2 {
                n1030 = call "PCI1220U停止.vi"("AxisHandle IN"=w1616) -> ()  [unwired: 9 in, 2 out]
              }
            }
          }
        }
      }
      frame #9 {
        n1031 = local read "测头机构轴后退"() -> (w1617:bool)
        n1032 = local read "测头机构轴前进"() -> (w1618:bool)
        n1033 = local read "黄灯"() -> (w1619:bool)
        n1034 = Not(x=w1617) -> (.not. x?=w1621:bool)
        n1035 = Compound Arithmetic op=AND(w1618, w1621, w1619) -> (w1620:bool)
        n1036 = case shown="真" w1620 {
          frame False {
          }
          frame True {
            n1037 = flat-sequence {
              tunnel: [w1625] -> w1623
              tunnel: w1623 -> [w1627]
              tunnel: [w1627] -> w1622
              tunnel: w1622 -> [w1634]
              frame #0 {
                n1038 = local read "测头机构电机"() -> (w1624:u32)
                n1039 = call "PCI1220U运行.vi"("方向"=enum32{"Negative", "Positive"}."Positive" ("Direction"), "AxisHandle IN"=w1624) -> ("AxisHandle OUT"=w1625:u32)  [unwired: 9 in]
              }
              frame #1 {
                n1040 = while {
                  stop <- w1631 stop-if-true
                  n1041 = local read "测头机构轴前进"() -> (w1628:bool)
                  n1042 = Wait (ms)(milliseconds to wait=u32 50 ("毫秒倍数")) -> ()  [unwired: 1 out]
                  n1043 = local read "红灯"() -> (w1629:bool)
                  n1044 = local read "复位"() -> (w1630:bool)
                  n1045 = Not(x=w1628) -> (.not. x?=w1632:bool)
                  n1046 = Compound Arithmetic op=OR(w1630, w1629, w1632) -> (w1631:bool)
                }
              }
              frame #2 {
                n1047 = call "PCI1220U停止.vi"("AxisHandle IN"=w1634) -> ()  [unwired: 9 in, 2 out]
              }
            }
          }
        }
      }
      frame #10 {
        n1048 = local read "测头机构轴前进"() -> (w1635:bool)
        n1049 = local read "测头机构轴后退"() -> (w1636:bool)
        n1050 = local read "黄灯"() -> (w1637:bool)
        n1051 = Not(x=w1635) -> (.not. x?=w1639:bool)
        n1052 = Compound Arithmetic op=AND(w1636, w1639, w1637) -> (w1638:bool)
        n1053 = case shown="真" w1638 {
          frame False {
          }
          frame True {
            n1054 = flat-sequence {
              tunnel: [w1643] -> w1641
              tunnel: w1641 -> [w1645]
              tunnel: [w1645] -> w1640
              tunnel: w1640 -> [w1652]
              frame #0 {
                n1055 = local read "测头机构电机"() -> (w1642:u32)
                n1056 = call "PCI1220U运行.vi"("方向"=enum32{"Negative", "Positive"}."Negative" ("Direction"), "AxisHandle IN"=w1642) -> ("AxisHandle OUT"=w1643:u32)  [unwired: 9 in]
              }
              frame #1 {
                n1057 = while {
                  stop <- w1649 stop-if-true
                  n1058 = local read "测头机构轴后退"() -> (w1646:bool)
                  n1059 = Wait (ms)(milliseconds to wait=u32 50 ("毫秒倍数")) -> ()  [unwired: 1 out]
                  n1060 = local read "红灯"() -> (w1648:bool)
                  n1061 = local read "复位"() -> (w1647:bool)
                  n1062 = Not(x=w1646) -> (.not. x?=w1650:bool)
                  n1063 = Compound Arithmetic op=OR(w1647, w1648, w1650) -> (w1649:bool)
                }
              }
              frame #2 {
                n1064 = call "PCI1220U停止.vi"("AxisHandle IN"=w1652) -> ()  [unwired: 9 in, 2 out]
              }
            }
          }
        }
      }
      frame #11 {
        n1065 = local read "电动缸回零"() -> (w1653:bool)
        n1066 = case shown="真" w1653 {
          frame False {
          }
          frame True {
            n1067 = stacked-sequence {
              frame #0 {
                n1068 = flat-sequence {
                  tunnel: [w1669] -> w1659
                  tunnel: [w1662] -> w1658
                  tunnel: w1659 -> [w1672]
                  tunnel: [w1672] -> w1657
                  tunnel: [w1670] -> w1656
                  tunnel: w1658 -> [w1670]
                  tunnel: w1657 -> [w1674]
                  tunnel: [w1674] -> w1655
                  tunnel: w1656 -> [w1673]
                  tunnel: [w1673] -> w1654
                  tunnel: w1655 -> [w1690]
                  tunnel: w1654 -> [w1689]
                  frame #0 {
                    n1069 = local write "电动缸速度(mm/s)"(15.0 ("电动缸速度(mm/s)")) -> ()
                    n1070 = local write "测头机构轴速度(mm/s)"(10.0 ("电动缸速度(mm/s)")) -> ()
                  }
                  frame #1 {
                    n1071 = local read "测头机构电机"() -> (w1666:u32)
                    n1072 = local read "电动缸电机"() -> (w1663:u32)
                    n1073 = call <userlib>:"Acm_AxHome.vi"("DirMode"=u32 1, "HomeMode"=u32 11, "AxisHandle"=w1663) -> ("AxisHandle"=w1662:u32)  [unwired: 1 in, 2 out]
                    n1074 = call <userlib>:"Acm_AxHome.vi"("DirMode"=u32 0, "HomeMode"=u32 11, "AxisHandle"=w1666) -> ("AxisHandle"=w1669:u32)  [unwired: 1 in, 2 out]
                  }
                  frame #2 {
                    n1075 = Wait Until Next ms Multiple(millisecond multiple=u32 100 ("毫秒倍数")) -> ()  [unwired: 1 out]
                  }
                  frame #3 {
                    n1076 = while {
                      tunnel: w1673 -> [w1681]
                      stop <- w1676 stop-if-true
                      n1077 = call <userlib>:"Acm_AxGetCmdVelocity.vi"("AxisHandle"=w1681) -> ("Velocity"=w1680:dbl)  [unwired: 1 in, 3 out]
                      n1078 = Wait Until Next ms Multiple(millisecond multiple=u32 50 ("毫秒倍数")) -> ()  [unwired: 1 out]
                      n1079 = Equal To 0?(x=w1680) -> (x = 0?=w1675:bool)
                      n1080 = local read "急停"() -> (w1677:bool)
                      n1081 = local read "复位"() -> (w1678:bool)
                      n1082 = Compound Arithmetic op=OR(invert w1677, w1678, w1675) -> (w1676:bool)
                    }
                    n1083 = while {
                      tunnel: w1674 -> [w1688]
                      stop <- w1684 stop-if-true
                      n1084 = call <userlib>:"Acm_AxGetCmdVelocity.vi"("AxisHandle"=w1688) -> ("Velocity"=w1687:dbl)  [unwired: 1 in, 3 out]
                      n1085 = Wait Until Next ms Multiple(millisecond multiple=u32 50 ("毫秒倍数")) -> ()  [unwired: 1 out]
                      n1086 = Equal To 0?(x=w1687) -> (x = 0?=w1685:bool)
                      n1087 = local read "急停"() -> (w1682:bool)
                      n1088 = local read "复位"() -> (w1683:bool)
                      n1089 = Compound Arithmetic op=OR(invert w1682, w1683, w1685) -> (w1684:bool)
                    }
                  }
                  frame #4 {
                    n1090 = call "PCI1220U角度置零.vi"("AxisHandle IN"=w1689) -> ()  [unwired: 10 in, 1 out]
                    n1091 = call "PCI1220U角度置零.vi"("AxisHandle IN"=w1690) -> ()  [unwired: 10 in, 1 out]
                  }
                }
              }
              frame #1 {
                n1092 = flat-sequence {
                  tunnel: [w1702] -> w1697
                  tunnel: w1697 -> [w1704]
                  tunnel: [w1704] -> w1696
                  tunnel: w1696 -> [w1705]
                  tunnel: [w1705] -> w1695
                  tunnel: w1695 -> [w1714]
                  tunnel: [w1713] -> w1692
                  tunnel: w1692 -> [w1716]
                  tunnel: [w1716] -> w1691
                  tunnel: w1691 -> [w1718]
                  tunnel: [w1717] -> w1694
                  tunnel: w1694 -> [w1727]
                  tunnel: [w1727] -> w1693
                  tunnel: w1693 -> [w1735]
                  frame #0 {
                    n1093 = local write "旋转齿条轴速度(°/s)"(5.0 ("电动缸速度(mm/s)")) -> ()
                  }
                  frame #1 {
                    n1094 = local read "旋转齿条电机"() -> (w1699:u32)
                    n1095 = call <userlib>:"Acm_AxHome.vi"("DirMode"=u32 0, "HomeMode"=u32 11, "AxisHandle"=w1699) -> ("AxisHandle"=w1702:u32)  [unwired: 1 in, 2 out]
                  }
                  frame #2 {
                    n1096 = Wait Until Next ms Multiple(millisecond multiple=u32 100 ("毫秒倍数")) -> ()  [unwired: 1 out]
                  }
                  frame #3 {
                    n1097 = while {
                      tunnel: w1705 -> [w1712]
                      stop <- w1706 stop-if-true
                      n1098 = call <userlib>:"Acm_AxGetCmdVelocity.vi"("AxisHandle"=w1712) -> ("Velocity"=w1711:dbl)  [unwired: 1 in, 3 out]
                      n1099 = Wait Until Next ms Multiple(millisecond multiple=u32 50 ("毫秒倍数")) -> ()  [unwired: 1 out]
                      n1100 = Equal To 0?(x=w1711) -> (x = 0?=w1707:bool)
                      n1101 = local read "急停"() -> (w1709:bool)
                      n1102 = local read "复位"() -> (w1708:bool)
                      n1103 = Compound Arithmetic op=OR(invert w1709, w1708, w1707) -> (w1706:bool)
                    }
                  }
                  frame #4 {
                    n1104 = call "PCI1220U角度置零.vi"("AxisHandle IN"=w1714) -> ("AxisHandle OUT"=w1713:u32)  [unwired: 10 in]
                  }
                  frame #5 {
                    n1105 = Wait (ms)(milliseconds to wait=u32 100 ("等待时间（毫秒）")) -> ()  [unwired: 1 out]
                  }
                  frame #6 {
                    n1106 = while {
                      tunnel: [w1725] -> w1717
                      tunnel: w1718 -> [w1723]
                      stop <- w1720 stop-if-true
                      n1107 = call "PCI1220U扭矩轴位置模式.vi"("Distance"=10.0, "AxisHandle IN"=w1723) -> ("AbsSuccess"=w1719:bool, "AxisHandle OUT"=w1725:u32)  [unwired: 8 in]
                      n1108 = Wait Until Next ms Multiple(millisecond multiple=u32 50 ("毫秒倍数")) -> ()  [unwired: 1 out]
                      n1109 = local read "急停"() -> (w1722:bool)
                      n1110 = local read "复位"() -> (w1721:bool)
                      n1111 = Compound Arithmetic op=OR(invert w1722, w1721, w1719) -> (w1720:bool)
                    }
                  }
                  frame #7 {
                    n1112 = while {
                      tunnel: w1727 -> [w1733]
                      stop <- w1728 stop-if-true
                      n1113 = call <userlib>:"Acm_AxGetCmdVelocity.vi"("AxisHandle"=w1733) -> ("Velocity"=w1734:dbl)  [unwired: 1 in, 3 out]
                      n1114 = Wait Until Next ms Multiple(millisecond multiple=u32 50 ("毫秒倍数")) -> ()  [unwired: 1 out]
                      n1115 = Equal To 0?(x=w1734) -> (x = 0?=w1729:bool)
                      n1116 = local read "急停"() -> (w1731:bool)
                      n1117 = local read "复位"() -> (w1730:bool)
                      n1118 = Compound Arithmetic op=OR(w1729, invert w1731, w1730) -> (w1728:bool)
                    }
                  }
                  frame #8 {
                    n1119 = call "PCI1220U角度置零.vi"("AxisHandle IN"=w1735) -> ()  [unwired: 10 in, 1 out]
                  }
                }
              }
              frame #2 {
                n1120 = flat-sequence {
                  frame #0 {
                    n1121 = while {
                      stop <- w1736 stop-if-true
                      n1122 = local read "电动缸回零"() -> (w1743:bool)
                      n1123 = local write "回零完成"(TRUE ("回零完成")) -> ()
                      n1124 = local write "电动缸回零"(FALSE ("电动缸回零")) -> ()
                      n1125 = Wait Until Next ms Multiple(millisecond multiple=u32 50 ("毫秒倍数")) -> ()  [unwired: 1 out]
                      n1126 = Not(x=w1743) -> (.not. x?=w1737:bool)
                      n1127 = local read "急停"() -> (w1738:bool)
                      n1128 = local read "复位"() -> (w1739:bool)
                      n1129 = Compound Arithmetic op=OR(w1737, invert w1738, w1739) -> (w1736:bool)
                    }
                  }
                }
              }
            }
          }
        }
      }
    }
    n1130 = Wait (ms)(milliseconds to wait=u32 50 ("毫秒倍数")) -> ()  [unwired: 1 out]
    n1131 = local read "停止"() -> (w1439:bool)
  }
  n1132 = while {
    stop <- FALSE stop-if-true
    n1133 = Equal?(x="密码", y="jizhuan") -> (x = y?=w1747:bool)
    n1134 = Compound Arithmetic op=AND(w1747, "?") -> (w1745:bool)
    n1135 = case shown="假" w1745 {
      frame False {
        n1136 = property class="Bool (严格)"("DisabledEnum"=T5."Disabled and Grayed Out" ("禁用")) -> ()  [unwired: 2 in, 2 out]
        n1137 = property class="Bool (严格)"("DisabledEnum"=T5."Disabled and Grayed Out" ("禁用")) -> ()  [unwired: 2 in, 2 out]
      }
      frame True {
        n1138 = property class="Bool (严格)"("DisabledEnum"=T5."Enabled" ("禁用")) -> ()  [unwired: 2 in, 2 out]
        n1139 = property class="Bool (严格)"("DisabledEnum"=T5."Enabled" ("禁用")) -> ()  [unwired: 2 in, 2 out]
        n1140 = case shown="真" "?" {
          frame False {
          }
          frame True {
            n1141 = property on="选项卡控件" class="TabCtl (严格)"() -> ("Pages"=w1756:refnum<vi>[])  [unwired: 2 in, 2 out]
            n1142 = for {
              N: 7 -> [_]
              tunnel: w1756 -> [w1758] mode=indexing
              i -> [w1759]
              n1143 = case shown="5" w1759 {
                tunnel: w1758 -> [_ w1761]
                frame 0, Default {
                }
                frame 5 {
                  n1144 = property class="Page"(reference=w1761, "PageVis"=FALSE ("选项卡可见")) -> ()  [unwired: 1 in, 2 out]
                }
              }
            }
          }
        }
        n1145 = case shown="真" "?" {
          frame False {
          }
          frame True {
            n1146 = property on="选项卡控件" class="TabCtl (严格)"() -> ("Pages"=w1762:refnum<vi>[])  [unwired: 2 in, 2 out]
            n1147 = for {
              N: 7 -> [_]
              tunnel: w1762 -> [w1764] mode=indexing
              i -> [w1765]
              n1148 = case shown="5" w1765 {
                tunnel: w1764 -> [_ w1767]
                frame 0, Default {
                }
                frame 5 {
                  n1149 = property class="Page"(reference=w1767, "PageVis"=TRUE ("选项卡可见")) -> ()  [unwired: 1 in, 2 out]
                }
              }
            }
          }
        }
      }
    }
  }
  n1150 = flat-sequence {
    tunnel: [w1771] -> w2
    tunnel: [w1769] -> w1
    tunnel: w2 -> [w1781]
    tunnel: w1 -> [w1780]
    frame #0 {
      n1151 = First Call?() -> (First Call?: T/F=w1768:bool)
      n1152 = case shown="真" w1768 {
        frame False {
        }
        frame True {
          n1153 = while {
            i -> [w1776]
            stop <- w1774 stop-if-true
            w1779 = TRUE ("电动缸使能")
            n1154 = local write "回零完成"(FALSE ("回零完成")) -> ()
            n1155 = local write "测头机构轴使能"(w1779) -> ()
            n1156 = local write "旋转齿条轴使能"(w1779) -> ()
            n1157 = local write "电动缸使能"(w1779) -> ()
            n1158 = Wait Until Next ms Multiple(millisecond multiple=u32 50 ("毫秒倍数")) -> ()  [unwired: 1 out]
            n1159 = Greater Or Equal?(x=w1776, y=30) -> (x >= y?=w1774:bool)
          }
        }
      }
      n1160 = call "ADO Connection Create.vi"() -> ("error out"=w1772:errorcluster, "ADODB._Connection Out"=w1773:refnum<k7>)  [unwired: 10 in]
      n1161 = call "ADO Connection Open.vi"("error in (no error)"=w1772, "ConnectionString"="Provider=Microsoft.Jet.OLEDB.4.0;Data Source=D:\\Q14070-Z060人机界面\\参数\\参数Z060.mdb;Persist Security Info=False;Jet OLEDB:Database Password=1234;", "ADODB._Connection In"=w1773) -> ("error out"=w1769:errorcluster, "ADODB._Connection Out"=w1771:refnum<k7>)  [unwired: 7 in]
    }
    frame #1 {
      n1162 = while {
        tunnel: w1781 -> [w1783]
        tunnel: w1780 -> [w1782]
        stop <- w1787 stop-if-true
        n1163 = Wait (ms)(milliseconds to wait=u32 50 ("等待时间（毫秒）")) -> ()  [unwired: 1 out]
        n1164 = First Call?() -> (First Call?: T/F=w1786:bool)
        n1165 = Or(x=w1786, y="参数加载") -> (x .or. y?=w1785:bool)
        n1166 = case shown="真" w1785 {
          tunnel: w1783 -> [_ w1790]
          tunnel: w1782 -> [_ w1789]
          frame False {
          }
          frame True {
            n1167 = stacked-sequence {
              tunnel: w1790 -> [w1796 w1807 w1870]
              tunnel: w1789 -> [w1791 _ _]
              frame #0 {
                n1168 = call "SQL Execute.vi"("error in (no error)"=w1791, "Command Text"="SELECT * FROM 测试参数表", "ADODB._Connection In"=w1796) -> ("Data"=w1794:string[][])  [unwired: 5 in, 3 out]
                n1169 = Index Array(array=w1794, index (col)=0 ("索引 (行)")) -> (element=w1798:string[])  [unwired: 1 in]
                n1170 = Array Size(array=w1798) -> (size(s)=w1793:i32)
                "型号数量" <- w1793
                n1171 = while {
                  shift-right: [w1805] -> w1797
                  shift-left: i32[] [] -> [w1804]
                  tunnel: w1793 -> [w1802]
                  i -> [w1803]
                  stop <- w1801 stop-if-true
                  n1172 = Greater Or Equal?(x=w1803, y=w1802) -> (x >= y?=w1801:bool)
                  n1173 = Build Array (concatenate)(w1804, w1803) -> (w1805:i32[])
                }
                n1174 = Build Cluster Array "索引与捆绑簇数组"(w1798, w1797) -> (w1792:cluster{"String":string, i32}[])
                n1175 = property on="型号选择" class="Ring (严格)"("StringsAndValues[]"=w1792) -> ()  [unwired: 2 in, 2 out]
              }
              frame #1 {
                n1176 = property on="型号选择" class="Ring (严格)"() -> ("RingText.Text"=w1808:string)  [unwired: 2 in, 2 out]
                n1177 = call "创建文本2"("型号选择"=w1808) -> ("Result"=w1812:string)  [unwired: 13 in, 1 out]
                n1178 = call "SQL Execute.vi"("Command Text"=w1812, "ADODB._Connection In"=w1807) -> ("Data"=w1811:string[][])  [unwired: 6 in, 3 out]
                n1179 = Index Array(array=w1811, index (row)=0 ("索引 (行)")) -> (element=w1809:string[])  [unwired: 1 in]
                n1180 = Fract/Exp String To Number ("分数/指数字符串至数值转换")(string=w1809) -> (number=w1806:dbl[])  [unwired: 3 in, 1 out]
                n1181 = stacked-sequence {
                  tunnel: w1806 -> [w1846]
                  frame #0 {
                    n1182 = Index Array ("索引数组")(array=w1846, index #1=2 ("索引"), index #2=3 ("索引"), index #3=4 ("索引"), index #4=5 ("索引"), index #5=6 ("索引"), index #6=7 ("索引"), index #7=8 ("索引"), index #8=9 ("索引"), index #9=10 ("索引"), index #10=11 ("索引"), index #11=12 ("索引"), index #12=13 ("索引"), index #13=14 ("索引"), index #14=15 ("索引"), index #15=16 ("索引"), index #16=17 ("索引"), index #17=18 ("索引"), index #18=19 ("索引"), index #19=20 ("索引"), index #20=21 ("索引"), index #21=22 ("索引"), index #22=23 ("索引")) -> (element #1=w1845:dbl, element #2=w1844:dbl, element #3=w1843:dbl, element #4=w1842:dbl, element #5=w1841:dbl, element #6=w1840:dbl, element #7=w1839:dbl, element #8=w1838:dbl, element #9=w1837:dbl, element #10=w1836:dbl, element #11=w1829:dbl, element #12=w1828:dbl, element #13=→"齿条传动比":dbl, element #14=→"力波动标准(N)":dbl, element #15=→"轴向力标准(N)":dbl, element #16=→"平均轴向力标准(N) max":dbl, element #17=→"总圈数标准":dbl, element #18=→"总圈数最大值":dbl, element #20=w1818:dbl, element #21=w1817:dbl, element #22=w1816:dbl)  [unwired: 1 out]
                    n1183 = local write "测头机构轴移动速度"(w1845) -> ()
                    n1184 = local write "中间位置最大间隙标准(mm)"(w1818) -> ()
                    n1185 = local write "测头机构轴检测位"(w1844) -> ()
                    n1186 = local write "测头机构轴后退位"(w1842) -> ()
                    n1187 = local write "180°外全行程间隙标准(mm)"(w1816) -> ()
                    n1188 = local write "测头机构轴待检位"(w1843) -> ()
                    n1189 = local write "180°内全行程间隙标准(mm)"(w1817) -> ()
                    n1190 = local write "旋转齿条轴找帽转速"(w1838) -> ()
                    n1191 = local write "旋转齿条轴测量转速"(w1837) -> ()
                    n1192 = local write "总行程标准(mm)"(w1829) -> ()
                    n1193 = local write "齿条移动速度"(w1841) -> ()
                    n1194 = local write "齿条左极限"(w1840) -> ()
                    n1195 = local write "齿条右极限"(w1839) -> ()
                    n1196 = local write "总行程最大值"(w1828) -> ()
                    n1197 = local write "测量点扭矩"(w1836) -> ()
                  }
                }
              }
              frame #2 {
                n1198 = call "SQL Execute.vi"("Command Text"="SELECT * FROM 传感器校验表 where ID='1'", "ADODB._Connection In"=w1870) -> ("Data"=w1872:string[][])  [unwired: 6 in, 3 out]
                n1199 = Index Array(array=w1872) -> (element=w1873:string[])  [unwired: 2 in]
                n1200 = Fract/Exp String To Number ("分数/指数字符串至数值转换")(string=w1873) -> (number=w1863:dbl[])  [unwired: 3 in, 1 out]
                n1201 = Index Array(array=w1863, index #1=1 ("索引"), index #2=2 ("索引"), index #3=3 ("索引"), index #4=4 ("索引"), index #5=5 ("索引"), index #6=6 ("索引")) -> (element #1=w1862:dbl, element #2=w1861:dbl, element #3=w1860:dbl, element #4=w1859:dbl, element #5=w1858:dbl, element #6=w1857:dbl)
                n1202 = local write "间隙位移零点偏移"(w1862) -> ()
                n1203 = local write "间隙位移比例偏移"(w1861) -> ()
                n1204 = local write "齿条推拉力零点偏移"(w1860) -> ()
                n1205 = local write "齿条推拉力比例偏移"(w1859) -> ()
                n1206 = local write "齿条扭矩零点偏移"(w1858) -> ()
                n1207 = local write "齿条扭矩比例偏移"(w1857) -> ()
              }
            }
          }
        }
        n1208 = local read "停止"() -> (w1787:bool)
        "ADODB._Connection Out 2" <- w1783
      }
    }
  }
  n1209 = while {
    stop <- w1875 stop-if-true
    n1210 = local read "rfid工步号"() -> (w1874:u32)
    n1211 = case shown="10" w1874 {
      frame 0, Default {
      }
      frame 10 {
        n1212 = flat-sequence {
          tunnel: [w1885] -> w1879
          tunnel: w1879 -> [w1887]
          tunnel: [w1886] -> w1878
          tunnel: w1878 -> [w1889]
          tunnel: [w1889] -> w1877
          tunnel: w1877 -> [w1892]
          frame #0 {
            n1213 = while {
              stop <- w1880 stop-if-true
              n1214 = local read "rfid触发"() -> (w1880:bool)
              n1215 = Wait Until Next ms Multiple(millisecond multiple=u32 50 ("毫秒倍数")) -> ()  [unwired: 1 out]
            }
          }
          frame #1 {
            n1216 = local write "芯片ID"("" ("随行板ID")) -> ()
            n1217 = local write "rfid完成"(FALSE ("RFID完成")) -> ()
            n1218 = local write "rfid触发"(FALSE ("RFID读取触发")) -> ()
          }
          frame #2 {
            n1219 = local read "Z060BRFID"() -> (w1885:string)
            n1220 = local write "芯片ID"(w1885) -> ()
          }
          frame #3 {
            n1221 = call "查询产品ID.vi"("芯片编码"=w1887) -> ("产品ID"=w1886:string)  [unwired: 8 in, 2 out]
            "读取产品ID" <- w1886
          }
          frame #4 {
            n1222 = Wait (ms)(milliseconds to wait=u32 500 ("等待时间（毫秒）")) -> ()  [unwired: 1 out]
          }
          frame #5 {
            n1223 = call "查询上序合格.vi"("产品ID"=w1892) -> ("本序已做"=w1890:bool, "上序合格"=w1891:bool)  [unwired: 8 in, 1 out]
            n1224 = Not(x=w1891) -> (.not. x?=w1893:bool)
            n1225 = local write "上序合格"(w1891) -> ()
            n1226 = local write "本序已做"(w1890) -> ()
            n1227 = local write "上序不合格"(w1893) -> ()
          }
          frame #6 {
            n1228 = local write "rfid完成"(TRUE ("RFID读取完成")) -> ()
            n1229 = Wait Until Next ms Multiple(millisecond multiple=u32 500 ("毫秒倍数")) -> ()  [unwired: 1 out]
          }
          frame #7 {
            "rfid工步号" <- 15.0 ("工步号")
          }
        }
      }
      frame 210 {
        n1230 = local read "读取产品ID"() -> (w1897:string)
        n1231 = local write "产品ID"(w1897) -> ()
      }
    }
    n1232 = Wait Until Next ms Multiple(millisecond multiple=u32 50 ("毫秒倍数")) -> ()  [unwired: 1 out]
    n1233 = local read "停止"() -> (w1875:bool)
  }
  n1234 = flat-sequence {
    tunnel: [w1898] -> w4
    tunnel: w4 -> [w1904]
    tunnel: [w1903] -> w3
    tunnel: w3 -> [w1974]
    frame #0 {
      n1235 = call "PCI1240U初始化.vi"() -> ("旋转电机"=→"旋转齿条电机":u32, "电动缸电机"=→"电动缸电机":u32, "DeviceHandle"=→"DeviceHandle":u32, "进给电机"=→"测头机构电机":u32)  [unwired: 6 in, 2 out]
      n1236 = call "PCI8622配置.vi"() -> ("DeviceID"=w1898:i32)  [unwired: 11 in]
    }
    frame #1 {
      n1237 = while {
        tunnel: w1904 -> [w1906]
        tunnel: [w1905] -> w1903
        stop <- "停止" stop-if-true
        n1238 = stacked-sequence {
          tunnel: w1906 -> [_ _ w1950]
          tunnel: [_ _ w1950] -> w1905
          frame #0 {
            n1239 = local read "测头机构电机"() -> (w1915:u32)
            n1240 = Boolean To (0,1)(Boolean="测头机构轴使能") -> (0, 1=w1913:i16)
            n1241 = call <userlib>:"Acm_AxSetSvOn.vi"("OnOff"=w1913, "AxisHandle"=w1915) -> ("AxisHandle"=w1912:u32)  [unwired: 1 in, 2 out]
            n1242 = call "PCI1220U进给轴速度设置.vi"("Change Velocity"="测头机构轴速度(mm/s)", "AxisHandle IN"=w1912) -> ("AxisHandle OUT"=w1910:u32)  [unwired: 9 in]
            n1243 = call "PCI1220U进给轴读取位置.vi"("AxisHandle IN"=w1910) -> ("位置"=→"测头机构轴位置(mm)":dbl)  [unwired: 9 in, 1 out]
          }
          frame #1 {
            n1244 = local read "电动缸电机"() -> (w1925:u32)
            n1245 = local read "旋转齿条电机"() -> (w1924:u32)
            n1246 = Boolean To (0,1)(Boolean="电动缸使能") -> (0, 1=w1929:i16)
            n1247 = Boolean To (0,1)(Boolean="旋转齿条轴使能") -> (0, 1=w1923:i16)
            n1248 = call <userlib>:"Acm_AxSetSvOn.vi"("OnOff"=w1923, "AxisHandle"=w1924) -> ("AxisHandle"=w1926:u32)  [unwired: 1 in, 2 out]
            n1249 = call <userlib>:"Acm_AxSetSvOn.vi"("OnOff"=w1929, "AxisHandle"=w1925) -> ("AxisHandle"=w1928:u32)  [unwired: 1 in, 2 out]
            n1250 = call "PCI1220U扭矩轴速度设置.vi"("Change Velocity"="旋转齿条轴速度(°/s)", "AxisHandle IN"=w1926) -> ("AxisHandle OUT"=w1927:u32)  [unwired: 9 in]
            n1251 = call "PCI1240电动缸速度设置.vi"("Change Velocity"="电动缸速度(mm/s)", "AxisHandle IN"=w1928) -> ("AxisHandle OUT"=w1916:u32)  [unwired: 9 in]
            n1252 = call "PCI1220U扭矩轴读取位置.vi"("AxisHandle IN"=w1927) -> ("位置"=→"旋转齿条轴位置(°)":dbl)  [unwired: 9 in, 1 out]
            n1253 = call "PCI1240电动缸读取位置.vi"("AxisHandle IN"=w1916) -> ("位置"=→"电动缸位置(mm)":dbl)  [unwired: 9 in, 1 out]
          }
          frame #2 {
            w1966 = 0  # nRetSizeWords
            w1967 = 2048  # nReadSizeWords
            # "hDevice"
            n1254 = Initialize Array(u16 0, 2048 ("dimension size")) -> (w1957:u16[])
            n1255 = dll-call lib="PCI8622_32.dll" fn="PCI8622_ReadDeviceProAD_Npt" label="ReadDeviceProAD_Npt"("hDevice"=w1950, "ADBuffer[]"=w1957, "nReadSizeWords"=w1967, "nRetSizeWords"=w1966) -> ("ADBuffer[]"=w1960:u16[])  [unwired: 7 in, 2 out]
            n1256 = Divide(x=w1960, y=65536.01) -> (x/y=w1961:dbl[])
            n1257 = Multiply(x=w1961, y=20) -> (x*y=w1964:dbl[])
            n1258 = Subtract(x=w1964, y=10) -> (x-y=w1956:dbl[])
            n1259 = Decimate 1D Array ("抽取一维数组")(w1956) -> (w1944:dbl[], w1945:dbl[], w1943:dbl[])  [unwired: 5 out]
            n1260 = Add Array Elements(numeric array=w1943) -> (sum=w1954:dbl)
            n1261 = Array Size(array=w1943) -> (size(s)=w1955:i32)
            n1262 = Divide(x=w1954, y=w1955) -> (x/y=w1936:dbl)
            n1263 = Divide(x=w1936, y=5.86) -> (x/y=w1933:dbl)
            n1264 = Multiply(x=4.0, y=w1933) -> (x*y=w1931:dbl)
            n1265 = Add Array Elements(numeric array=w1944) -> (sum=w1953:dbl)
            n1266 = Array Size(array=w1944) -> (size(s)=w1952:i32)
            n1267 = Add Array Elements(numeric array=w1945) -> (sum=w1949:dbl)
            n1268 = Array Size(array=w1945) -> (size(s)=w1951:i32)
            n1269 = Divide(x=w1953, y=w1952) -> (x/y=w1942:dbl)
            n1270 = Divide(x=w1949, y=w1951) -> (x/y=w1939:dbl)
            n1271 = Multiply(x=w1942, y=2.0) -> (x*y=w1937:dbl)
            n1272 = Multiply(x=w1939, y=200.0) -> (x*y=w1938:dbl)
            n1273 = Subtract(x=w1931, y=0.675) -> (x-y=w1934:dbl)
            n1274 = local read "间隙位移比例偏移"() -> (w1971:dbl)
            n1275 = local read "间隙位移零点偏移"() -> (w1970:dbl)
            n1276 = local read "齿条扭矩零点偏移"() -> (w1972:dbl)
            n1277 = local read "齿条扭矩比例偏移"() -> (w1973:dbl)
            n1278 = local read "齿条推拉力比例偏移"() -> (w1969:dbl)
            n1279 = local read "齿条推拉力零点偏移"() -> (w1968:dbl)
            n1280 = call "传感器校订.vi"("零点"=w1972, "比例"=w1973, "传感器"=w1937) -> ("示值"=→"齿条扭矩(Nm)":dbl)  [unwired: 8 in]
            n1281 = call "传感器校订.vi"("零点"=w1970, "比例"=w1971, "传感器"=w1934) -> ("示值"=→"间隙位移(mm)":dbl)  [unwired: 8 in]
            n1282 = call "传感器校订.vi"("零点"=w1968, "比例"=w1969, "传感器"=w1938) -> ("示值"=→"齿条推拉力(N)":dbl)  [unwired: 8 in]
          }
        }
        n1283 = Wait Until Next ms Multiple(millisecond multiple=u32 50 ("毫秒倍数")) -> ()  [unwired: 1 out]
      }
    }
    frame #2 {
      n1284 = dll-call lib="PCI8622_32.dll" fn="PCI8622_StopDeviceProAD" label="StopDeviceProAD"("hDevice"=w1974) -> ("hDevice"=w1975:i32)  [unwired: 4 in, 2 out]
      n1285 = dll-call lib="PCI8622_32.dll" fn="PCI8622_ReleaseDeviceProAD" label="ReleaseDeviceProAD"("hDevice"=w1975) -> ()  [unwired: 5 in, 2 out]
      n1286 = dll-call lib="PCI8622_32.dll" fn="PCI8622_ReleaseDevice" label="ReleaseDevice"("hDevice"=w1974) -> ()  [unwired: 5 in, 2 out]
    }
  }
